vi "Omniax_mDrive_XYZR_MM_BR_RES_2_NC_GR_pxi_Acc.vi"() -> ()   [LabVIEW 2009]
uses:
  <vilib>/Instr/_visa.llb/VISA Configure Serial Port (Instr).vi
panel:
  out "XY Graph 2":cluster{"Y":dbl[], "Y":dbl[]}[](graph)
  out "XY Graph":cluster{"Y":dbl[], "Y":dbl[]}[](graph)
  out "X Scan Duration":dbl
  out "Y Scan Duration":dbl
  out "Z Scan Duration":dbl
  out "R Scan Duration":dbl
  out "R Backlash steps/sec":i32
  out "R Backlash":i32
  out "R Holding Current %":i32
  out "R Run Current %":i32
  out "R offset deg":dbl
  out "R deg/rev":dbl
  out "R steps/rev":u32
  out "R velocity PV step/sec":i32
  out "R MINPOS":i32=-94296
  out "R MAXPOS":i32=-34296
  out "R COM PORT":refnum<visa-resource-name>="COM5"
  in  "R Scan set":bool
  in  "R Scan Velocity SP deg/sec":dbl
  in  "R Scan Length SP deg":dbl
  in  "R Move Set":bool
  out "Reset R Motor Steps":i32
  in  "Reset R Position deg":dbl
  out "R Velocity MVdeg/sec":dbl
  in  "R Velocity SP deg/sec":dbl
  in  "R Position SP deg":dbl
  out "R Position MV deg":dbl
  out "R Scan velocity MV deg/sec":dbl format="%#_6f"
  out "R Scan length MV deg":dbl
  in  "R Scan Length SP steps":i32 min=0 max=6144000 step=100
  in  "R Scan OK":bool
  in  "R Velocity SP step/sec":i32 min=1 max=20000
  in  "R Scan Velocity SP steps/sec":i32=1 min=1 max=102400 step=1
  in  "R Go":bool
  in  "R Step SP":i32=-20000 min=-6144000 max=0 step=500
  out "R Position deg PV":dbl
  out "R Step PV":i32 max=2000
  out "R Backlash corr":bool
  out "R in Motion":bool
  out "R Scan":bool
  out "R in Range":bool
  out "Z COM PORT":refnum<visa-resource-name>="COM5"
  out "Z Backlash steps/sec":i32
  out "Z Backlash":i32
  out "Z Holding Current %":i32
  out "Z Run Current %":i32
  out "Z offset mm":dbl
  out "Z mm/rev":dbl
  out "Z steps/rev":u32
  out "Z  velocity PV step/sec":i32
  out "Z MINPOS":i32=-94296
  out "Z MAXPOS":i32=-34296
  in  "Z Scan set":bool
  in  "Z Scan Velocity SP mm/sec":dbl
  in  "Z Scan Length SP mm":dbl
  in  "Z Move Set":bool
  out "Reset Z Motor Steps":i32
  in  "Reset Z Position mm":dbl
  out "Z Velocity MV mm/sec":dbl
  in  "Z Velocity SP mm/sec":dbl
  in  "Z Position SP mm":dbl
  out "Z Position MV mm":dbl
  out "Z Scan velocity MV mm/sec":dbl format="%#_6f"
  out "Z Scan length MV mm":dbl
  in  "Z Scan Length SP steps":i32 min=0 max=2048000 step=100
  in  "Z Scan OK":bool
  in  "Z Velocity SP step/sec":i32 min=1 max=204800
  in  "Z Scan Velocity SP steps/sec":i32=1 min=1 max=102400 step=1
  in  "Z Go":bool
  in  "Z Step SP":i32=-20000 min=0 max=102400000 step=500
  out "Z Position mm PV":dbl
  out "Z Step PV":i32 max=2000
  out "Z Backlash corr":bool
  out "Z in Motion":bool
  out "Z Scan":bool
  out "Z in Range":bool
  out "Reset X Motor Steps":i32
  in  "Reset X Position mm":dbl
  out "X Backlash corr":bool
  out "X  in Motion":bool
  out "X Scan":bool
  out "X  in Range":bool
  out "X Step PV":i32 max=2000
  out "X Position mm PV":dbl
  out "X velocity PV step/sec":i32
  in  "X Scan set":bool
  in  "X Scan Velocity SP mm/sec":dbl
  in  "X Scan Length SP mm":dbl
  in  "X Move Set":bool
  out "X Velocity MV mm/sec":dbl
  in  "X Velocity SP mm/sec":dbl
  in  "X Position SP mm":dbl
  out "X Position MV mm":dbl
  out "X Scan velocity MV mm/sec":dbl format="%#_6f"
  out "X Scan length MV mm":dbl
  in  "X Scan Length SP steps":i32 min=-2304000 max=2304000 step=100
  in  "X Scan OK":bool
  in  "X Velocity SP step/sec":i32 min=1 max=25600
  in  "X Scan Velocity SP steps/sec":i32=1 min=1 max=102400 step=1
  in  "X Go":bool
  in  "X Step SP":i32=-20000 min=-2304000 max=2304000 step=500
  out "X Backlash steps/sec":i32
  out "X Backlash":i32
  out "X Holding Current %":i32
  out "X Run Current %":i32
  out "X offset mm":dbl
  out "X mm/rev":dbl
  out "X steps/rev":u32
  out "X MAXPOS":i32=-34296
  out "X MINPOS":i32=-94296
  out "X COM PORT":refnum<visa-resource-name>="COM5"
  out "Y Backlash corr":bool
  in  "Y Scan set":bool
  in  "Y Scan Velocity SP mm/sec":dbl
  in  "Y Scan Length SP mm":dbl
  in  "Y Move Set":bool
  out "Y Backlash steps/sec":i32
  out "Y Backlash":i32
  out "Y in Motion":bool
  in  "Reset":bool
  out "Reset Y Motor Steps":i32
  in  "Reset Y Position mm":dbl
  out "Y Velocity MV mm/sec":dbl
  in  "Y Velocity SP mm/sec":dbl
  in  "Y Position SP mm":dbl
  out "Y Position MV mm":dbl
  out "Y Holding Current %":i32
  out "Y Run Current %":i32
  out "Y Scan velocity MV mm/sec":dbl format="%#_6f"
  out "Y Scan length MV mm":dbl
  in  "Scan Cancel":bool
  out "Y Position mm PV":dbl
  out "Y offset mm":dbl
  out "Y mm/rev":dbl
  out "Y steps/rev":u32
  out "Y velocity PV step/sec":i32
  in  "Y Scan Length SP steps":i32 min=-2304000 max=2304000 step=100
  out "Y Scan":bool
  in  "Y Scan OK":bool
  in  "Scan Go":bool
  in  "Y Velocity SP step/sec":i32 min=1 max=25600
  in  "Y Scan Velocity SP steps/sec":i32=1 min=1 max=102400 step=1
  in  "Stop":bool
  out "Y in Range":bool
  out "Y Step PV":i32 max=2000
  in  "Y Go":bool
  in  "Y Step SP":i32=-20000 min=-2304000 max=2304000 step=500
  out "Y MINPOS":i32=-94296
  out "Y MAXPOS":i32=-34296
  out "Y COM PORT":refnum<visa-resource-name>="COM5"
  # "L"
  # "M"
  # "B"
  # "S"
  # "MX"
  # "MY"
  # "MZ"
  # "MR"
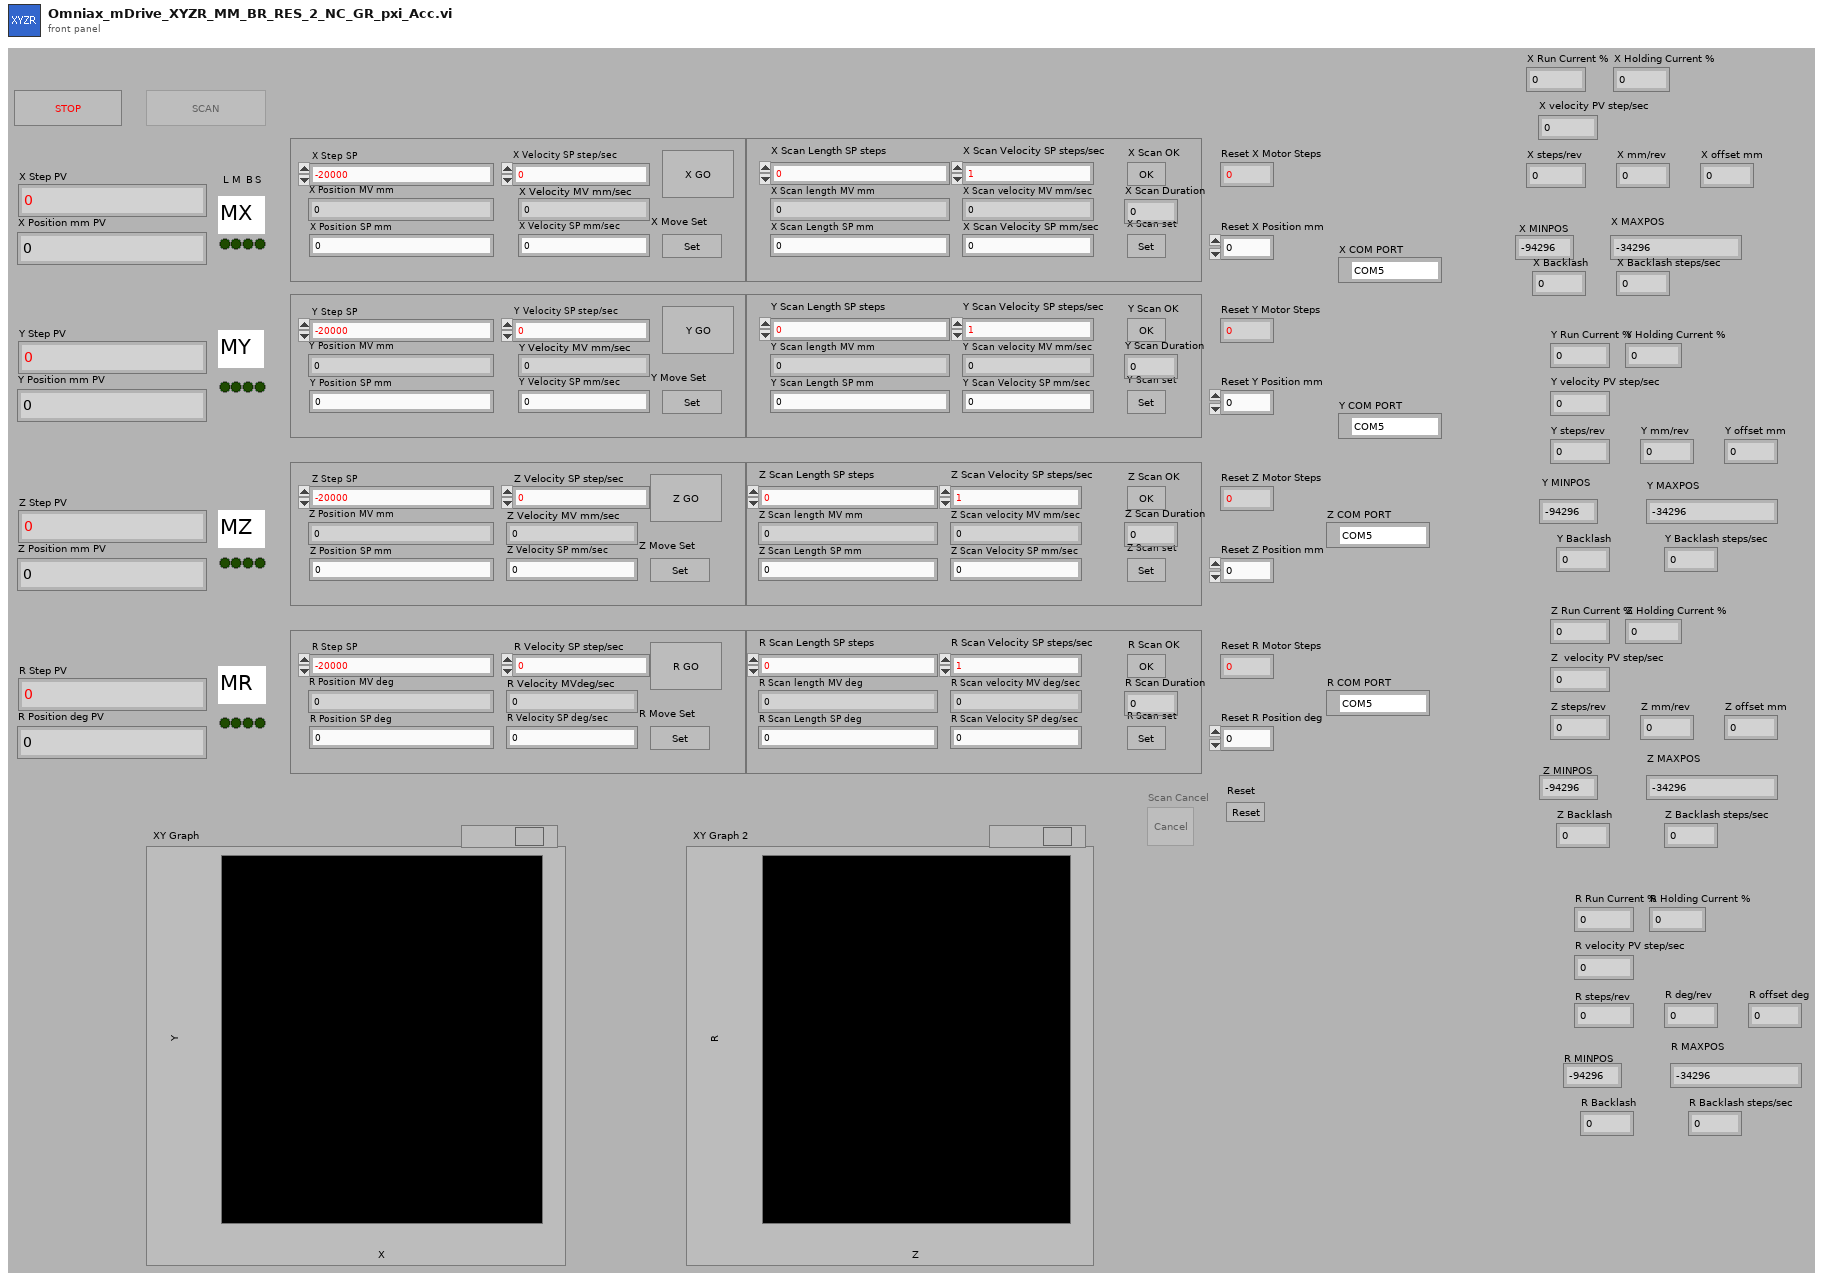
[diagram p1: front panel]
types:
  T1 = enum8{"Enabled", "Disabled", "Disabled and Grayed Out"}
  T2 = enum16{"Stop", "Reset", "Run Current", "Holding Current", "Accel Rate", "Decel Rate", "Move to Relative Position", "Move to Absolute Position", "Echo Mode", "Print Parameter", "Send String", "Microstep Resolution", "Set Current Position", "Max Velocity"}
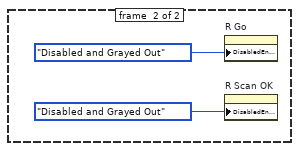
[diagram p2: hidden frame]
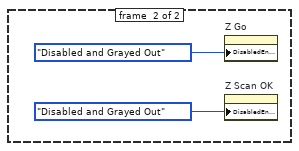
[diagram p5: hidden frame]
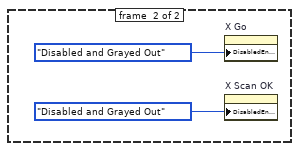
[diagram p8: hidden frame]
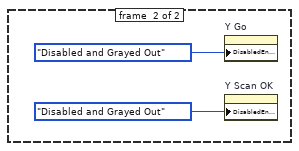
[diagram p11: hidden frame]
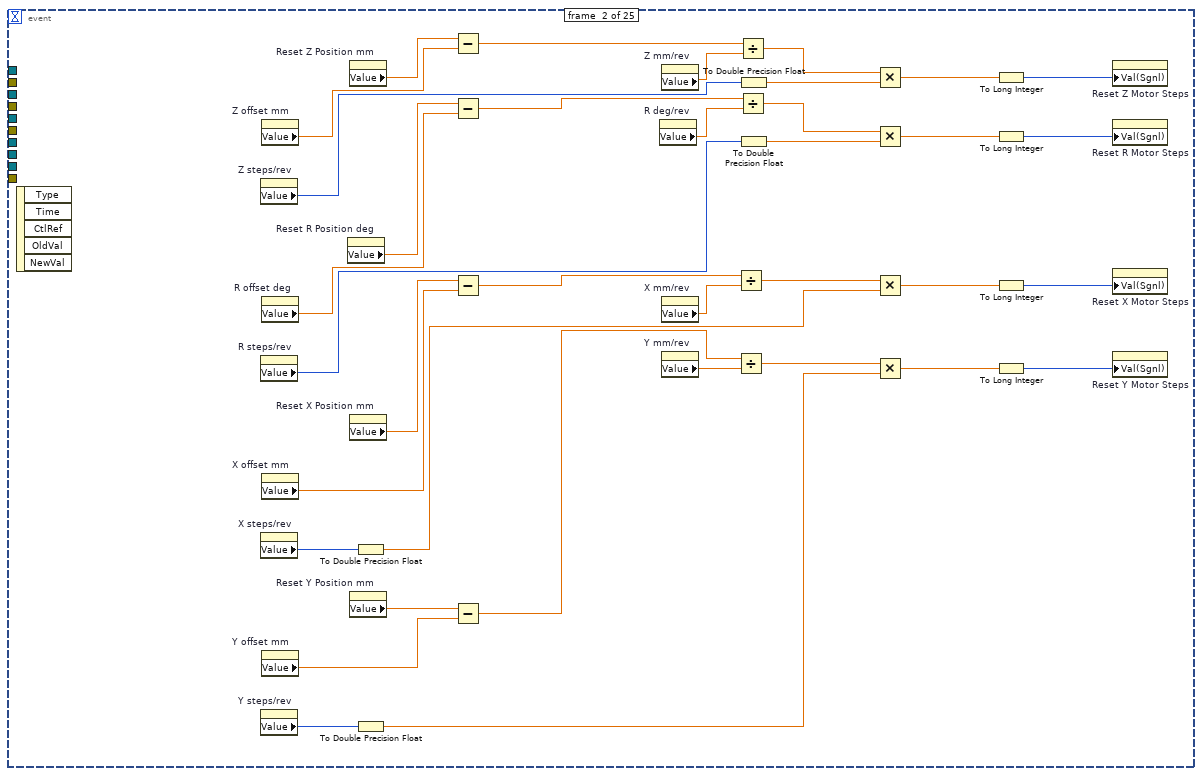
[diagram p14: hidden frame]
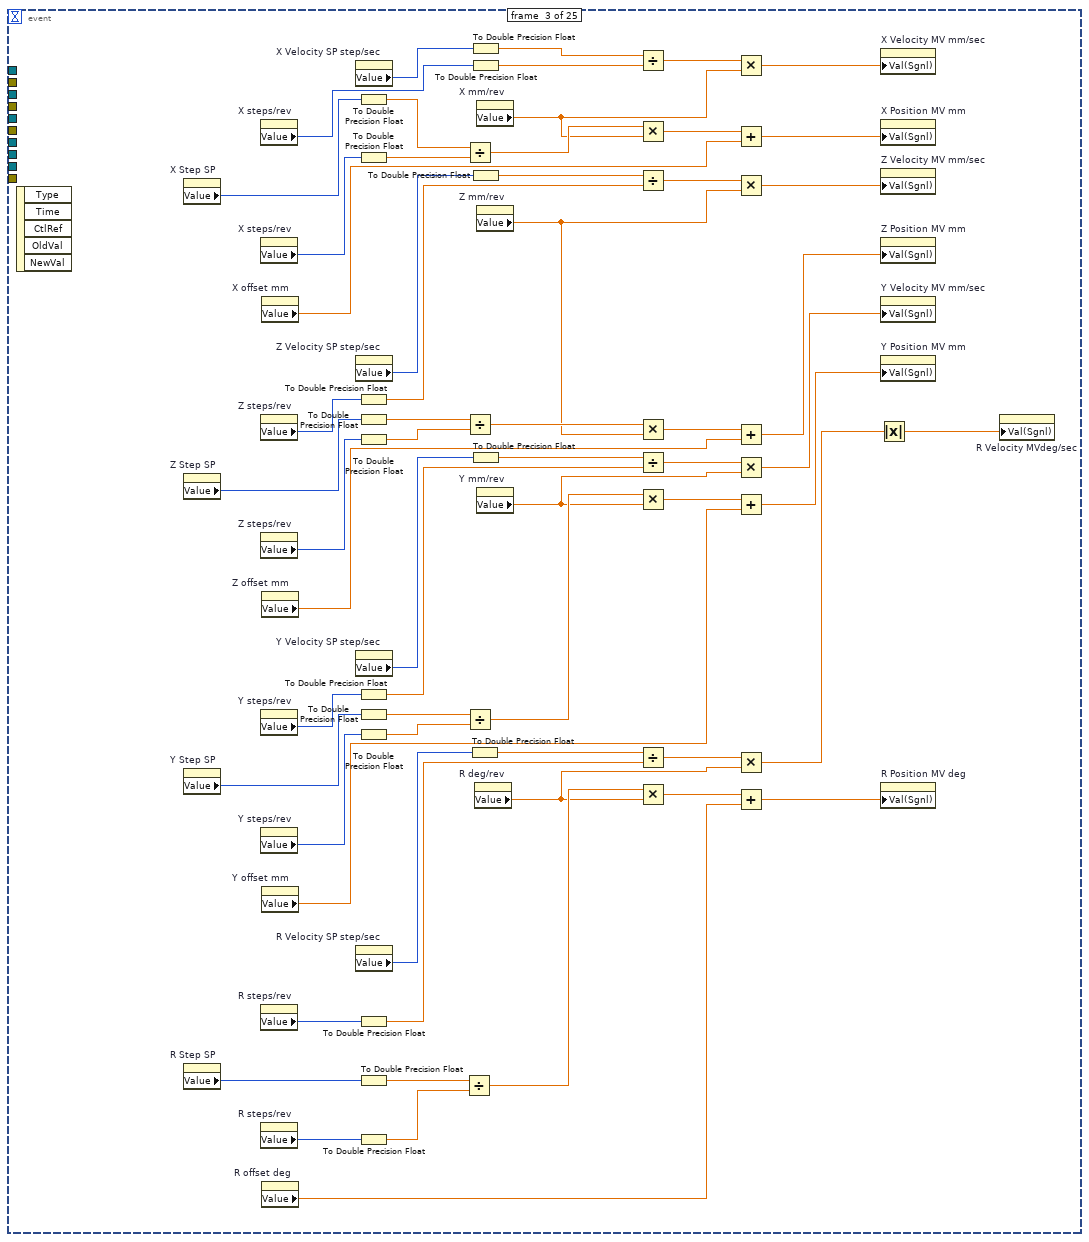
[diagram p15: hidden frame]
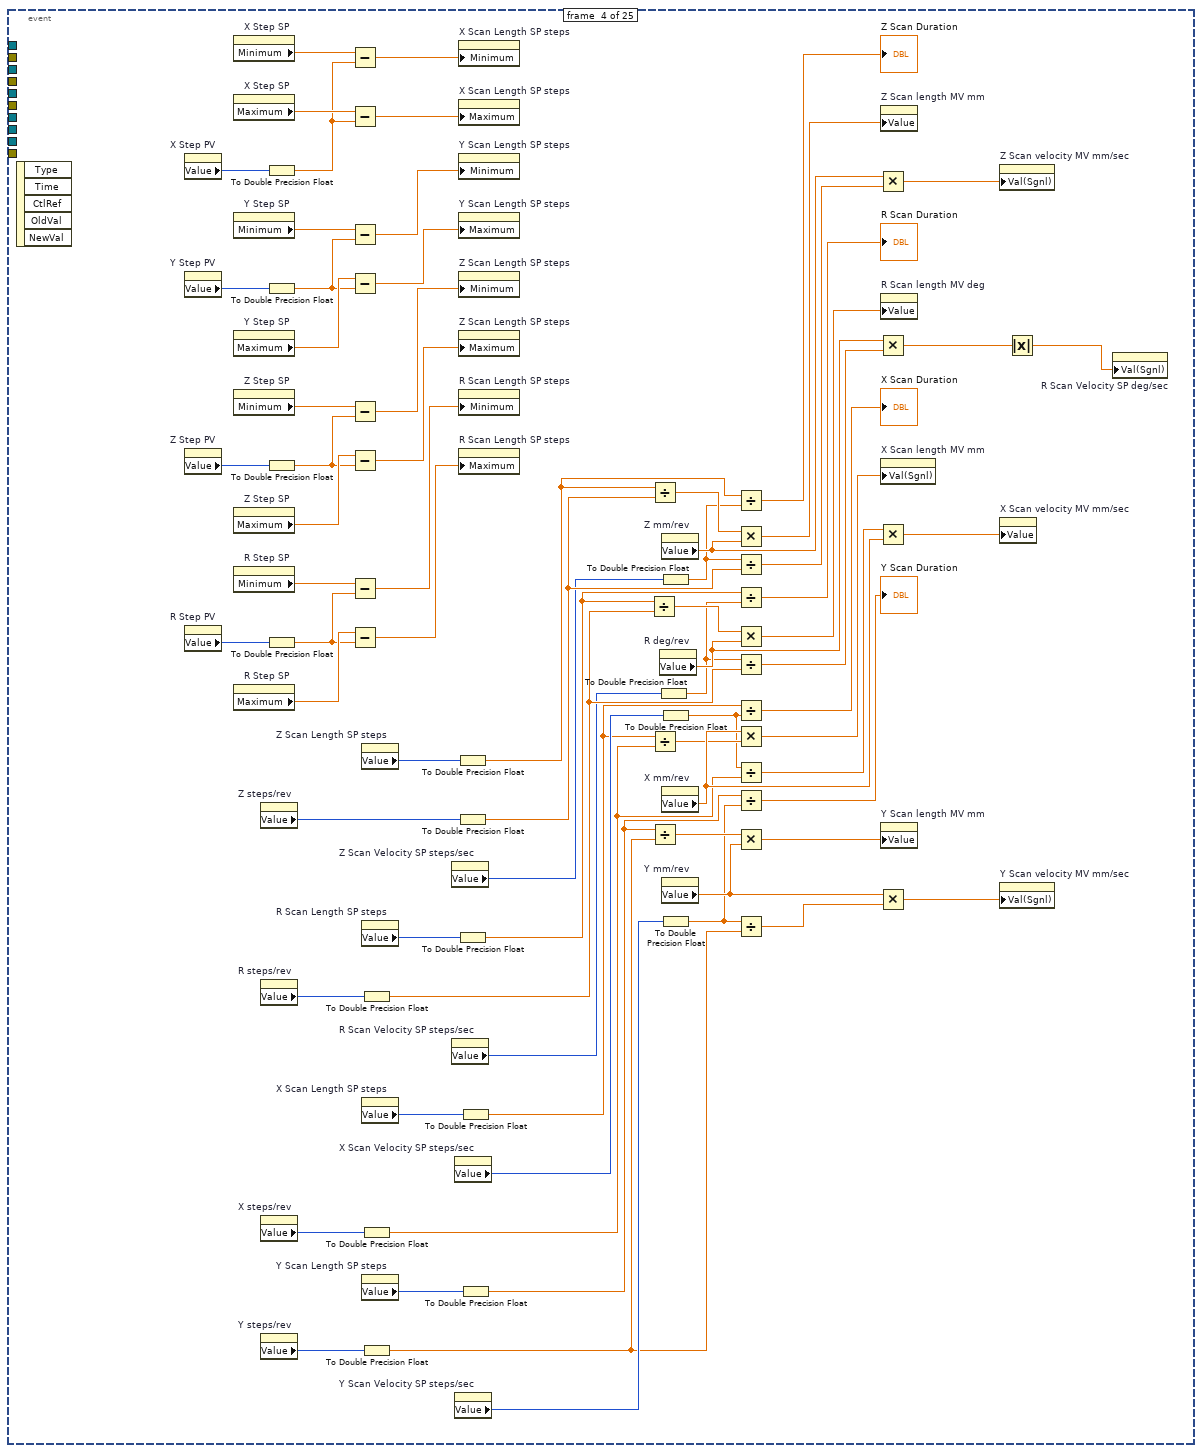
[diagram p16: hidden frame]
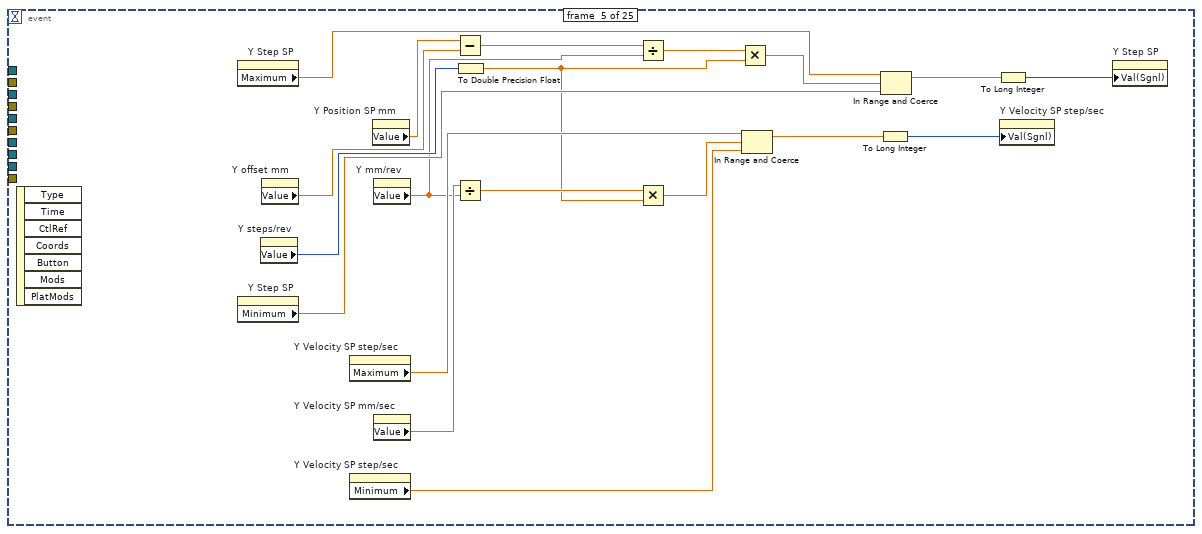
[diagram p17: hidden frame]
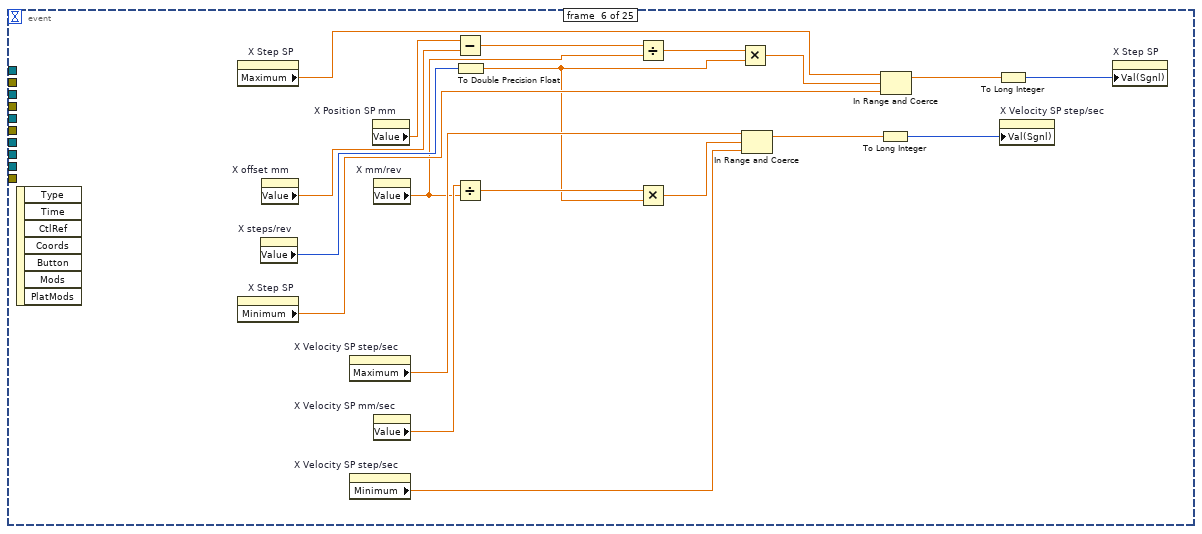
[diagram p18: hidden frame]
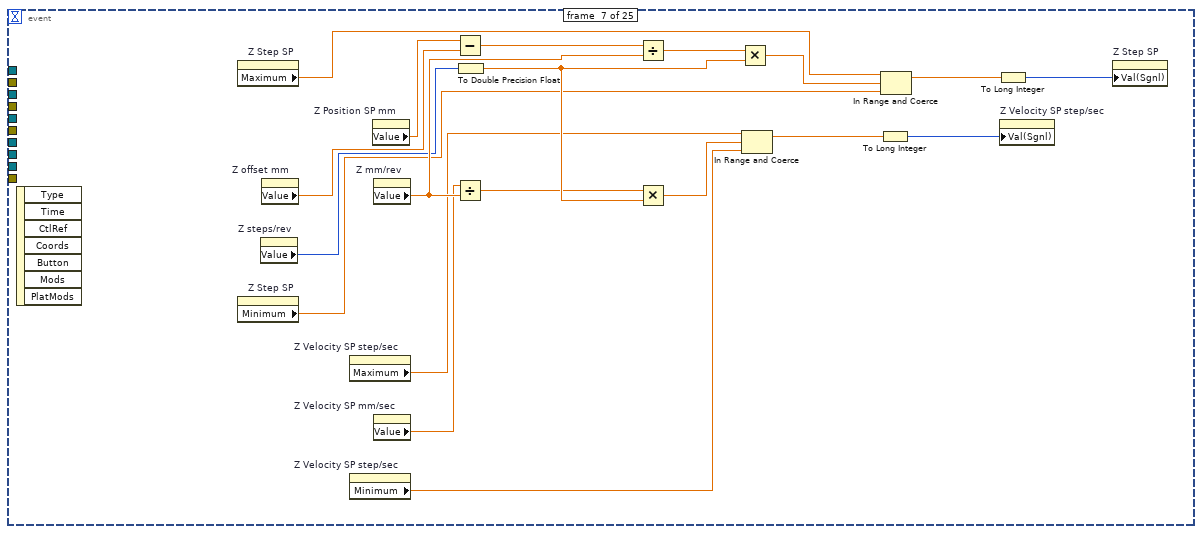
[diagram p19: hidden frame]
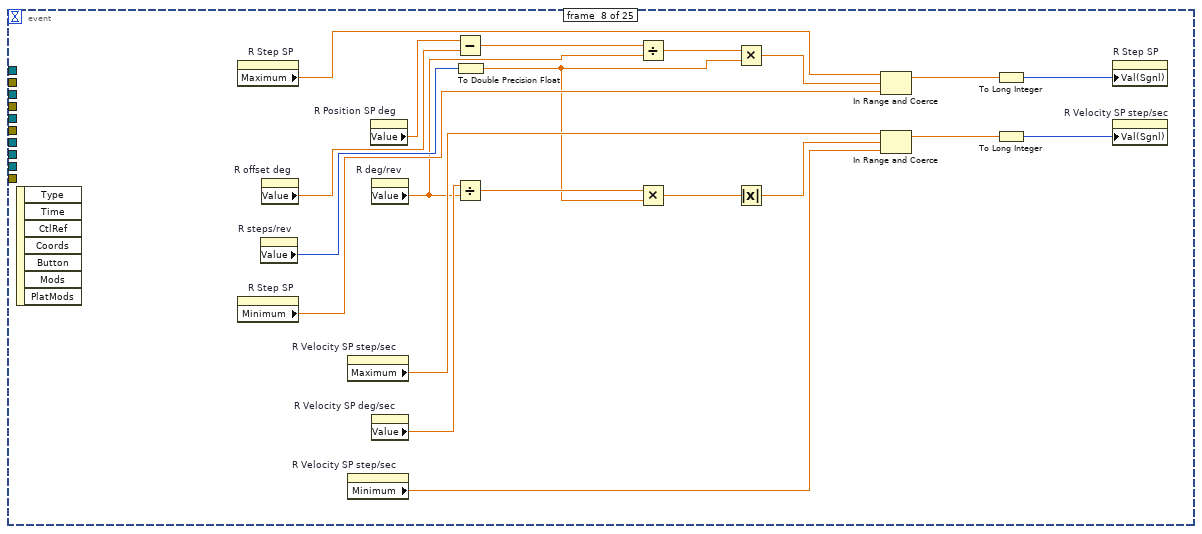
[diagram p20: hidden frame]
diagram:
  w29 = refnum<visa-resource-name> "COM7" ("COM PORT")
  w31 = u16 0 items=["None", "XON/XOFF", "RTS/CTS", "XON/XOFF & RTS/CTS", "DTR/DSR", "XON/XOFF & DTR/DSR"] ("flow control (0:none)")
  w32 = u16 10 items=["1.0"=10, "1.5"=15, "2.0"=20] ("stop bits (10: 1 bit)")
  w62 = refnum<visa-resource-name> "COM6" ("COM PORT")
  w64 = u16 0 items=["None", "XON/XOFF", "RTS/CTS", "XON/XOFF & RTS/CTS", "DTR/DSR", "XON/XOFF & DTR/DSR"] ("flow control (0:none)")
  w65 = u16 10 items=["1.0"=10, "1.5"=15, "2.0"=20] ("stop bits (10: 1 bit)")
  w75 = refnum<visa-resource-name> "COM4" ("COM PORT")
  w77 = u16 0 items=["None", "XON/XOFF", "RTS/CTS", "XON/XOFF & RTS/CTS", "DTR/DSR", "XON/XOFF & DTR/DSR"] ("flow control (0:none)")
  w78 = u16 10 items=["1.0"=10, "1.5"=15, "2.0"=20] ("stop bits (10: 1 bit)")
  w100 = refnum<visa-resource-name> "COM5" ("COM PORT")
  w102 = u16 0 items=["None", "XON/XOFF", "RTS/CTS", "XON/XOFF & RTS/CTS", "DTR/DSR", "XON/XOFF & DTR/DSR"] ("flow control (0:none)")
  w103 = u16 10 items=["1.0"=10, "1.5"=15, "2.0"=20] ("stop bits (10: 1 bit)")
  # "Stop bits"
  # "Stop bits"
  # "Stop bits"
  # "Stop bits"
  n1 = flat-sequence {
    frame #0 {
      w112 = -3.0 ("R deg/rev")
      w110 = u32 51200 ("step/rev")
      w114 = 20000 ("Value (Signaling)")
      n2 = To Double Precision Float(number=w114) -> (double precision float=w116:dbl)
      n3 = To Double Precision Float(number=w110) -> (double precision float=w111:dbl)
      n4 = property on="R Velocity SP step/sec" class="DigNum (strict)"("Val(Sgnl)"=w114) -> ()  [unwired: 2 in, 2 out]
      n5 = property on="R Velocity SP step/sec" class="DigNum (strict)"("Minimum"=1.0 ("Data Entry Limits:Minimum")) -> ()  [unwired: 2 in, 2 out]
      n6 = Divide(x=w116, y=w111) -> (x/y=w115:dbl)
      n7 = property on="R Velocity SP step/sec" class="DigNum (strict)"("Maximum"=w116) -> ()  [unwired: 2 in, 2 out]
      n8 = Multiply(x=w115, y=w112) -> (x*y=w113:dbl)
      n9 = Absolute Value(x=w113) -> (abs(x)=w107:dbl)
      n10 = property on="R Velocity SP deg/sec" class="DigNum (strict)"("Val(Sgnl)"=w107) -> ()  [unwired: 2 in, 2 out]
      "R offset deg" <- 0.0 ("R offset deg")
      "R deg/rev" <- w112
      "R steps/rev" <- w110
    }
  }
  n11 = flat-sequence {
    frame #0 {
      w118 = 0.2 ("Z mm/rev")
      w117 = u32 51200 ("step/rev")
      w119 = 204800 ("Value (Signaling)")
      n12 = To Double Precision Float(number=w119) -> (double precision float=w123:dbl)
      n13 = To Double Precision Float(number=w117) -> (double precision float=w122:dbl)
      n14 = property on="Z Velocity SP step/sec" class="DigNum (strict)"("Val(Sgnl)"=w119) -> ()  [unwired: 2 in, 2 out]
      n15 = property on="Z Velocity SP step/sec" class="DigNum (strict)"("Minimum"=1.0 ("Data Entry Limits:Minimum")) -> ()  [unwired: 2 in, 2 out]
      n16 = Divide(x=w123, y=w122) -> (x/y=w120:dbl)
      n17 = property on="Z Velocity SP step/sec" class="DigNum (strict)"("Maximum"=w123) -> ()  [unwired: 2 in, 2 out]
      n18 = Multiply(x=w120, y=w118) -> (x*y=w121:dbl)
      n19 = property on="Z Velocity SP mm/sec" class="DigNum (strict)"("Val(Sgnl)"=w121) -> ()  [unwired: 2 in, 2 out]
      "Z offset mm" <- 0.0 ("Z offset mm")
      "Z mm/rev" <- w118
      "Z steps/rev" <- w117
    }
  }
  n20 = flat-sequence {
    frame #0 {
      n21 = property on="X Backlash corr" class="Bool (strict)"("Val(Sgnl)"=FALSE ("Value (Signaling)")) -> ()  [unwired: 2 in, 2 out]
      n22 = property on="R Backlash corr" class="Bool (strict)"("Val(Sgnl)"=FALSE ("Value (Signaling)")) -> ()  [unwired: 2 in, 2 out]
      n23 = property on="Z Backlash corr" class="Bool (strict)"("Val(Sgnl)"=FALSE ("Value (Signaling)")) -> ()  [unwired: 2 in, 2 out]
      n24 = property on="Y Backlash corr" class="Bool (strict)"("Val(Sgnl)"=FALSE ("Value (Signaling)")) -> ()  [unwired: 2 in, 2 out]
      "Z Backlash steps/sec" <- 25600 ("Z Backlash steps/sec")
      "Z Backlash" <- -12800 ("Z Backlash")
      "X Backlash steps/sec" <- 25600 ("Value (Signaling)")
      "X Backlash" <- -5120 ("Backlash2")
      "Y Backlash" <- -5120 ("Backlash2")
      "Y Backlash steps/sec" <- 25600 ("Value (Signaling)")
      "R Backlash steps/sec" <- 6400 ("R Backlash steps/sec")
      "R Backlash" <- -12800 ("R Backlash")
    }
  }
  n25 = flat-sequence {
    frame #0 {
      "Z Holding Current %" <- 20 ("Z Holding Current %")
      "Z Run Current %" <- 40 ("Z Run Current %")
      "X Run Current %" <- 40 ("Run Current %")
      "X Holding Current %" <- 20 ("Holding Current %")
      "Y Run Current %" <- 40 ("Run Current %")
      "Y Holding Current %" <- 20 ("Holding Current %")
      "R Holding Current %" <- 20 ("R Holding Current %")
      "R Run Current %" <- 100 ("R Run Current %")
    }
  }
  n26 = flat-sequence {
    frame #0 {
      n27 = property on="Y Scan" class="Bool (strict)"("Val(Sgnl)"=FALSE ("Value (Signaling)")) -> ()  [unwired: 2 in, 2 out]
      n28 = property on="R Velocity SP deg/sec" class="DigNum (strict)"("Val(Sgnl)"=0.1 ("Value (Signaling)")) -> ()  [unwired: 2 in, 2 out]
      n29 = property on="X Scan Velocity SP mm/sec" class="DigNum (strict)"("Val(Sgnl)"=0.1 ("Value (Signaling)")) -> ()  [unwired: 2 in, 2 out]
      n30 = property on="Z Scan" class="Bool (strict)"("Val(Sgnl)"=FALSE ("Value (Signaling)")) -> ()  [unwired: 2 in, 2 out]
      n31 = property on="X Scan" class="Bool (strict)"("Val(Sgnl)"=FALSE ("Value (Signaling)")) -> ()  [unwired: 2 in, 2 out]
      n32 = property on="Z Scan Velocity SP mm/sec" class="DigNum (strict)"("Val(Sgnl)"=0.1 ("Value (Signaling)")) -> ()  [unwired: 2 in, 2 out]
      n33 = property on="R Scan" class="Bool (strict)"("Val(Sgnl)"=FALSE ("Value (Signaling)")) -> ()  [unwired: 2 in, 2 out]
      n34 = property on="Y Scan Velocity SP mm/sec" class="DigNum (strict)"("Val(Sgnl)"=0.1 ("Value (Signaling)")) -> ()  [unwired: 2 in, 2 out]
      n35 = property on="Scan Cancel" class="Bool"("DisabledEnum"=T1."Disabled and Grayed Out" ("Disabled")) -> ()  [unwired: 2 in, 2 out]
      n36 = property on="Scan Go" class="Bool"("DisabledEnum"=T1."Disabled and Grayed Out" ("Disabled")) -> ()  [unwired: 2 in, 2 out]
    }
  }
  n37 = flat-sequence {
    frame #0 {
      w158 = 0.2 ("MM/rev")
      w161 = u32 51200 ("step/rev")
      w156 = 25600 ("Value (Signaling)")
      # "a=1000000"
      n38 = To Double Precision Float(number=w156) -> (double precision float=w162:dbl)
      n39 = To Double Precision Float(number=w161) -> (double precision float=w160:dbl)
      n40 = property on="X Velocity SP step/sec" class="DigNum (strict)"("Minimum"=1.0 ("Data Entry Limits:Minimum")) -> ()  [unwired: 2 in, 2 out]
      n41 = property on="X Velocity SP step/sec" class="DigNum (strict)"("Val(Sgnl)"=w156) -> ()  [unwired: 2 in, 2 out]
      n42 = Divide(x=w162, y=w160) -> (x/y=w157:dbl)
      n43 = property on="X Velocity SP step/sec" class="DigNum (strict)"("Maximum"=w162) -> ()  [unwired: 2 in, 2 out]
      n44 = Multiply(x=w157, y=w158) -> (x*y=w159:dbl)
      n45 = property on="X Velocity SP mm/sec" class="DigNum (strict)"("Val(Sgnl)"=w159) -> ()  [unwired: 2 in, 2 out]
      "X offset mm" <- 0.0 ("offset")
      "X steps/rev" <- w161
      "X mm/rev" <- w158
    }
  }
  n46 = flat-sequence {
    frame #0 {
      w167 = 0.2 ("MM/rev")
      w170 = u32 51200 ("step/rev")
      w165 = 25600 ("Value (Signaling)")
      n47 = To Double Precision Float(number=w165) -> (double precision float=w171:dbl)
      n48 = To Double Precision Float(number=w170) -> (double precision float=w169:dbl)
      n49 = property on="Y Velocity SP step/sec" class="DigNum (strict)"("Minimum"=1.0 ("Data Entry Limits:Minimum")) -> ()  [unwired: 2 in, 2 out]
      n50 = property on="Y Velocity SP step/sec" class="DigNum (strict)"("Val(Sgnl)"=w165) -> ()  [unwired: 2 in, 2 out]
      n51 = Divide(x=w171, y=w169) -> (x/y=w166:dbl)
      n52 = property on="Y Velocity SP step/sec" class="DigNum (strict)"("Maximum"=w171) -> ()  [unwired: 2 in, 2 out]
      n53 = Multiply(x=w166, y=w167) -> (x*y=w168:dbl)
      n54 = property on="Y Velocity SP mm/sec" class="DigNum (strict)"("Val(Sgnl)"=w168) -> ()  [unwired: 2 in, 2 out]
      "Y offset mm" <- 0.0 ("offset")
      "Y steps/rev" <- w170
      "Y mm/rev" <- w167
    }
  }
  n55 = call-poly "VISA Configure Serial Port"("VISA resource name"=w100, "timeout (10sec)"=u32 10000, "baud rate (9600)"=u32 9600, "data bits (8)"=u16 8, "parity (0:none)"=enum16{"None", "Odd", "Even", "Mark", "Space"}."None", "stop bits (10: 1 bit)"=w103, "flow control (0:none)"=w102) -> ("VISA resource name out"=w93:refnum<visa-resource-name>, "error out"=w92:errorcluster)  [unwired: 7 in]
  n56 = flat-sequence {
    tunnel: w92 -> [w175]
    tunnel: w93 -> [w177]
    tunnel: [w176] -> w10
    tunnel: [w174] -> w8
    tunnel: w10 -> [w183]
    tunnel: [w184] -> w9
    tunnel: w8 -> [w180]
    tunnel: [w182] -> w7
    tunnel: [w193] -> w91
    tunnel: [w195] -> w89
    tunnel: w9 -> [w194]
    tunnel: w7 -> [w196]
    tunnel: w91 -> [w203]
    tunnel: [w202] -> w90
    tunnel: w89 -> [w200]
    tunnel: [w201] -> w88
    tunnel: [w213] -> w95
    tunnel: [w214] -> w94
    tunnel: w90 -> [w212]
    tunnel: w88 -> [w211]
    tunnel: w95 -> [w224]
    tunnel: w94 -> [w223]
    tunnel: [w226] -> w61
    tunnel: [w225] -> w60
    tunnel: [w220] -> w59
    tunnel: [w231] -> w98
    tunnel: [w232] -> w99
    tunnel: w61 -> [w232]
    tunnel: w60 -> [w231]
    tunnel: w59 -> [w227]
    frame #0 {
      n57 = call "mDrive Send Command.vi"("error in (no error)"=w175, "Extra"="EM=2", "Command"=T2."Send String", "VISA resource name"=w177) -> ("error out"=w174:errorcluster, "VISA resource name out"=w176:refnum<visa-resource-name>)  [unwired: 3 in, 1 out]
    }
    frame #1 {
      n58 = Number To Decimal String(number=1000000) -> (decimal integer string=w185:string)  [unwired: 1 in]
      n59 = call "mDrive Send Command.vi"("error in (no error)"=w180, "Extra"=w185, "Command"=T2."Accel Rate", "VISA resource name"=w183) -> ("error out"=w181:errorcluster, "VISA resource name out"=w189:refnum<visa-resource-name>)  [unwired: 3 in, 1 out]
      n60 = call "mDrive Send Command.vi"("error in (no error)"=w181, "Extra"=w185, "Command"=T2."Decel Rate", "VISA resource name"=w189) -> ("error out"=w182:errorcluster, "VISA resource name out"=w184:refnum<visa-resource-name>)  [unwired: 3 in, 1 out]
    }
    frame #2 {
      # "Run Current %"
      n61 = property on="Y Run Current %" class="DigNum (strict)"() -> ("Value"=w191:i32)  [unwired: 2 in, 2 out]
      n62 = Number To Decimal String(number=w191) -> (decimal integer string=w192:string)  [unwired: 1 in]
      n63 = call "mDrive Send Command.vi"("error in (no error)"=w196, "Extra"=w192, "Command"=T2."Run Current", "VISA resource name"=w194) -> ("error out"=w195:errorcluster, "VISA resource name out"=w193:refnum<visa-resource-name>)  [unwired: 3 in, 1 out]
    }
    frame #3 {
      # "Holding Current %"
      n64 = property on="Y Holding Current %" class="DigNum (strict)"() -> ("Value"=w198:i32)  [unwired: 2 in, 2 out]
      n65 = Number To Decimal String(number=w198) -> (decimal integer string=w199:string)  [unwired: 1 in]
      n66 = call "mDrive Send Command.vi"("error in (no error)"=w200, "Extra"=w199, "Command"=T2."Holding Current", "VISA resource name"=w203) -> ("error out"=w201:errorcluster, "VISA resource name out"=w202:refnum<visa-resource-name>)  [unwired: 3 in, 1 out]
    }
    frame #4 {
      # "Print Velocity Ma"
      # "Velocity Max"
      n67 = property on="Y Velocity SP step/sec" class="DigNum (strict)"() -> ("Value"=w210:i32)  [unwired: 2 in, 2 out]
      n68 = Number To Decimal String(number=w210) -> (decimal integer string=w209:string)  [unwired: 1 in]
      n69 = call "mDrive Send Command.vi"("error in (no error)"=w211, "Extra"=w209, "Command"=T2."Max Velocity", "VISA resource name"=w212) -> ("error out"=w207:errorcluster, "VISA resource name out"=w217:refnum<visa-resource-name>)  [unwired: 3 in, 1 out]
      n70 = call "mDrive Send Command.vi"("error in (no error)"=w207, "Extra"="VM", "Command"=T2."Print Parameter", "VISA resource name"=w217) -> ("error out"=w214:errorcluster, "read buffer"=w215:string, "VISA resource name out"=w213:refnum<visa-resource-name>)  [unwired: 3 in]
      n71 = Decimal String To Number(string=w215, offset=0) -> (number=w208:i32)  [unwired: 1 in, 1 out]
      n72 = property on="Y scan velocity MV step/sec" class="DigNum (strict)"("Val(Sgnl)"=w208) -> ()  [unwired: 2 in, 2 out]
    }
    frame #5 {
      # "PRINT POSITION"
      n73 = call "mDrive Send Command.vi"("error in (no error)"=w223, "Extra"="P", "Command"=T2."Print Parameter", "VISA resource name"=w224) -> ("error out"=w225:errorcluster, "read buffer"=w222:string, "VISA resource name out"=w226:refnum<visa-resource-name>)  [unwired: 3 in]
      n74 = Decimal String To Number(string=w222, offset=0) -> (number=w220:i32)  [unwired: 1 in, 1 out]
    }
    frame #6 {
      w229 = -2304000 ("lower limit")
      w230 = 2304000 ("upper limit")
      n75 = property on="Y Step SP" class="DigNum (strict)"("Val(Sgnl)"=w227) -> ()  [unwired: 2 in, 2 out]
      n76 = property on="Y Step SP" class="DigNum (strict)"("Maximum"=w230) -> ()  [unwired: 2 in, 2 out]
      n77 = In Range and Coerce(upper limit=w230, x=w227, lower limit=w229) -> (In Range?=w228:bool)  [unwired: 1 out]
      n78 = property on="Y Step SP" class="DigNum (strict)"("Minimum"=w229) -> ()  [unwired: 2 in, 2 out]
      n79 = property on="Y in Range" class="Bool (strict)"("Val(Sgnl)"=w228) -> ()  [unwired: 2 in, 2 out]
      "Y MINPOS" <- w229
      "Y MAXPOS" <- w230
    }
  }
  n80 = call-poly "VISA Configure Serial Port"("VISA resource name"=w75, "timeout (10sec)"=u32 10000, "baud rate (9600)"=u32 9600, "data bits (8)"=u16 8, "parity (0:none)"=enum16{"None", "Odd", "Even", "Mark", "Space"}."None", "stop bits (10: 1 bit)"=w78, "flow control (0:none)"=w77) -> ("VISA resource name out"=w74:refnum<visa-resource-name>, "error out"=w73:errorcluster)  [unwired: 7 in]
  n81 = call-poly "VISA Configure Serial Port"("VISA resource name"=w29, "timeout (10sec)"=u32 10000, "baud rate (9600)"=u32 9600, "data bits (8)"=u16 8, "parity (0:none)"=enum16{"None", "Odd", "Even", "Mark", "Space"}."None", "stop bits (10: 1 bit)"=w32, "flow control (0:none)"=w31) -> ("VISA resource name out"=w28:refnum<visa-resource-name>, "error out"=w27:errorcluster)  [unwired: 7 in]
  n82 = call-poly "VISA Configure Serial Port"("VISA resource name"=w62, "timeout (10sec)"=u32 10000, "baud rate (9600)"=u32 9600, "data bits (8)"=u16 8, "parity (0:none)"=enum16{"None", "Odd", "Even", "Mark", "Space"}."None", "stop bits (10: 1 bit)"=w65, "flow control (0:none)"=w64) -> ("VISA resource name out"=w46:refnum<visa-resource-name>, "error out"=w45:errorcluster)  [unwired: 7 in]
  n83 = flat-sequence {
    tunnel: w45 -> [w233]
    tunnel: w46 -> [w236]
    tunnel: [w235] -> w6
    tunnel: [w234] -> w4
    tunnel: w6 -> [w246]
    tunnel: [w241] -> w5
    tunnel: w4 -> [w245]
    tunnel: [w245] -> w3
    tunnel: [w250] -> w55
    tunnel: [w252] -> w54
    tunnel: w5 -> [w251]
    tunnel: w3 -> [w253]
    tunnel: w55 -> [w260]
    tunnel: [w259] -> w53
    tunnel: w54 -> [w257]
    tunnel: [w258] -> w52
    tunnel: [w270] -> w51
    tunnel: [w271] -> w50
    tunnel: w53 -> [w269]
    tunnel: w52 -> [w268]
    tunnel: w51 -> [w281]
    tunnel: w50 -> [w280]
    tunnel: [w283] -> w49
    tunnel: [w282] -> w48
    tunnel: [w277] -> w47
    tunnel: [w290] -> w25
    tunnel: [w291] -> w26
    tunnel: w49 -> [w291]
    tunnel: w48 -> [w290]
    tunnel: w47 -> [w288]
    frame #0 {
      n84 = call "mDrive Send Command.vi"("error in (no error)"=w233, "Extra"="EM=2", "Command"=T2."Send String", "VISA resource name"=w236) -> ("error out"=w234:errorcluster, "VISA resource name out"=w235:refnum<visa-resource-name>)  [unwired: 3 in, 1 out]
    }
    frame #1 {
      n85 = Number To Decimal String(number=1000000) -> (decimal integer string=w239:string)  [unwired: 1 in]
      n86 = call "mDrive Send Command.vi"("Extra"=w239, "Command"=T2."Accel Rate", "VISA resource name"=w246) -> ("VISA resource name out"=w244:refnum<visa-resource-name>)  [unwired: 4 in, 2 out]
      n87 = call "mDrive Send Command.vi"("Extra"=w239, "Command"=T2."Decel Rate", "VISA resource name"=w244) -> ("VISA resource name out"=w241:refnum<visa-resource-name>)  [unwired: 4 in, 2 out]
    }
    frame #2 {
      # "Run Current %"
      n88 = property on="Z Run Current %" class="DigNum (strict)"() -> ("Value"=w248:i32)  [unwired: 2 in, 2 out]
      n89 = Number To Decimal String(number=w248) -> (decimal integer string=w249:string)  [unwired: 1 in]
      n90 = call "mDrive Send Command.vi"("error in (no error)"=w253, "Extra"=w249, "Command"=T2."Run Current", "VISA resource name"=w251) -> ("error out"=w252:errorcluster, "VISA resource name out"=w250:refnum<visa-resource-name>)  [unwired: 3 in, 1 out]
    }
    frame #3 {
      # "Holding Current %"
      n91 = property on="Z Run Current %" class="DigNum (strict)"() -> ("Value"=w255:i32)  [unwired: 2 in, 2 out]
      n92 = Number To Decimal String(number=w255) -> (decimal integer string=w256:string)  [unwired: 1 in]
      n93 = call "mDrive Send Command.vi"("error in (no error)"=w257, "Extra"=w256, "Command"=T2."Holding Current", "VISA resource name"=w260) -> ("error out"=w258:errorcluster, "VISA resource name out"=w259:refnum<visa-resource-name>)  [unwired: 3 in, 1 out]
    }
    frame #4 {
      # "Print Velocity Ma"
      # "Velocity Max"
      n94 = property on="Z Velocity SP step/sec" class="DigNum (strict)"() -> ("Value"=w267:i32)  [unwired: 2 in, 2 out]
      n95 = Number To Decimal String(number=w267) -> (decimal integer string=w266:string)  [unwired: 1 in]
      n96 = call "mDrive Send Command.vi"("error in (no error)"=w268, "Extra"=w266, "Command"=T2."Max Velocity", "VISA resource name"=w269) -> ("error out"=w264:errorcluster, "VISA resource name out"=w274:refnum<visa-resource-name>)  [unwired: 3 in, 1 out]
      n97 = call "mDrive Send Command.vi"("error in (no error)"=w264, "Extra"="VM", "Command"=T2."Print Parameter", "VISA resource name"=w274) -> ("error out"=w271:errorcluster, "read buffer"=w272:string, "VISA resource name out"=w270:refnum<visa-resource-name>)  [unwired: 3 in]
      n98 = Decimal String To Number(string=w272, offset=0) -> (number=w265:i32)  [unwired: 1 in, 1 out]
      n99 = property on="Z  velocity PV step/sec" class="DigNum (strict)"("Val(Sgnl)"=w265) -> ()  [unwired: 2 in, 2 out]
    }
    frame #5 {
      # "PRINT POSITION"
      n100 = call "mDrive Send Command.vi"("error in (no error)"=w280, "Extra"="P", "Command"=T2."Print Parameter", "VISA resource name"=w281) -> ("error out"=w282:errorcluster, "read buffer"=w279:string, "VISA resource name out"=w283:refnum<visa-resource-name>)  [unwired: 3 in]
      n101 = Decimal String To Number(string=w279, offset=0) -> (number=w277:i32)  [unwired: 1 in, 1 out]
    }
    frame #6 {
      n102 = property on="Z Step SP" class="DigNum (strict)"("Val(Sgnl)"=w288) -> ()  [unwired: 2 in, 2 out]
      n103 = property on="Z Step SP" class="DigNum (strict)"() -> ("Minimum"=w287:dbl)  [unwired: 2 in, 2 out]
      n104 = To Long Integer(number=w287) -> (32bit integer=w284:i32)
      "Z MINPOS" <- w284
      n105 = property on="Z Step SP" class="DigNum (strict)"() -> ("Maximum"=w285:dbl)  [unwired: 2 in, 2 out]
      n106 = To Long Integer(number=w285) -> (32bit integer=w286:i32)
      "Z MAXPOS" <- w286
      n107 = In Range and Coerce(upper limit=w286, x=w288, lower limit=w284) -> (In Range?=w289:bool)  [unwired: 1 out]
      n108 = property on="Z in Range" class="Bool (strict)"("Val(Sgnl)"=w289) -> ()  [unwired: 2 in, 2 out]
    }
  }
  n109 = flat-sequence {
    tunnel: w73 -> [w293]
    tunnel: w74 -> [w295]
    tunnel: [w294] -> w18
    tunnel: [w292] -> w16
    tunnel: w18 -> [w299]
    tunnel: [w298] -> w17
    tunnel: w16 -> [w300]
    tunnel: [w302] -> w15
    tunnel: [w311] -> w87
    tunnel: [w313] -> w86
    tunnel: w17 -> [w312]
    tunnel: w15 -> [w314]
    tunnel: w87 -> [w321]
    tunnel: [w320] -> w85
    tunnel: w86 -> [w318]
    tunnel: [w319] -> w84
    tunnel: [w331] -> w83
    tunnel: [w332] -> w82
    tunnel: w85 -> [w330]
    tunnel: w84 -> [w329]
    tunnel: w83 -> [w342]
    tunnel: w82 -> [w341]
    tunnel: [w344] -> w58
    tunnel: [w343] -> w57
    tunnel: [w338] -> w56
    tunnel: [w349] -> w71
    tunnel: [w350] -> w72
    tunnel: w58 -> [w350]
    tunnel: w57 -> [w349]
    tunnel: w56 -> [w345]
    frame #0 {
      n110 = call "mDrive Send Command.vi"("error in (no error)"=w293, "Extra"="EM=2", "Command"=T2."Send String", "VISA resource name"=w295) -> ("error out"=w292:errorcluster, "VISA resource name out"=w294:refnum<visa-resource-name>)  [unwired: 3 in, 1 out]
    }
    frame #1 {
      n111 = Number To Decimal String(number=1000000) -> (decimal integer string=w303:string)  [unwired: 1 in]
      n112 = call "mDrive Send Command.vi"("error in (no error)"=w300, "Extra"=w303, "Command"=T2."Accel Rate", "VISA resource name"=w299) -> ("error out"=w301:errorcluster, "VISA resource name out"=w307:refnum<visa-resource-name>)  [unwired: 3 in, 1 out]
      n113 = call "mDrive Send Command.vi"("error in (no error)"=w301, "Extra"=w303, "Command"=T2."Decel Rate", "VISA resource name"=w307) -> ("error out"=w302:errorcluster, "VISA resource name out"=w298:refnum<visa-resource-name>)  [unwired: 3 in, 1 out]
    }
    frame #2 {
      # "Run Current %"
      n114 = property on="X Run Current %" class="DigNum (strict)"() -> ("Value"=w309:i32)  [unwired: 2 in, 2 out]
      n115 = Number To Decimal String(number=w309) -> (decimal integer string=w310:string)  [unwired: 1 in]
      n116 = call "mDrive Send Command.vi"("error in (no error)"=w314, "Extra"=w310, "Command"=T2."Run Current", "VISA resource name"=w312) -> ("error out"=w313:errorcluster, "VISA resource name out"=w311:refnum<visa-resource-name>)  [unwired: 3 in, 1 out]
    }
    frame #3 {
      # "Holding Current %"
      n117 = property on="X Holding Current %" class="DigNum (strict)"() -> ("Value"=w316:i32)  [unwired: 2 in, 2 out]
      n118 = Number To Decimal String(number=w316) -> (decimal integer string=w317:string)  [unwired: 1 in]
      n119 = call "mDrive Send Command.vi"("error in (no error)"=w318, "Extra"=w317, "Command"=T2."Holding Current", "VISA resource name"=w321) -> ("error out"=w319:errorcluster, "VISA resource name out"=w320:refnum<visa-resource-name>)  [unwired: 3 in, 1 out]
    }
    frame #4 {
      # "Print Velocity Ma"
      # "Velocity Max"
      n120 = property on="X Velocity SP step/sec" class="DigNum (strict)"() -> ("Value"=w328:i32)  [unwired: 2 in, 2 out]
      n121 = Number To Decimal String(number=w328) -> (decimal integer string=w327:string)  [unwired: 1 in]
      n122 = call "mDrive Send Command.vi"("error in (no error)"=w329, "Extra"=w327, "Command"=T2."Max Velocity", "VISA resource name"=w330) -> ("error out"=w325:errorcluster, "VISA resource name out"=w335:refnum<visa-resource-name>)  [unwired: 3 in, 1 out]
      n123 = call "mDrive Send Command.vi"("error in (no error)"=w325, "Extra"="VM", "Command"=T2."Print Parameter", "VISA resource name"=w335) -> ("error out"=w332:errorcluster, "read buffer"=w333:string, "VISA resource name out"=w331:refnum<visa-resource-name>)  [unwired: 3 in]
      n124 = Decimal String To Number(string=w333, offset=0) -> (number=w326:i32)  [unwired: 1 in, 1 out]
      n125 = property on="X velocity PV step/sec" class="DigNum (strict)"("Val(Sgnl)"=w326) -> ()  [unwired: 2 in, 2 out]
    }
    frame #5 {
      # "PRINT POSITION"
      n126 = call "mDrive Send Command.vi"("error in (no error)"=w341, "Extra"="P", "Command"=T2."Print Parameter", "VISA resource name"=w342) -> ("error out"=w343:errorcluster, "read buffer"=w340:string, "VISA resource name out"=w344:refnum<visa-resource-name>)  [unwired: 3 in]
      n127 = Decimal String To Number(string=w340, offset=0) -> (number=w338:i32)  [unwired: 1 in, 1 out]
    }
    frame #6 {
      w347 = -2304000 ("lower limit")
      w348 = 2304000 ("upper limit")
      n128 = property on="X Step SP" class="DigNum (strict)"("Val(Sgnl)"=w345) -> ()  [unwired: 2 in, 2 out]
      n129 = property on="X Step SP" class="DigNum (strict)"("Maximum"=w348) -> ()  [unwired: 2 in, 2 out]
      n130 = In Range and Coerce(upper limit=w348, x=w345, lower limit=w347) -> (In Range?=w346:bool)  [unwired: 1 out]
      n131 = property on="X Step SP" class="DigNum (strict)"("Minimum"=w347) -> ()  [unwired: 2 in, 2 out]
      n132 = property on="X  in Range" class="Bool (strict)"("Val(Sgnl)"=w346) -> ()  [unwired: 2 in, 2 out]
      "X MINPOS" <- w347
      "X MAXPOS" <- w348
    }
  }
  n133 = flat-sequence {
    tunnel: w27 -> [w354]
    tunnel: w28 -> [w352]
    tunnel: [w351] -> w14
    tunnel: [w353] -> w12
    tunnel: w14 -> [w358]
    tunnel: [w359] -> w13
    tunnel: w12 -> [w357]
    tunnel: [w360] -> w11
    tunnel: [w371] -> w44
    tunnel: [w373] -> w43
    tunnel: w13 -> [w372]
    tunnel: w11 -> [w367]
    tunnel: w44 -> [w380]
    tunnel: [w379] -> w42
    tunnel: w43 -> [w377]
    tunnel: [w378] -> w41
    tunnel: [w390] -> w40
    tunnel: [w391] -> w39
    tunnel: w42 -> [w389]
    tunnel: w41 -> [w388]
    tunnel: w40 -> [w401]
    tunnel: w39 -> [w400]
    tunnel: [w403] -> w38
    tunnel: [w402] -> w37
    tunnel: [w397] -> w36
    tunnel: [w408] -> w21
    tunnel: [w409] -> w22
    tunnel: w38 -> [w409]
    tunnel: w37 -> [w408]
    tunnel: w36 -> [w406]
    frame #0 {
      n134 = call "mDrive Send Command.vi"("error in (no error)"=w354, "Extra"="EM=2", "Command"=T2."Send String", "VISA resource name"=w352) -> ("error out"=w353:errorcluster, "VISA resource name out"=w351:refnum<visa-resource-name>)  [unwired: 3 in, 1 out]
    }
    frame #1 {
      # "pr=1000000"
      n135 = Number To Decimal String(number=100000) -> (decimal integer string=w362:string)  [unwired: 1 in]
      n136 = call "mDrive Send Command.vi"("error in (no error)"=w357, "Extra"=w362, "Command"=T2."Accel Rate", "VISA resource name"=w358) -> ("error out"=w361:errorcluster, "VISA resource name out"=w366:refnum<visa-resource-name>)  [unwired: 3 in, 1 out]
      n137 = call "mDrive Send Command.vi"("error in (no error)"=w361, "Extra"=w362, "Command"=T2."Decel Rate", "VISA resource name"=w366) -> ("error out"=w360:errorcluster, "VISA resource name out"=w359:refnum<visa-resource-name>)  [unwired: 3 in, 1 out]
    }
    frame #2 {
      # "Run Current %"
      n138 = property on="R Run Current %" class="DigNum (strict)"() -> ("Value"=w369:i32)  [unwired: 2 in, 2 out]
      n139 = Number To Decimal String(number=w369) -> (decimal integer string=w370:string)  [unwired: 1 in]
      n140 = call "mDrive Send Command.vi"("error in (no error)"=w367, "Extra"=w370, "Command"=T2."Run Current", "VISA resource name"=w372) -> ("error out"=w373:errorcluster, "VISA resource name out"=w371:refnum<visa-resource-name>)  [unwired: 3 in, 1 out]
    }
    frame #3 {
      # "Holding Current %"
      n141 = property on="R Holding Current %" class="DigNum (strict)"() -> ("Value"=w375:i32)  [unwired: 2 in, 2 out]
      n142 = Number To Decimal String(number=w375) -> (decimal integer string=w376:string)  [unwired: 1 in]
      n143 = call "mDrive Send Command.vi"("error in (no error)"=w377, "Extra"=w376, "Command"=T2."Holding Current", "VISA resource name"=w380) -> ("error out"=w378:errorcluster, "VISA resource name out"=w379:refnum<visa-resource-name>)  [unwired: 3 in, 1 out]
    }
    frame #4 {
      # "Print Velocity Ma"
      # "Velocity Max"
      n144 = property on="R Velocity SP step/sec" class="DigNum (strict)"() -> ("Value"=w387:i32)  [unwired: 2 in, 2 out]
      n145 = Number To Decimal String(number=w387) -> (decimal integer string=w386:string)  [unwired: 1 in]
      n146 = call "mDrive Send Command.vi"("error in (no error)"=w388, "Extra"=w386, "Command"=T2."Max Velocity", "VISA resource name"=w389) -> ("error out"=w384:errorcluster, "VISA resource name out"=w394:refnum<visa-resource-name>)  [unwired: 3 in, 1 out]
      n147 = call "mDrive Send Command.vi"("error in (no error)"=w384, "Extra"="VM", "Command"=T2."Print Parameter", "VISA resource name"=w394) -> ("error out"=w391:errorcluster, "read buffer"=w392:string, "VISA resource name out"=w390:refnum<visa-resource-name>)  [unwired: 3 in]
      n148 = Decimal String To Number(string=w392, offset=0) -> (number=w385:i32)  [unwired: 1 in, 1 out]
      n149 = property on="R velocity PV step/sec" class="DigNum (strict)"("Val(Sgnl)"=w385) -> ()  [unwired: 2 in, 2 out]
    }
    frame #5 {
      # "PRINT POSITION"
      n150 = call "mDrive Send Command.vi"("error in (no error)"=w400, "Extra"="P", "Command"=T2."Print Parameter", "VISA resource name"=w401) -> ("error out"=w402:errorcluster, "read buffer"=w399:string, "VISA resource name out"=w403:refnum<visa-resource-name>)  [unwired: 3 in]
      n151 = Decimal String To Number(string=w399, offset=0) -> (number=w397:i32)  [unwired: 1 in, 1 out]
    }
    frame #6 {
      w405 = -6144000 ("lower limit")
      w404 = 0 ("upper limit")
      n152 = property on="R Step SP" class="DigNum (strict)"("Val(Sgnl)"=w406) -> ()  [unwired: 2 in, 2 out]
      n153 = property on="R Step SP" class="DigNum (strict)"("Maximum"=w404) -> ()  [unwired: 2 in, 2 out]
      n154 = In Range and Coerce(upper limit=w404, x=w406, lower limit=w405) -> (In Range?=w407:bool)  [unwired: 1 out]
      n155 = property on="R Step SP" class="DigNum (strict)"("Minimum"=w405) -> ()  [unwired: 2 in, 2 out]
      n156 = property on="R in Range" class="Bool (strict)"("Val(Sgnl)"=w407) -> ()  [unwired: 2 in, 2 out]
      "R MINPOS" <- w405
      "R MAXPOS" <- w404
    }
  }
  n157 = property on="Z Step SP" class="DigNum (strict)"("Minimum"=0 ("lower limit")) -> ()  [unwired: 2 in, 2 out]
  n158 = property on="Z Step SP" class="DigNum (strict)"("Maximum"=102400000 ("upper limit")) -> ()  [unwired: 2 in, 2 out]
  n159 = while {
    tunnel: w99 -> [w425]
    tunnel: w98 -> [w428]
    tunnel: [w429] -> w96
    tunnel: [w427] -> w97
    tunnel: w72 -> [w423]
    tunnel: w71 -> [w422]
    tunnel: [w421] -> w70
    tunnel: [w420] -> w69
    tunnel: w26 -> [w419]
    tunnel: w25 -> [w418]
    tunnel: [w417] -> w24
    tunnel: [w416] -> w23
    tunnel: w22 -> [w415]
    tunnel: w21 -> [w414]
    tunnel: [w413] -> w20
    tunnel: [w412] -> w19
    stop <- w424 stop-if-true
    n160 = property on="X COM PORT" class="VISAName"() -> ("Value"=w411:refnum<visa-resource-name>)  [unwired: 2 in, 2 out]
    n161 = property on="Y COM PORT" class="VISAName"() -> ("Value"=w410:refnum<visa-resource-name>)  [unwired: 2 in, 2 out]
    n162 = event shown="[0] Timeout" {
      selector: _ -> [_ _ _ _ _ _ _ _ _ _ _ _ _ _ _ _ _ _ _ _ _ _ _ _ _]
      dyn-events: _ -> [_ _ _ _ _ _ _ _ _ _ _ _ _ _ _ _ _ _ _ _ _ _ _ _ _]
      timeout: 200 -> [_ _ _ _ _ _ _ _ _ _ _ _ _ _ _ _ _ _ _ _ _ _ _ _ _]
      tunnel: w428 -> [w495 _ _ _ _ _ _ _ _ _ _ _ w1324 _ _ _ _ w1573 _ _ w1669 w1685 w1729 w1806 w2050]
      tunnel: [w494 _ _ _ _ _ _ _ _ _ _ _ w1330 _ _ _ _ w1571 _ _ w1669 w1683 w1731 w1795 w2048] -> w429
      tunnel: w425 -> [_ _ _ _ _ _ _ _ _ _ _ _ w1325 _ _ _ _ w1572 _ _ w1670 w1686 w1730 w1808 w2051]
      tunnel: [w493 _ _ _ _ _ _ _ _ _ _ _ w1331 _ _ _ _ w1568 _ _ w1670 w1684 w1732 w1796 w2049] -> w427
      tunnel: [_ _ _ _ _ _ _ _ _ _ _ _ _ _ _ _ _ _ _ _ TRUE _ _ _ _] -> w424
      tunnel: w423 -> [_ _ _ _ _ _ _ _ _ _ _ _ _ _ _ w1482 w1537 _ _ _ _ w1680 w1722 w1812 w2047]
      tunnel: w422 -> [w470 _ _ _ _ _ _ _ _ _ _ _ _ _ _ w1481 w1536 _ _ _ _ w1679 w1721 w1810 w2046]
      tunnel: [w469 _ _ _ _ _ _ _ _ _ _ _ _ _ _ w1480 w1535 _ _ _ _ w1682 w1720 w1788 w2045] -> w421
      tunnel: [w468 _ _ _ _ _ _ _ _ _ _ _ _ _ _ w1479 w1534 _ _ _ _ w1681 w1719 w1786 w2044] -> w420
      tunnel: w419 -> [w442 _ _ _ _ _ _ _ _ _ _ _ _ w1376 _ _ _ _ w1603 _ _ w1678 w1716 w1804 w2043]
      tunnel: w418 -> [w445 _ _ _ _ _ _ _ _ _ _ _ _ w1375 _ _ _ _ w1602 _ _ w1677 w1715 w1802 w2042]
      tunnel: [w444 _ _ _ _ _ _ _ _ _ _ _ _ w1373 _ _ _ _ w1600 _ _ w1676 w1714 w1794 w2039] -> w417
      tunnel: [w443 _ _ _ _ _ _ _ _ _ _ _ _ w1374 _ _ _ _ w1601 _ _ w1675 w1713 w1793 w2038] -> w416
      tunnel: w415 -> [w441 _ _ _ _ _ _ _ _ _ _ _ _ _ w1429 _ _ _ _ w1637 _ w1674 w1710 w1799 w2041]
      tunnel: w414 -> [w440 _ _ _ _ _ _ _ _ _ _ _ _ _ w1428 _ _ _ _ w1636 _ w1673 w1709 w1797 w2040]
      tunnel: [w439 _ _ _ _ _ _ _ _ _ _ _ _ _ w1426 _ _ _ _ w1635 _ w1672 w1708 w1791 w2037] -> w413
      tunnel: [w438 _ _ _ _ _ _ _ _ _ _ _ _ _ w1427 _ _ _ _ w1634 _ w1671 w1707 w1790 w2036] -> w412
      tunnel: w411 -> [w431 _ _ _ _ _ _ _ _ _ _ _ _ _ _ _ _ _ _ _ _ _ _ _ _]
      tunnel: w410 -> [w430 _ _ _ _ _ _ _ _ _ _ _ _ _ _ _ _ _ _ _ _ _ _ _ _]
      event #0 {
        n163 = event-data() -> ()  [unwired: 1 in, 2 out]
        n164 = flat-sequence {
          tunnel: [w785] -> w481
          tunnel: [w761] -> w480
          tunnel: [w774] -> w479
          tunnel: [w752] -> w478
          tunnel: w431 -> [w751]
          tunnel: w470 -> [w750]
          tunnel: w481 -> [w791]
          tunnel: [w791] -> w477
          tunnel: w480 -> [w790]
          tunnel: [w790] -> w476
          tunnel: w479 -> [w789]
          tunnel: [w789] -> w475
          tunnel: w478 -> [w786]
          tunnel: [w786] -> w474
          tunnel: w477 -> [w798]
          tunnel: [w799] -> w473
          tunnel: w476 -> [w801]
          tunnel: [w800] -> w472
          tunnel: w475 -> [w797]
          tunnel: [w796] -> w471
          tunnel: w474 -> [w796]
          tunnel: w473 -> [w811]
          tunnel: w472 -> [w812]
          tunnel: w471 -> [w814]
          tunnel: [w810] -> w468
          tunnel: [w809] -> w469
          frame #0 {
            w756 = 0.05 ("Delay Time (s)")
            n165 = property on="X Step SP" class="DigNum (strict)"() -> ("Maximum"=w776:dbl)  [unwired: 2 in, 2 out]
            n166 = property on="X Step SP" class="DigNum (strict)"() -> ("Minimum"=w778:dbl)  [unwired: 2 in, 2 out]
            n167 = property on="X steps/rev" class="DigNum (strict)"() -> ("Value"=w772:u32)  [unwired: 2 in, 2 out]
            n168 = property on="X offset mm" class="DigNum (strict)"() -> ("Value"=w768:dbl)  [unwired: 2 in, 2 out]
            n169 = To Long Integer(number=w776) -> (32bit integer=w775:i32)
            n170 = To Long Integer(number=w778) -> (32bit integer=w777:i32)
            n171 = To Double Precision Float(number=w772) -> (double precision float=w773:dbl)
            n172 = call "mDrive Send Command.vi"("error in (no error)"=w750, "Extra"="P", "Command"=T2."Print Parameter", "VISA resource name"=w751) -> ("error out"=w780:errorcluster, "read buffer"=w784:string, "VISA resource name out"=w782:refnum<visa-resource-name>)  [unwired: 3 in]
            n173 = call "Time Delay12"("error in (no error)"=w780, "Delay Time (s)"=w756) -> ("error out"=w779:errorcluster)  [unwired: 9 in]
            n174 = Decimal String To Number(string=w784, offset=0) -> (number=w764:i32)  [unwired: 1 in, 1 out]
            n175 = To Long Integer(number=w764) -> (32bit integer=w766:i32)
            n176 = property on="X Step PV" class="DigNum (strict)"("Val(Sgnl)"=w766) -> ()  [unwired: 2 in, 2 out]
            n177 = call "mDrive Send Command.vi"("error in (no error)"=w779, "Extra"="MV", "Command"=T2."Print Parameter", "VISA resource name"=w782) -> ("error out"=w781:errorcluster, "read buffer"=w762:string, "VISA resource name out"=w785:refnum<visa-resource-name>)  [unwired: 3 in]
            n178 = call "Time Delay11"("error in (no error)"=w781, "Delay Time (s)"=w756) -> ("error out"=w761:errorcluster)  [unwired: 9 in]
            n179 = In Range and Coerce(upper limit=w775, x=w766, lower limit=w777) -> (In Range?=w774:bool)  [unwired: 1 out]
            n180 = To Double Precision Float(number=w766) -> (double precision float=w767:dbl)
            n181 = Decimal String To Number(string=w762, offset=0 ("offset (0)")) -> (number=w755:i32)  [unwired: 1 in, 1 out]
            n182 = Divide(x=w767, y=w773) -> (x/y=w771:dbl)
            n183 = Number To Boolean Array(number=w755) -> (Boolean array=w754:bool[])
            n184 = property on="X  in Range" class="Bool (strict)"("Val(Sgnl)"=w774) -> ()  [unwired: 2 in, 2 out]
            n185 = property on="X mm/rev" class="DigNum (strict)"() -> ("Value"=w770:dbl)  [unwired: 2 in, 2 out]
            n186 = Index Array(array=w754, index=0) -> (element=w752:bool)
            n187 = Multiply(x=w771, y=w770) -> (x*y=w769:dbl)
            n188 = property on="X  in Motion" class="Bool (strict)"("Val(Sgnl)"=w752) -> ()  [unwired: 2 in, 2 out]
            n189 = Add(x=w769, y=w768) -> (x+y=w765:dbl)
            n190 = property on="X Position mm PV" class="DigNum (strict)"("Val(Sgnl)"=w765) -> ()  [unwired: 2 in, 2 out]
          }
          frame #1 {
            n191 = property on="X Scan" class="Bool (strict)"() -> ("Value"=w787:bool)  [unwired: 2 in, 2 out]
            n192 = Or(x=w786, y=w787) -> (x .or. y?=w788:bool)
            n193 = case shown="True" w788 {
              frame #0 {
                n194 = property on="X Go" class="Bool"("DisabledEnum"=T1."Enabled" ("Disabled")) -> ()  [unwired: 2 in, 2 out]
                n195 = property on="X Scan OK" class="Bool"("DisabledEnum"=T1."Enabled" ("Disabled")) -> ()  [unwired: 2 in, 2 out]
              }
              frame #1 {
                n196 = property on="X Go" class="Bool"("DisabledEnum"=T1."Disabled and Grayed Out" ("Disabled")) -> ()  [unwired: 2 in, 2 out]
                n197 = property on="X Scan OK" class="Bool"("DisabledEnum"=T1."Disabled and Grayed Out" ("Disabled")) -> ()  [unwired: 2 in, 2 out]
              }
            }
          }
          frame #2 {
            n198 = case shown="False" w797 {
              tunnel: w798 -> [w804 w808]
              tunnel: [w805 w808] -> w799
              tunnel: [w806 w807] -> w800
              tunnel: w801 -> [w803 w807]
              frame #0 {
                n199 = call "mDrive Send Command.vi"("error in (no error)"=w803, "Command"=T2."Stop", "VISA resource name"=w804) -> ("error out"=w806:errorcluster, "VISA resource name out"=w805:refnum<visa-resource-name>)  [unwired: 4 in, 1 out]
              }
              frame #1 {
              }
            }
          }
          frame #3 {
            n200 = property on="X Backlash corr" class="Bool (strict)"() -> ("Value"=w815:bool)  [unwired: 2 in, 2 out]
            n201 = Implies(1:w814, 2:w815) -> (0:w813:bool)
            n202 = case shown="False" w813 {
              tunnel: w812 -> [w822 w875]
              tunnel: w811 -> [w821 w876]
              tunnel: [w820 w875] -> w810
              tunnel: [w819 w876] -> w809
              frame #0 {
                # "Backlash"
                n203 = flat-sequence {
                  tunnel: [w837] -> w834
                  tunnel: [w839] -> w833
                  tunnel: [w838] -> w832
                  tunnel: w822 -> [w836]
                  tunnel: w821 -> [w835]
                  tunnel: w834 -> [w847]
                  tunnel: [w847] -> w831
                  tunnel: w833 -> [w846]
                  tunnel: w832 -> [w845]
                  tunnel: [w844] -> w830
                  tunnel: [w843] -> w829
                  tunnel: [w842] -> w818
                  tunnel: w831 -> [w857]
                  tunnel: w830 -> [w856]
                  tunnel: w829 -> [w854]
                  tunnel: [w855] -> w828
                  tunnel: [w854] -> w827
                  tunnel: [w853] -> w824
                  tunnel: [w852] -> w823
                  tunnel: w818 -> [w852]
                  tunnel: w828 -> [w868]
                  tunnel: w827 -> [w861]
                  tunnel: [w868] -> w826
                  tunnel: [w867] -> w825
                  tunnel: w824 -> [w867]
                  tunnel: w823 -> [w863]
                  tunnel: [w862] -> w816
                  tunnel: w826 -> [w872]
                  tunnel: w825 -> [w871]
                  tunnel: [w870] -> w820
                  tunnel: [w869] -> w817
                  tunnel: w816 -> [w869]
                  tunnel: [w874] -> w819
                  tunnel: w817 -> [w874]
                  frame #0 {
                    n204 = property on="X Backlash steps/sec" class="DigNum (strict)"() -> ("Value"=w837:i32)  [unwired: 2 in, 2 out]
                    n205 = Number To Decimal String(number=w837) -> (decimal integer string=w840:string)  [unwired: 1 in]
                    n206 = call "mDrive Send Command.vi"("error in (no error)"=w836, "Extra"=w840, "Command"=T2."Max Velocity", "VISA resource name"=w835) -> ("error out"=w838:errorcluster, "VISA resource name out"=w839:refnum<visa-resource-name>)  [unwired: 3 in, 1 out]
                  }
                  frame #1 {
                    n207 = property on="X Backlash" class="DigNum (strict)"() -> ("Value"=w842:i32)  [unwired: 2 in, 2 out]
                    n208 = Number To Decimal String(number=w842) -> (decimal integer string=w848:string)  [unwired: 1 in]
                    n209 = call "mDrive Send Command.vi"("error in (no error)"=w845, "Extra"=w848, "Command"=T2."Move to Relative Position", "VISA resource name"=w846) -> ("error out"=w844:errorcluster, "VISA resource name out"=w843:refnum<visa-resource-name>)  [unwired: 3 in, 1 out]
                  }
                  frame #2 {
                    n210 = To Double Precision Float(number=w852) -> (double precision float=w850:dbl)
                    n211 = To Double Precision Float(number=w857) -> (double precision float=w859:dbl)
                    n212 = Absolute Value(x=w850) -> (abs(x)=w851:dbl)
                    n213 = Divide(x=w851, y=w859) -> (x/y=w860:dbl)
                    n214 = Add(x=w860, y=0.3) -> (x+y=w853:dbl)
                    n215 = call "Time Delay13"("error in (no error)"=w856, "Delay Time (s)"=w853) -> ("error out"=w855:errorcluster)  [unwired: 9 in]
                  }
                  frame #3 {
                    n216 = Negate(x=w863) -> (-x=w864:i32)
                    n217 = Number To Decimal String(number=w864) -> (decimal integer string=w865:string)  [unwired: 1 in]
                    n218 = call "mDrive Send Command.vi"("Extra"=w865, "Command"=T2."Move to Relative Position", "VISA resource name"=w861) -> ("VISA resource name out"=w862:refnum<visa-resource-name>)  [unwired: 4 in, 2 out]
                  }
                  frame #4 {
                    n219 = call "Time Delay14"("error in (no error)"=w872, "Delay Time (s)"=w871) -> ("error out"=w870:errorcluster)  [unwired: 9 in]
                  }
                  frame #5 {
                    n220 = property on="X Backlash corr" class="Bool (strict)"("Val(Sgnl)"=FALSE ("Value (Signaling)")) -> ()  [unwired: 2 in, 2 out]
                  }
                }
              }
              frame #1 {
              }
            }
          }
        }
        n221 = flat-sequence {
          tunnel: w495 -> [w907]
          tunnel: w430 -> [w906]
          tunnel: [w912] -> w492
          tunnel: [w886] -> w490
          tunnel: [w899] -> w488
          tunnel: [w877] -> w486
          tunnel: w492 -> [w918]
          tunnel: [w918] -> w491
          tunnel: w490 -> [w917]
          tunnel: [w917] -> w489
          tunnel: w488 -> [w916]
          tunnel: [w916] -> w487
          tunnel: w486 -> [w913]
          tunnel: [w913] -> w482
          tunnel: w491 -> [w925]
          tunnel: [w926] -> w485
          tunnel: w489 -> [w928]
          tunnel: [w927] -> w484
          tunnel: w487 -> [w924]
          tunnel: [w923] -> w483
          tunnel: w482 -> [w923]
          tunnel: w485 -> [w938]
          tunnel: w484 -> [w939]
          tunnel: w483 -> [w941]
          tunnel: [w937] -> w494
          tunnel: [w936] -> w493
          frame #0 {
            w881 = 0.05 ("Delay Time (s)")
            n222 = property on="Y Step SP" class="DigNum (strict)"() -> ("Maximum"=w901:dbl)  [unwired: 2 in, 2 out]
            n223 = property on="Y Step SP" class="DigNum (strict)"() -> ("Minimum"=w903:dbl)  [unwired: 2 in, 2 out]
            n224 = property on="Y steps/rev" class="DigNum (strict)"() -> ("Value"=w897:u32)  [unwired: 2 in, 2 out]
            n225 = property on="Y offset mm" class="DigNum (strict)"() -> ("Value"=w893:dbl)  [unwired: 2 in, 2 out]
            n226 = To Long Integer(number=w901) -> (32bit integer=w900:i32)
            n227 = To Long Integer(number=w903) -> (32bit integer=w902:i32)
            n228 = To Double Precision Float(number=w897) -> (double precision float=w898:dbl)
            n229 = call "mDrive Send Command.vi"("error in (no error)"=w907, "Extra"="P", "Command"=T2."Print Parameter", "VISA resource name"=w906) -> ("error out"=w905:errorcluster, "read buffer"=w911:string, "VISA resource name out"=w909:refnum<visa-resource-name>)  [unwired: 3 in]
            n230 = call "Time Delay4"("error in (no error)"=w905, "Delay Time (s)"=w881) -> ("error out"=w904:errorcluster)  [unwired: 9 in]
            n231 = Decimal String To Number(string=w911, offset=0) -> (number=w889:i32)  [unwired: 1 in, 1 out]
            n232 = To Long Integer(number=w889) -> (32bit integer=w891:i32)
            n233 = property on="Y Step PV" class="DigNum (strict)"("Val(Sgnl)"=w891) -> ()  [unwired: 2 in, 2 out]
            n234 = call "mDrive Send Command.vi"("error in (no error)"=w904, "Extra"="MV", "Command"=T2."Print Parameter", "VISA resource name"=w909) -> ("error out"=w908:errorcluster, "read buffer"=w887:string, "VISA resource name out"=w912:refnum<visa-resource-name>)  [unwired: 3 in]
            n235 = call "Time Delay3"("error in (no error)"=w908, "Delay Time (s)"=w881) -> ("error out"=w886:errorcluster)  [unwired: 9 in]
            n236 = In Range and Coerce(upper limit=w900, x=w891, lower limit=w902) -> (In Range?=w899:bool)  [unwired: 1 out]
            n237 = To Double Precision Float(number=w891) -> (double precision float=w892:dbl)
            n238 = Decimal String To Number(string=w887, offset=0 ("offset (0)")) -> (number=w880:i32)  [unwired: 1 in, 1 out]
            n239 = property on="Y in Range" class="Bool (strict)"("Val(Sgnl)"=w899) -> ()  [unwired: 2 in, 2 out]
            n240 = Divide(x=w892, y=w898) -> (x/y=w896:dbl)
            n241 = Number To Boolean Array(number=w880) -> (Boolean array=w879:bool[])
            n242 = property on="Y mm/rev" class="DigNum (strict)"() -> ("Value"=w895:dbl)  [unwired: 2 in, 2 out]
            n243 = Index Array(array=w879, index=0) -> (element=w877:bool)
            n244 = Multiply(x=w896, y=w895) -> (x*y=w894:dbl)
            n245 = property on="Y in Motion" class="Bool (strict)"("Val(Sgnl)"=w877) -> ()  [unwired: 2 in, 2 out]
            n246 = Add(x=w894, y=w893) -> (x+y=w890:dbl)
            n247 = property on="Y Position mm PV" class="DigNum (strict)"("Val(Sgnl)"=w890) -> ()  [unwired: 2 in, 2 out]
          }
          frame #1 {
            n248 = property on="Y Scan" class="Bool (strict)"() -> ("Value"=w914:bool)  [unwired: 2 in, 2 out]
            n249 = Or(x=w913, y=w914) -> (x .or. y?=w915:bool)
            n250 = case shown="True" w915 {
              frame #0 {
                n251 = property on="Y Go" class="Bool"("DisabledEnum"=T1."Enabled" ("Disabled")) -> ()  [unwired: 2 in, 2 out]
                n252 = property on="Y Scan OK" class="Bool"("DisabledEnum"=T1."Enabled" ("Disabled")) -> ()  [unwired: 2 in, 2 out]
              }
              frame #1 {
                n253 = property on="Y Go" class="Bool"("DisabledEnum"=T1."Disabled and Grayed Out" ("Disabled")) -> ()  [unwired: 2 in, 2 out]
                n254 = property on="Y Scan OK" class="Bool"("DisabledEnum"=T1."Disabled and Grayed Out" ("Disabled")) -> ()  [unwired: 2 in, 2 out]
              }
            }
          }
          frame #2 {
            n255 = case shown="False" w924 {
              tunnel: w925 -> [w931 w935]
              tunnel: [w932 w935] -> w926
              tunnel: [w933 w934] -> w927
              tunnel: w928 -> [w930 w934]
              frame #0 {
                n256 = call "mDrive Send Command.vi"("error in (no error)"=w930, "Command"=T2."Stop", "VISA resource name"=w931) -> ("error out"=w933:errorcluster, "VISA resource name out"=w932:refnum<visa-resource-name>)  [unwired: 4 in, 1 out]
              }
              frame #1 {
              }
            }
          }
          frame #3 {
            n257 = property on="Y Backlash corr" class="Bool (strict)"() -> ("Value"=w942:bool)  [unwired: 2 in, 2 out]
            n258 = Implies(1:w941, 2:w942) -> (0:w940:bool)
            n259 = case shown="False" w940 {
              tunnel: w939 -> [w949 w1002]
              tunnel: w938 -> [w948 w1003]
              tunnel: [w947 w1002] -> w937
              tunnel: [w946 w1003] -> w936
              frame #0 {
                # "Backlash"
                n260 = flat-sequence {
                  tunnel: [w964] -> w961
                  tunnel: [w966] -> w960
                  tunnel: [w965] -> w959
                  tunnel: w949 -> [w963]
                  tunnel: w948 -> [w962]
                  tunnel: w961 -> [w974]
                  tunnel: [w974] -> w958
                  tunnel: w960 -> [w973]
                  tunnel: w959 -> [w972]
                  tunnel: [w971] -> w957
                  tunnel: [w970] -> w956
                  tunnel: [w969] -> w945
                  tunnel: w958 -> [w984]
                  tunnel: w957 -> [w983]
                  tunnel: w956 -> [w981]
                  tunnel: [w982] -> w955
                  tunnel: [w981] -> w954
                  tunnel: [w980] -> w951
                  tunnel: [w979] -> w950
                  tunnel: w945 -> [w979]
                  tunnel: w955 -> [w995]
                  tunnel: w954 -> [w988]
                  tunnel: [w995] -> w953
                  tunnel: [w994] -> w952
                  tunnel: w951 -> [w994]
                  tunnel: w950 -> [w990]
                  tunnel: [w989] -> w943
                  tunnel: w953 -> [w999]
                  tunnel: w952 -> [w998]
                  tunnel: [w997] -> w947
                  tunnel: [w996] -> w944
                  tunnel: w943 -> [w996]
                  tunnel: [w1001] -> w946
                  tunnel: w944 -> [w1001]
                  frame #0 {
                    n261 = property on="Y Backlash steps/sec" class="DigNum (strict)"() -> ("Value"=w964:i32)  [unwired: 2 in, 2 out]
                    n262 = Number To Decimal String(number=w964) -> (decimal integer string=w967:string)  [unwired: 1 in]
                    n263 = call "mDrive Send Command.vi"("error in (no error)"=w963, "Extra"=w967, "Command"=T2."Max Velocity", "VISA resource name"=w962) -> ("error out"=w965:errorcluster, "VISA resource name out"=w966:refnum<visa-resource-name>)  [unwired: 3 in, 1 out]
                  }
                  frame #1 {
                    n264 = property on="Y Backlash" class="DigNum (strict)"() -> ("Value"=w969:i32)  [unwired: 2 in, 2 out]
                    n265 = Number To Decimal String(number=w969) -> (decimal integer string=w975:string)  [unwired: 1 in]
                    n266 = call "mDrive Send Command.vi"("error in (no error)"=w972, "Extra"=w975, "Command"=T2."Move to Relative Position", "VISA resource name"=w973) -> ("error out"=w971:errorcluster, "VISA resource name out"=w970:refnum<visa-resource-name>)  [unwired: 3 in, 1 out]
                  }
                  frame #2 {
                    n267 = To Double Precision Float(number=w979) -> (double precision float=w977:dbl)
                    n268 = To Double Precision Float(number=w984) -> (double precision float=w986:dbl)
                    n269 = Absolute Value(x=w977) -> (abs(x)=w978:dbl)
                    n270 = Divide(x=w978, y=w986) -> (x/y=w987:dbl)
                    n271 = Add(x=w987, y=0.3) -> (x+y=w980:dbl)
                    n272 = call "Time Delay8"("error in (no error)"=w983, "Delay Time (s)"=w980) -> ("error out"=w982:errorcluster)  [unwired: 9 in]
                  }
                  frame #3 {
                    n273 = Negate(x=w990) -> (-x=w991:i32)
                    n274 = Number To Decimal String(number=w991) -> (decimal integer string=w992:string)  [unwired: 1 in]
                    n275 = call "mDrive Send Command.vi"("Extra"=w992, "Command"=T2."Move to Relative Position", "VISA resource name"=w988) -> ("VISA resource name out"=w989:refnum<visa-resource-name>)  [unwired: 4 in, 2 out]
                  }
                  frame #4 {
                    n276 = call "Time Delay2"("error in (no error)"=w999, "Delay Time (s)"=w998) -> ("error out"=w997:errorcluster)  [unwired: 9 in]
                  }
                  frame #5 {
                    n277 = property on="Y Backlash corr" class="Bool (strict)"("Val(Sgnl)"=FALSE ("Value (Signaling)")) -> ()  [unwired: 2 in, 2 out]
                  }
                }
              }
              frame #1 {
              }
            }
          }
        }
        n278 = flat-sequence {
          tunnel: [w658] -> w467
          tunnel: [w634] -> w466
          tunnel: [w647] -> w465
          tunnel: [w625] -> w464
          tunnel: w442 -> [w624]
          tunnel: w445 -> [w623]
          tunnel: w467 -> [w664]
          tunnel: [w664] -> w463
          tunnel: w466 -> [w663]
          tunnel: [w663] -> w462
          tunnel: w465 -> [w662]
          tunnel: [w662] -> w461
          tunnel: w464 -> [w659]
          tunnel: [w659] -> w460
          tunnel: w463 -> [w671]
          tunnel: [w672] -> w459
          tunnel: w462 -> [w674]
          tunnel: [w673] -> w458
          tunnel: w461 -> [w670]
          tunnel: [w669] -> w457
          tunnel: w460 -> [w669]
          tunnel: w459 -> [w684]
          tunnel: w458 -> [w685]
          tunnel: w457 -> [w687]
          tunnel: [w683] -> w443
          tunnel: [w682] -> w444
          frame #0 {
            w629 = 0.05 ("Delay Time (s)")
            n279 = property on="Z Step SP" class="DigNum (strict)"() -> ("Maximum"=w649:dbl)  [unwired: 2 in, 2 out]
            n280 = property on="Z Step SP" class="DigNum (strict)"() -> ("Minimum"=w651:dbl)  [unwired: 2 in, 2 out]
            n281 = property on="Z steps/rev" class="DigNum (strict)"() -> ("Value"=w645:u32)  [unwired: 2 in, 2 out]
            n282 = property on="Z offset mm" class="DigNum (strict)"() -> ("Value"=w641:dbl)  [unwired: 2 in, 2 out]
            n283 = To Long Integer(number=w649) -> (32bit integer=w648:i32)
            n284 = To Long Integer(number=w651) -> (32bit integer=w650:i32)
            n285 = To Double Precision Float(number=w645) -> (double precision float=w646:dbl)
            n286 = call "mDrive Send Command.vi"("error in (no error)"=w623, "Extra"="P", "Command"=T2."Print Parameter", "VISA resource name"=w624) -> ("error out"=w653:errorcluster, "read buffer"=w657:string, "VISA resource name out"=w655:refnum<visa-resource-name>)  [unwired: 3 in]
            n287 = call "Time Delay17"("error in (no error)"=w653, "Delay Time (s)"=w629) -> ("error out"=w652:errorcluster)  [unwired: 9 in]
            n288 = Decimal String To Number(string=w657, offset=0) -> (number=w637:i32)  [unwired: 1 in, 1 out]
            n289 = To Long Integer(number=w637) -> (32bit integer=w639:i32)
            n290 = property on="Z Step PV" class="DigNum (strict)"("Val(Sgnl)"=w639) -> ()  [unwired: 2 in, 2 out]
            n291 = call "mDrive Send Command.vi"("error in (no error)"=w652, "Extra"="MV", "Command"=T2."Print Parameter", "VISA resource name"=w655) -> ("error out"=w654:errorcluster, "read buffer"=w635:string, "VISA resource name out"=w658:refnum<visa-resource-name>)  [unwired: 3 in]
            n292 = call "Time Delay16"("error in (no error)"=w654, "Delay Time (s)"=w629) -> ("error out"=w634:errorcluster)  [unwired: 9 in]
            n293 = In Range and Coerce(upper limit=w648, x=w639, lower limit=w650) -> (In Range?=w647:bool)  [unwired: 1 out]
            n294 = To Double Precision Float(number=w639) -> (double precision float=w640:dbl)
            n295 = Decimal String To Number(string=w635, offset=0 ("offset (0)")) -> (number=w628:i32)  [unwired: 1 in, 1 out]
            n296 = property on="Z in Range" class="Bool (strict)"("Val(Sgnl)"=w647) -> ()  [unwired: 2 in, 2 out]
            n297 = Divide(x=w640, y=w646) -> (x/y=w644:dbl)
            n298 = Number To Boolean Array(number=w628) -> (Boolean array=w627:bool[])
            n299 = property on="Z mm/rev" class="DigNum (strict)"() -> ("Value"=w643:dbl)  [unwired: 2 in, 2 out]
            n300 = Index Array(array=w627, index=0) -> (element=w625:bool)
            n301 = Multiply(x=w644, y=w643) -> (x*y=w642:dbl)
            n302 = property on="Z in Motion" class="Bool (strict)"("Val(Sgnl)"=w625) -> ()  [unwired: 2 in, 2 out]
            n303 = Add(x=w642, y=w641) -> (x+y=w638:dbl)
            n304 = property on="Z Position mm PV" class="DigNum (strict)"("Val(Sgnl)"=w638) -> ()  [unwired: 2 in, 2 out]
          }
          frame #1 {
            n305 = property on="Z Scan" class="Bool (strict)"() -> ("Value"=w660:bool)  [unwired: 2 in, 2 out]
            n306 = Or(x=w659, y=w660) -> (x .or. y?=w661:bool)
            n307 = case shown="True" w661 {
              frame #0 {
                n308 = property on="Z Go" class="Bool"("DisabledEnum"=T1."Enabled" ("Disabled")) -> ()  [unwired: 2 in, 2 out]
                n309 = property on="Z Scan OK" class="Bool"("DisabledEnum"=T1."Enabled" ("Disabled")) -> ()  [unwired: 2 in, 2 out]
              }
              frame #1 {
                n310 = property on="Z Go" class="Bool"("DisabledEnum"=T1."Disabled and Grayed Out" ("Disabled")) -> ()  [unwired: 2 in, 2 out]
                n311 = property on="Z Scan OK" class="Bool"("DisabledEnum"=T1."Disabled and Grayed Out" ("Disabled")) -> ()  [unwired: 2 in, 2 out]
              }
            }
          }
          frame #2 {
            n312 = case shown="False" w670 {
              tunnel: w671 -> [w677 w681]
              tunnel: [w678 w681] -> w672
              tunnel: [w679 w680] -> w673
              tunnel: w674 -> [w676 w680]
              frame #0 {
                n313 = call "mDrive Send Command.vi"("error in (no error)"=w676, "Command"=T2."Stop", "VISA resource name"=w677) -> ("error out"=w679:errorcluster, "VISA resource name out"=w678:refnum<visa-resource-name>)  [unwired: 4 in, 1 out]
              }
              frame #1 {
              }
            }
          }
          frame #3 {
            n314 = property on="Z Backlash corr" class="Bool (strict)"() -> ("Value"=w688:bool)  [unwired: 2 in, 2 out]
            n315 = Implies(1:w687, 2:w688) -> (0:w686:bool)
            n316 = case shown="False" w686 {
              tunnel: w685 -> [w695 w748]
              tunnel: w684 -> [w694 w749]
              tunnel: [w693 w748] -> w683
              tunnel: [w692 w749] -> w682
              frame #0 {
                # "Backlash"
                n317 = flat-sequence {
                  tunnel: [w710] -> w707
                  tunnel: [w712] -> w706
                  tunnel: [w711] -> w705
                  tunnel: w695 -> [w709]
                  tunnel: w694 -> [w708]
                  tunnel: w707 -> [w720]
                  tunnel: [w720] -> w704
                  tunnel: w706 -> [w719]
                  tunnel: w705 -> [w718]
                  tunnel: [w717] -> w703
                  tunnel: [w716] -> w702
                  tunnel: [w715] -> w691
                  tunnel: w704 -> [w730]
                  tunnel: w703 -> [w729]
                  tunnel: w702 -> [w727]
                  tunnel: [w728] -> w701
                  tunnel: [w727] -> w700
                  tunnel: [w726] -> w697
                  tunnel: [w725] -> w696
                  tunnel: w691 -> [w725]
                  tunnel: w701 -> [w741]
                  tunnel: w700 -> [w734]
                  tunnel: [w741] -> w699
                  tunnel: [w740] -> w698
                  tunnel: w697 -> [w740]
                  tunnel: w696 -> [w736]
                  tunnel: [w735] -> w689
                  tunnel: w699 -> [w745]
                  tunnel: w698 -> [w744]
                  tunnel: [w743] -> w693
                  tunnel: [w742] -> w690
                  tunnel: w689 -> [w742]
                  tunnel: [w747] -> w692
                  tunnel: w690 -> [w747]
                  frame #0 {
                    n318 = property on="Z Backlash steps/sec" class="DigNum (strict)"() -> ("Value"=w710:i32)  [unwired: 2 in, 2 out]
                    n319 = Number To Decimal String(number=w710) -> (decimal integer string=w713:string)  [unwired: 1 in]
                    n320 = call "mDrive Send Command.vi"("error in (no error)"=w709, "Extra"=w713, "Command"=T2."Max Velocity", "VISA resource name"=w708) -> ("error out"=w711:errorcluster, "VISA resource name out"=w712:refnum<visa-resource-name>)  [unwired: 3 in, 1 out]
                  }
                  frame #1 {
                    n321 = property on="Z Backlash" class="DigNum (strict)"() -> ("Value"=w715:i32)  [unwired: 2 in, 2 out]
                    n322 = Number To Decimal String(number=w715) -> (decimal integer string=w721:string)  [unwired: 1 in]
                    n323 = call "mDrive Send Command.vi"("error in (no error)"=w718, "Extra"=w721, "Command"=T2."Move to Relative Position", "VISA resource name"=w719) -> ("error out"=w717:errorcluster, "VISA resource name out"=w716:refnum<visa-resource-name>)  [unwired: 3 in, 1 out]
                  }
                  frame #2 {
                    n324 = To Double Precision Float(number=w725) -> (double precision float=w723:dbl)
                    n325 = To Double Precision Float(number=w730) -> (double precision float=w732:dbl)
                    n326 = Absolute Value(x=w723) -> (abs(x)=w724:dbl)
                    n327 = Divide(x=w724, y=w732) -> (x/y=w733:dbl)
                    n328 = Add(x=w733, y=0.5) -> (x+y=w726:dbl)
                    n329 = call "Time Delay18"("error in (no error)"=w729, "Delay Time (s)"=w726) -> ("error out"=w728:errorcluster)  [unwired: 9 in]
                  }
                  frame #3 {
                    n330 = Negate(x=w736) -> (-x=w737:i32)
                    n331 = Number To Decimal String(number=w737) -> (decimal integer string=w738:string)  [unwired: 1 in]
                    n332 = call "mDrive Send Command.vi"("Extra"=w738, "Command"=T2."Move to Relative Position", "VISA resource name"=w734) -> ("VISA resource name out"=w735:refnum<visa-resource-name>)  [unwired: 4 in, 2 out]
                  }
                  frame #4 {
                    n333 = call "Time Delay19"("error in (no error)"=w745, "Delay Time (s)"=w744) -> ("error out"=w743:errorcluster)  [unwired: 9 in]
                  }
                  frame #5 {
                    n334 = property on="Z Backlash corr" class="Bool (strict)"("Val(Sgnl)"=FALSE ("Value (Signaling)")) -> ()  [unwired: 2 in, 2 out]
                  }
                }
              }
              frame #1 {
              }
            }
          }
        }
        n335 = flat-sequence {
          tunnel: [w531] -> w456
          tunnel: [w507] -> w455
          tunnel: [w520] -> w454
          tunnel: [w498] -> w453
          tunnel: w441 -> [w497]
          tunnel: w440 -> [w496]
          tunnel: w456 -> [w537]
          tunnel: [w537] -> w452
          tunnel: w455 -> [w536]
          tunnel: [w536] -> w451
          tunnel: w454 -> [w535]
          tunnel: [w535] -> w450
          tunnel: w453 -> [w532]
          tunnel: [w532] -> w449
          tunnel: w452 -> [w544]
          tunnel: [w545] -> w448
          tunnel: w451 -> [w547]
          tunnel: [w546] -> w447
          tunnel: w450 -> [w543]
          tunnel: [w542] -> w446
          tunnel: w449 -> [w542]
          tunnel: w448 -> [w557]
          tunnel: w447 -> [w558]
          tunnel: w446 -> [w560]
          tunnel: [w556] -> w438
          tunnel: [w555] -> w439
          frame #0 {
            w502 = 0.05 ("Delay Time (s)")
            n336 = property on="R Step SP" class="DigNum (strict)"() -> ("Maximum"=w522:dbl)  [unwired: 2 in, 2 out]
            n337 = property on="R Step SP" class="DigNum (strict)"() -> ("Minimum"=w524:dbl)  [unwired: 2 in, 2 out]
            n338 = property on="R steps/rev" class="DigNum (strict)"() -> ("Value"=w518:u32)  [unwired: 2 in, 2 out]
            n339 = property on="R offset deg" class="DigNum (strict)"() -> ("Value"=w514:dbl)  [unwired: 2 in, 2 out]
            n340 = To Long Integer(number=w522) -> (32bit integer=w521:i32)
            n341 = To Long Integer(number=w524) -> (32bit integer=w523:i32)
            n342 = To Double Precision Float(number=w518) -> (double precision float=w519:dbl)
            n343 = call "mDrive Send Command.vi"("error in (no error)"=w496, "Extra"="P", "Command"=T2."Print Parameter", "VISA resource name"=w497) -> ("error out"=w526:errorcluster, "read buffer"=w530:string, "VISA resource name out"=w528:refnum<visa-resource-name>)  [unwired: 3 in]
            n344 = call "Time Delay21"("error in (no error)"=w526, "Delay Time (s)"=w502) -> ("error out"=w525:errorcluster)  [unwired: 9 in]
            n345 = Decimal String To Number(string=w530, offset=0) -> (number=w510:i32)  [unwired: 1 in, 1 out]
            n346 = To Long Integer(number=w510) -> (32bit integer=w512:i32)
            n347 = property on="R Step PV" class="DigNum (strict)"("Val(Sgnl)"=w512) -> ()  [unwired: 2 in, 2 out]
            n348 = call "mDrive Send Command.vi"("error in (no error)"=w525, "Extra"="MV", "Command"=T2."Print Parameter", "VISA resource name"=w528) -> ("error out"=w527:errorcluster, "read buffer"=w508:string, "VISA resource name out"=w531:refnum<visa-resource-name>)  [unwired: 3 in]
            n349 = call "Time Delay20"("error in (no error)"=w527, "Delay Time (s)"=w502) -> ("error out"=w507:errorcluster)  [unwired: 9 in]
            n350 = In Range and Coerce(upper limit=w521, x=w512, lower limit=w523) -> (In Range?=w520:bool)  [unwired: 1 out]
            n351 = To Double Precision Float(number=w512) -> (double precision float=w513:dbl)
            n352 = Decimal String To Number(string=w508, offset=0 ("offset (0)")) -> (number=w501:i32)  [unwired: 1 in, 1 out]
            n353 = property on="R in Range" class="Bool (strict)"("Val(Sgnl)"=w520) -> ()  [unwired: 2 in, 2 out]
            n354 = Divide(x=w513, y=w519) -> (x/y=w517:dbl)
            n355 = Number To Boolean Array(number=w501) -> (Boolean array=w500:bool[])
            n356 = property on="R deg/rev" class="DigNum (strict)"() -> ("Value"=w516:dbl)  [unwired: 2 in, 2 out]
            n357 = Index Array(array=w500, index=0) -> (element=w498:bool)
            n358 = Multiply(x=w517, y=w516) -> (x*y=w515:dbl)
            n359 = property on="R in Motion" class="Bool (strict)"("Val(Sgnl)"=w498) -> ()  [unwired: 2 in, 2 out]
            n360 = Add(x=w515, y=w514) -> (x+y=w511:dbl)
            n361 = property on="R Position deg PV" class="DigNum (strict)"("Val(Sgnl)"=w511) -> ()  [unwired: 2 in, 2 out]
          }
          frame #1 {
            n362 = property on="R Scan" class="Bool (strict)"() -> ("Value"=w533:bool)  [unwired: 2 in, 2 out]
            n363 = Or(x=w532, y=w533) -> (x .or. y?=w534:bool)
            n364 = case shown="True" w534 {
              frame #0 {
                n365 = property on="R Go" class="Bool"("DisabledEnum"=T1."Enabled" ("Disabled")) -> ()  [unwired: 2 in, 2 out]
                n366 = property on="R Scan OK" class="Bool"("DisabledEnum"=T1."Enabled" ("Disabled")) -> ()  [unwired: 2 in, 2 out]
              }
              frame #1 {
                n367 = property on="R Go" class="Bool"("DisabledEnum"=T1."Disabled and Grayed Out" ("Disabled")) -> ()  [unwired: 2 in, 2 out]
                n368 = property on="R Scan OK" class="Bool"("DisabledEnum"=T1."Disabled and Grayed Out" ("Disabled")) -> ()  [unwired: 2 in, 2 out]
              }
            }
          }
          frame #2 {
            n369 = case shown="False" w543 {
              tunnel: w544 -> [w550 w554]
              tunnel: [w551 w554] -> w545
              tunnel: [w552 w553] -> w546
              tunnel: w547 -> [w549 w553]
              frame #0 {
                n370 = call "mDrive Send Command.vi"("error in (no error)"=w549, "Command"=T2."Stop", "VISA resource name"=w550) -> ("error out"=w552:errorcluster, "VISA resource name out"=w551:refnum<visa-resource-name>)  [unwired: 4 in, 1 out]
              }
              frame #1 {
              }
            }
          }
          frame #3 {
            n371 = property on="R Backlash corr" class="Bool (strict)"() -> ("Value"=w561:bool)  [unwired: 2 in, 2 out]
            n372 = Implies(1:w560, 2:w561) -> (0:w559:bool)
            n373 = case shown="False" w559 {
              tunnel: w558 -> [w568 w621]
              tunnel: w557 -> [w567 w622]
              tunnel: [w566 w621] -> w556
              tunnel: [w565 w622] -> w555
              frame #0 {
                # "Backlash"
                n374 = flat-sequence {
                  tunnel: [w583] -> w580
                  tunnel: [w585] -> w579
                  tunnel: [w584] -> w578
                  tunnel: w568 -> [w582]
                  tunnel: w567 -> [w581]
                  tunnel: w580 -> [w593]
                  tunnel: [w593] -> w577
                  tunnel: w579 -> [w592]
                  tunnel: w578 -> [w591]
                  tunnel: [w590] -> w576
                  tunnel: [w589] -> w575
                  tunnel: [w588] -> w564
                  tunnel: w577 -> [w603]
                  tunnel: w576 -> [w602]
                  tunnel: w575 -> [w600]
                  tunnel: [w601] -> w574
                  tunnel: [w600] -> w573
                  tunnel: [w599] -> w570
                  tunnel: [w598] -> w569
                  tunnel: w564 -> [w598]
                  tunnel: w574 -> [w614]
                  tunnel: w573 -> [w607]
                  tunnel: [w614] -> w572
                  tunnel: [w613] -> w571
                  tunnel: w570 -> [w613]
                  tunnel: w569 -> [w609]
                  tunnel: [w608] -> w562
                  tunnel: w572 -> [w618]
                  tunnel: w571 -> [w617]
                  tunnel: [w616] -> w566
                  tunnel: [w615] -> w563
                  tunnel: w562 -> [w615]
                  tunnel: [w620] -> w565
                  tunnel: w563 -> [w620]
                  frame #0 {
                    n375 = property on="R Backlash steps/sec" class="DigNum (strict)"() -> ("Value"=w583:i32)  [unwired: 2 in, 2 out]
                    n376 = Number To Decimal String(number=w583) -> (decimal integer string=w586:string)  [unwired: 1 in]
                    n377 = call "mDrive Send Command.vi"("error in (no error)"=w582, "Extra"=w586, "Command"=T2."Max Velocity", "VISA resource name"=w581) -> ("error out"=w584:errorcluster, "VISA resource name out"=w585:refnum<visa-resource-name>)  [unwired: 3 in, 1 out]
                  }
                  frame #1 {
                    n378 = property on="R Backlash" class="DigNum (strict)"() -> ("Value"=w588:i32)  [unwired: 2 in, 2 out]
                    n379 = Number To Decimal String(number=w588) -> (decimal integer string=w594:string)  [unwired: 1 in]
                    n380 = call "mDrive Send Command.vi"("error in (no error)"=w591, "Extra"=w594, "Command"=T2."Move to Relative Position", "VISA resource name"=w592) -> ("error out"=w590:errorcluster, "VISA resource name out"=w589:refnum<visa-resource-name>)  [unwired: 3 in, 1 out]
                  }
                  frame #2 {
                    n381 = To Double Precision Float(number=w598) -> (double precision float=w596:dbl)
                    n382 = To Double Precision Float(number=w603) -> (double precision float=w605:dbl)
                    n383 = Absolute Value(x=w596) -> (abs(x)=w597:dbl)
                    n384 = Divide(x=w597, y=w605) -> (x/y=w606:dbl)
                    n385 = Add(x=w606, y=0.3) -> (x+y=w599:dbl)
                    n386 = call "Time Delay22"("error in (no error)"=w602, "Delay Time (s)"=w599) -> ("error out"=w601:errorcluster)  [unwired: 9 in]
                  }
                  frame #3 {
                    n387 = Negate(x=w609) -> (-x=w610:i32)
                    n388 = Number To Decimal String(number=w610) -> (decimal integer string=w611:string)  [unwired: 1 in]
                    n389 = call "mDrive Send Command.vi"("Extra"=w611, "Command"=T2."Move to Relative Position", "VISA resource name"=w607) -> ("VISA resource name out"=w608:refnum<visa-resource-name>)  [unwired: 4 in, 2 out]
                  }
                  frame #4 {
                    n390 = call "Time Delay23"("error in (no error)"=w618, "Delay Time (s)"=w617) -> ("error out"=w616:errorcluster)  [unwired: 9 in]
                  }
                  frame #5 {
                    n391 = property on="R Backlash corr" class="Bool (strict)"("Val(Sgnl)"=FALSE ("Value (Signaling)")) -> ()  [unwired: 2 in, 2 out]
                  }
                }
              }
              frame #1 {
              }
            }
          }
        }
        n392 = property on="X Position mm PV" class="DigNum (strict)"() -> ("Value"=w433:dbl)  [unwired: 2 in, 2 out]
        n393 = property on="Y Position mm PV" class="DigNum (strict)"() -> ("Value"=w435:dbl)  [unwired: 2 in, 2 out]
        n394 = property on="Z Position mm PV" class="DigNum (strict)"() -> ("Value"=w432:dbl)  [unwired: 2 in, 2 out]
        n395 = property on="R Position deg PV" class="DigNum (strict)"() -> ("Value"=w434:dbl)  [unwired: 2 in, 2 out]
        n396 = call "Build XY Graph"("Y Input"=w435, "X Input"=w433) -> ("XY Graph"=→"XY Graph":cluster{"Y":dbl[], "Y":dbl[]}[])  [unwired: 8 in, 1 out]
        n397 = call "Build XY Graph2"("Y Input"=w434, "X Input"=w432) -> ("XY Graph"=→"XY Graph 2":cluster{"Y":dbl[], "Y":dbl[]}[])  [unwired: 8 in, 1 out]
      }
      event #1 {
        n398 = event-data() -> ()  [unwired: 1 in, 5 out]
        n399 = property on="Z steps/rev" class="DigNum (strict)"() -> ("Value"=w1015:u32)  [unwired: 2 in, 2 out]
        n400 = property on="R steps/rev" class="DigNum (strict)"() -> ("Value"=w1006:u32)  [unwired: 2 in, 2 out]
        n401 = property on="X steps/rev" class="DigNum (strict)"() -> ("Value"=w1024:u32)  [unwired: 2 in, 2 out]
        n402 = property on="Y steps/rev" class="DigNum (strict)"() -> ("Value"=w1033:u32)  [unwired: 2 in, 2 out]
        n403 = property on="Z offset mm" class="DigNum (strict)"() -> ("Value"=w1013:dbl)  [unwired: 2 in, 2 out]
        n404 = property on="R offset deg" class="DigNum (strict)"() -> ("Value"=w1004:dbl)  [unwired: 2 in, 2 out]
        n405 = property on="X offset mm" class="DigNum (strict)"() -> ("Value"=w1022:dbl)  [unwired: 2 in, 2 out]
        n406 = property on="Y offset mm" class="DigNum (strict)"() -> ("Value"=w1031:dbl)  [unwired: 2 in, 2 out]
        n407 = property on="Reset R Position deg" class="DigNum (strict)"() -> ("Value"=w1012:dbl)  [unwired: 2 in, 2 out]
        n408 = property on="Reset Z Position mm" class="DigNum (strict)"() -> ("Value"=w1021:dbl)  [unwired: 2 in, 2 out]
        n409 = property on="Reset X Position mm" class="DigNum (strict)"() -> ("Value"=w1030:dbl)  [unwired: 2 in, 2 out]
        n410 = property on="Reset Y Position mm" class="DigNum (strict)"() -> ("Value"=w1039:dbl)  [unwired: 2 in, 2 out]
        n411 = To Double Precision Float(number=w1024) -> (double precision float=w1027:dbl)
        n412 = To Double Precision Float(number=w1033) -> (double precision float=w1036:dbl)
        n413 = Subtract(x=w1021, y=w1013) -> (x-y=w1020:dbl)
        n414 = Subtract(x=w1012, y=w1004) -> (x-y=w1011:dbl)
        n415 = Subtract(x=w1030, y=w1022) -> (x-y=w1029:dbl)
        n416 = Subtract(x=w1039, y=w1031) -> (x-y=w1038:dbl)
        n417 = property on="R deg/rev" class="DigNum (strict)"() -> ("Value"=w1005:dbl)  [unwired: 2 in, 2 out]
        n418 = property on="Z mm/rev" class="DigNum (strict)"() -> ("Value"=w1014:dbl)  [unwired: 2 in, 2 out]
        n419 = property on="X mm/rev" class="DigNum (strict)"() -> ("Value"=w1023:dbl)  [unwired: 2 in, 2 out]
        n420 = property on="Y mm/rev" class="DigNum (strict)"() -> ("Value"=w1032:dbl)  [unwired: 2 in, 2 out]
        n421 = Divide(x=w1029, y=w1023) -> (x/y=w1028:dbl)
        n422 = Divide(x=w1038, y=w1032) -> (x/y=w1037:dbl)
        n423 = Divide(x=w1020, y=w1014) -> (x/y=w1019:dbl)
        n424 = Divide(x=w1011, y=w1005) -> (x/y=w1010:dbl)
        n425 = To Double Precision Float(number=w1015) -> (double precision float=w1018:dbl)
        n426 = To Double Precision Float(number=w1006) -> (double precision float=w1009:dbl)
        n427 = Multiply(x=w1019, y=w1018) -> (x*y=w1017:dbl)
        n428 = Multiply(x=w1010, y=w1009) -> (x*y=w1008:dbl)
        n429 = Multiply(x=w1028, y=w1027) -> (x*y=w1026:dbl)
        n430 = Multiply(x=w1037, y=w1036) -> (x*y=w1035:dbl)
        n431 = To Long Integer(number=w1017) -> (32bit integer=w1016:i32)
        n432 = To Long Integer(number=w1008) -> (32bit integer=w1007:i32)
        n433 = To Long Integer(number=w1026) -> (32bit integer=w1025:i32)
        n434 = To Long Integer(number=w1035) -> (32bit integer=w1034:i32)
        n435 = property on="Reset Z Motor Steps" class="DigNum (strict)"("Val(Sgnl)"=w1016) -> ()  [unwired: 2 in, 2 out]
        n436 = property on="Reset R Motor Steps" class="DigNum (strict)"("Val(Sgnl)"=w1007) -> ()  [unwired: 2 in, 2 out]
        n437 = property on="Reset X Motor Steps" class="DigNum (strict)"("Val(Sgnl)"=w1025) -> ()  [unwired: 2 in, 2 out]
        n438 = property on="Reset Y Motor Steps" class="DigNum (strict)"("Val(Sgnl)"=w1034) -> ()  [unwired: 2 in, 2 out]
      }
      event #2 {
        n439 = event-data() -> ()  [unwired: 1 in, 5 out]
        n440 = property on="X Step SP" class="DigNum (strict)"() -> ("Value"=w1064:i32)  [unwired: 2 in, 2 out]
        n441 = property on="Z Step SP" class="DigNum (strict)"() -> ("Value"=w1056:i32)  [unwired: 2 in, 2 out]
        n442 = property on="Y Step SP" class="DigNum (strict)"() -> ("Value"=w1072:i32)  [unwired: 2 in, 2 out]
        n443 = property on="R Step SP" class="DigNum (strict)"() -> ("Value"=w1048:i32)  [unwired: 2 in, 2 out]
        n444 = property on="X steps/rev" class="DigNum (strict)"() -> ("Value"=w1089:u32)  [unwired: 2 in, 2 out]
        n445 = property on="X steps/rev" class="DigNum (strict)"() -> ("Value"=w1062:u32)  [unwired: 2 in, 2 out]
        n446 = property on="Z steps/rev" class="DigNum (strict)"() -> ("Value"=w1083:u32)  [unwired: 2 in, 2 out]
        n447 = property on="Z steps/rev" class="DigNum (strict)"() -> ("Value"=w1054:u32)  [unwired: 2 in, 2 out]
        n448 = property on="Y steps/rev" class="DigNum (strict)"() -> ("Value"=w1095:u32)  [unwired: 2 in, 2 out]
        n449 = property on="Y steps/rev" class="DigNum (strict)"() -> ("Value"=w1070:u32)  [unwired: 2 in, 2 out]
        n450 = property on="R steps/rev" class="DigNum (strict)"() -> ("Value"=w1077:u32)  [unwired: 2 in, 2 out]
        n451 = property on="R steps/rev" class="DigNum (strict)"() -> ("Value"=w1046:u32)  [unwired: 2 in, 2 out]
        n452 = property on="X offset mm" class="DigNum (strict)"() -> ("Value"=w1061:dbl)  [unwired: 2 in, 2 out]
        n453 = property on="Z offset mm" class="DigNum (strict)"() -> ("Value"=w1053:dbl)  [unwired: 2 in, 2 out]
        n454 = property on="Y offset mm" class="DigNum (strict)"() -> ("Value"=w1069:dbl)  [unwired: 2 in, 2 out]
        n455 = property on="R offset deg" class="DigNum (strict)"() -> ("Value"=w1045:dbl)  [unwired: 2 in, 2 out]
        n456 = property on="X Velocity SP step/sec" class="DigNum (strict)"() -> ("Value"=w1091:i32)  [unwired: 2 in, 2 out]
        n457 = property on="Z Velocity SP step/sec" class="DigNum (strict)"() -> ("Value"=w1085:i32)  [unwired: 2 in, 2 out]
        n458 = property on="Y Velocity SP step/sec" class="DigNum (strict)"() -> ("Value"=w1097:i32)  [unwired: 2 in, 2 out]
        n459 = property on="R Velocity SP step/sec" class="DigNum (strict)"() -> ("Value"=w1079:i32)  [unwired: 2 in, 2 out]
        n460 = To Double Precision Float(number=w1064) -> (double precision float=w1065:dbl)
        n461 = To Double Precision Float(number=w1062) -> (double precision float=w1068:dbl)
        n462 = To Double Precision Float(number=w1083) -> (double precision float=w1088:dbl)
        n463 = To Double Precision Float(number=w1056) -> (double precision float=w1057:dbl)
        n464 = To Double Precision Float(number=w1054) -> (double precision float=w1060:dbl)
        n465 = To Double Precision Float(number=w1095) -> (double precision float=w1100:dbl)
        n466 = To Double Precision Float(number=w1072) -> (double precision float=w1073:dbl)
        n467 = To Double Precision Float(number=w1070) -> (double precision float=w1076:dbl)
        n468 = To Double Precision Float(number=w1077) -> (double precision float=w1082:dbl)
        n469 = To Double Precision Float(number=w1048) -> (double precision float=w1049:dbl)
        n470 = To Double Precision Float(number=w1046) -> (double precision float=w1052:dbl)
        n471 = Divide(x=w1049, y=w1052) -> (x/y=w1051:dbl)
        n472 = Divide(x=w1065, y=w1068) -> (x/y=w1067:dbl)
        n473 = Divide(x=w1057, y=w1060) -> (x/y=w1059:dbl)
        n474 = Divide(x=w1073, y=w1076) -> (x/y=w1075:dbl)
        n475 = To Double Precision Float(number=w1079) -> (double precision float=w1080:dbl)
        n476 = To Double Precision Float(number=w1091) -> (double precision float=w1092:dbl)
        n477 = To Double Precision Float(number=w1089) -> (double precision float=w1094:dbl)
        n478 = To Double Precision Float(number=w1085) -> (double precision float=w1086:dbl)
        n479 = To Double Precision Float(number=w1097) -> (double precision float=w1098:dbl)
        n480 = property on="R deg/rev" class="DigNum (strict)"() -> ("Value"=w1044:dbl)  [unwired: 2 in, 2 out]
        n481 = property on="X mm/rev" class="DigNum (strict)"() -> ("Value"=w1042:dbl)  [unwired: 2 in, 2 out]
        n482 = property on="Z mm/rev" class="DigNum (strict)"() -> ("Value"=w1043:dbl)  [unwired: 2 in, 2 out]
        n483 = property on="Y mm/rev" class="DigNum (strict)"() -> ("Value"=w1041:dbl)  [unwired: 2 in, 2 out]
        n484 = Divide(x=w1092, y=w1094) -> (x/y=w1093:dbl)
        n485 = Multiply(x=w1067, y=w1042) -> (x*y=w1066:dbl)
        n486 = Divide(x=w1086, y=w1088) -> (x/y=w1087:dbl)
        n487 = Multiply(x=w1059, y=w1043) -> (x*y=w1058:dbl)
        n488 = Divide(x=w1098, y=w1100) -> (x/y=w1099:dbl)
        n489 = Multiply(x=w1075, y=w1041) -> (x*y=w1074:dbl)
        n490 = Divide(x=w1080, y=w1082) -> (x/y=w1081:dbl)
        n491 = Multiply(x=w1051, y=w1044) -> (x*y=w1050:dbl)
        n492 = Multiply(x=w1093, y=w1042) -> (x*y=w1090:dbl)
        n493 = Add(x=w1066, y=w1061) -> (x+y=w1063:dbl)
        n494 = Multiply(x=w1087, y=w1043) -> (x*y=w1084:dbl)
        n495 = Add(x=w1058, y=w1053) -> (x+y=w1055:dbl)
        n496 = Multiply(x=w1099, y=w1041) -> (x*y=w1096:dbl)
        n497 = Add(x=w1074, y=w1069) -> (x+y=w1071:dbl)
        n498 = Multiply(x=w1081, y=w1044) -> (x*y=w1078:dbl)
        n499 = Add(x=w1050, y=w1045) -> (x+y=w1047:dbl)
        n500 = Absolute Value(x=w1078) -> (abs(x)=w1040:dbl)
        n501 = property on="X Velocity MV mm/sec" class="DigNum (strict)"("Val(Sgnl)"=w1090) -> ()  [unwired: 2 in, 2 out]
        n502 = property on="X Position MV mm" class="DigNum (strict)"("Val(Sgnl)"=w1063) -> ()  [unwired: 2 in, 2 out]
        n503 = property on="Z Velocity MV mm/sec" class="DigNum (strict)"("Val(Sgnl)"=w1084) -> ()  [unwired: 2 in, 2 out]
        n504 = property on="Z Position MV mm" class="DigNum (strict)"("Val(Sgnl)"=w1055) -> ()  [unwired: 2 in, 2 out]
        n505 = property on="Y Velocity MV mm/sec" class="DigNum (strict)"("Val(Sgnl)"=w1096) -> ()  [unwired: 2 in, 2 out]
        n506 = property on="Y Position MV mm" class="DigNum (strict)"("Val(Sgnl)"=w1071) -> ()  [unwired: 2 in, 2 out]
        n507 = property on="R Position MV deg" class="DigNum (strict)"("Val(Sgnl)"=w1047) -> ()  [unwired: 2 in, 2 out]
        n508 = property on="R Velocity MVdeg/sec" class="DigNum (strict)"("Val(Sgnl)"=w1040) -> ()  [unwired: 2 in, 2 out]
      }
      event #3 {
        n509 = event-data() -> ()  [unwired: 1 in, 5 out]
        n510 = property on="X Step PV" class="DigNum (strict)"() -> ("Value"=w1165:i32)  [unwired: 2 in, 2 out]
        n511 = property on="Y Step PV" class="DigNum (strict)"() -> ("Value"=w1151:i32)  [unwired: 2 in, 2 out]
        n512 = property on="Z Step PV" class="DigNum (strict)"() -> ("Value"=w1138:i32)  [unwired: 2 in, 2 out]
        n513 = property on="R Step PV" class="DigNum (strict)"() -> ("Value"=w1124:i32)  [unwired: 2 in, 2 out]
        n514 = property on="X Step SP" class="DigNum (strict)"() -> ("Minimum"=w1172:dbl)  [unwired: 2 in, 2 out]
        n515 = property on="X Step SP" class="DigNum (strict)"() -> ("Maximum"=w1171:dbl)  [unwired: 2 in, 2 out]
        n516 = property on="Y Step SP" class="DigNum (strict)"() -> ("Minimum"=w1158:dbl)  [unwired: 2 in, 2 out]
        n517 = property on="Y Step SP" class="DigNum (strict)"() -> ("Maximum"=w1157:dbl)  [unwired: 2 in, 2 out]
        n518 = property on="Z Step SP" class="DigNum (strict)"() -> ("Minimum"=w1145:dbl)  [unwired: 2 in, 2 out]
        n519 = property on="Z Step SP" class="DigNum (strict)"() -> ("Maximum"=w1144:dbl)  [unwired: 2 in, 2 out]
        n520 = property on="R Step SP" class="DigNum (strict)"() -> ("Minimum"=w1129:dbl)  [unwired: 2 in, 2 out]
        n521 = property on="R Step SP" class="DigNum (strict)"() -> ("Maximum"=w1132:dbl)  [unwired: 2 in, 2 out]
        n522 = property on="Z steps/rev" class="DigNum (strict)"() -> ("Value"=w1140:u32)  [unwired: 2 in, 2 out]
        n523 = property on="R steps/rev" class="DigNum (strict)"() -> ("Value"=w1126:u32)  [unwired: 2 in, 2 out]
        n524 = property on="X steps/rev" class="DigNum (strict)"() -> ("Value"=w1167:u32)  [unwired: 2 in, 2 out]
        n525 = property on="Y steps/rev" class="DigNum (strict)"() -> ("Value"=w1153:u32)  [unwired: 2 in, 2 out]
        n526 = To Double Precision Float(number=w1165) -> (double precision float=w1118:dbl)
        n527 = To Double Precision Float(number=w1151) -> (double precision float=w1117:dbl)
        n528 = To Double Precision Float(number=w1138) -> (double precision float=w1116:dbl)
        n529 = To Double Precision Float(number=w1124) -> (double precision float=w1115:dbl)
        n530 = Subtract(x=w1172, y=w1118) -> (x-y=w1173:dbl)
        n531 = Subtract(x=w1171, y=w1118) -> (x-y=w1170:dbl)
        n532 = Subtract(x=w1158, y=w1117) -> (x-y=w1159:dbl)
        n533 = Subtract(x=w1157, y=w1117) -> (x-y=w1156:dbl)
        n534 = Subtract(x=w1145, y=w1116) -> (x-y=w1146:dbl)
        n535 = Subtract(x=w1144, y=w1116) -> (x-y=w1143:dbl)
        n536 = Subtract(x=w1129, y=w1115) -> (x-y=w1130:dbl)
        n537 = Subtract(x=w1132, y=w1115) -> (x-y=w1131:dbl)
        n538 = property on="Z Scan Length SP steps" class="DigNum (strict)"() -> ("Value"=w1141:i32)  [unwired: 2 in, 2 out]
        n539 = property on="R Scan Length SP steps" class="DigNum (strict)"() -> ("Value"=w1127:i32)  [unwired: 2 in, 2 out]
        n540 = To Double Precision Float(number=w1126) -> (double precision float=w1123:dbl)
        n541 = property on="X Scan Length SP steps" class="DigNum (strict)"() -> ("Value"=w1163:i32)  [unwired: 2 in, 2 out]
        n542 = To Double Precision Float(number=w1167) -> (double precision float=w1164:dbl)
        n543 = property on="Y Scan Length SP steps" class="DigNum (strict)"() -> ("Value"=w1154:i32)  [unwired: 2 in, 2 out]
        n544 = To Double Precision Float(number=w1153) -> (double precision float=w1108:dbl)
        n545 = property on="Z Scan Velocity SP steps/sec" class="DigNum (strict)"() -> ("Value"=w1136:i32)  [unwired: 2 in, 2 out]
        n546 = property on="R Scan Velocity SP steps/sec" class="DigNum (strict)"() -> ("Value"=w1122:i32)  [unwired: 2 in, 2 out]
        n547 = property on="X Scan Velocity SP steps/sec" class="DigNum (strict)"() -> ("Value"=w1168:i32)  [unwired: 2 in, 2 out]
        n548 = property on="Y Scan Velocity SP steps/sec" class="DigNum (strict)"() -> ("Value"=w1150:i32)  [unwired: 2 in, 2 out]
        n549 = To Double Precision Float(number=w1141) -> (double precision float=w1114:dbl)
        n550 = To Double Precision Float(number=w1140) -> (double precision float=w1137:dbl)
        n551 = To Double Precision Float(number=w1127) -> (double precision float=w1112:dbl)
        n552 = property on="X Scan Length SP steps" class="DigNum (strict)"("Minimum"=w1173) -> ()  [unwired: 2 in, 2 out]
        n553 = property on="X Scan Length SP steps" class="DigNum (strict)"("Maximum"=w1170) -> ()  [unwired: 2 in, 2 out]
        n554 = property on="Y Scan Length SP steps" class="DigNum (strict)"("Minimum"=w1159) -> ()  [unwired: 2 in, 2 out]
        n555 = property on="Y Scan Length SP steps" class="DigNum (strict)"("Maximum"=w1156) -> ()  [unwired: 2 in, 2 out]
        n556 = property on="Z Scan Length SP steps" class="DigNum (strict)"("Minimum"=w1146) -> ()  [unwired: 2 in, 2 out]
        n557 = property on="Z Scan Length SP steps" class="DigNum (strict)"("Maximum"=w1143) -> ()  [unwired: 2 in, 2 out]
        n558 = property on="R Scan Length SP steps" class="DigNum (strict)"("Minimum"=w1130) -> ()  [unwired: 2 in, 2 out]
        n559 = property on="R Scan Length SP steps" class="DigNum (strict)"("Maximum"=w1131) -> ()  [unwired: 2 in, 2 out]
        n560 = To Double Precision Float(number=w1163) -> (double precision float=w1103:dbl)
        n561 = To Double Precision Float(number=w1154) -> (double precision float=w1107:dbl)
        n562 = Divide(x=w1112, y=w1123) -> (x/y=w1128:dbl)
        n563 = Divide(x=w1114, y=w1137) -> (x/y=w1142:dbl)
        n564 = Divide(x=w1103, y=w1164) -> (x/y=w1162:dbl)
        n565 = Divide(x=w1107, y=w1108) -> (x/y=w1155:dbl)
        n566 = To Double Precision Float(number=w1122) -> (double precision float=w1111:dbl)
        n567 = property on="R deg/rev" class="DigNum (strict)"() -> ("Value"=w1125:dbl)  [unwired: 2 in, 2 out]
        n568 = To Double Precision Float(number=w1136) -> (double precision float=w1113:dbl)
        n569 = To Double Precision Float(number=w1168) -> (double precision float=w1102:dbl)
        n570 = To Double Precision Float(number=w1150) -> (double precision float=w1106:dbl)
        n571 = property on="Z mm/rev" class="DigNum (strict)"() -> ("Value"=w1139:dbl)  [unwired: 2 in, 2 out]
        n572 = property on="X mm/rev" class="DigNum (strict)"() -> ("Value"=w1166:dbl)  [unwired: 2 in, 2 out]
        n573 = property on="Y mm/rev" class="DigNum (strict)"() -> ("Value"=w1152:dbl)  [unwired: 2 in, 2 out]
        n574 = Divide(x=w1114, y=w1113) -> (x/y=→"Z Scan Duration":dbl)
        n575 = Multiply(x=w1142, y=w1139) -> (x*y=w1134:dbl)
        n576 = Divide(x=w1113, y=w1137) -> (x/y=w1135:dbl)
        n577 = Divide(x=w1112, y=w1111) -> (x/y=→"R Scan Duration":dbl)
        n578 = Multiply(x=w1128, y=w1125) -> (x*y=w1120:dbl)
        n579 = Divide(x=w1111, y=w1123) -> (x/y=w1121:dbl)
        n580 = Divide(x=w1103, y=w1102) -> (x/y=→"X Scan Duration":dbl)
        n581 = Multiply(x=w1166, y=w1162) -> (x*y=w1160:dbl)
        n582 = Divide(x=w1102, y=w1164) -> (x/y=w1169:dbl)
        n583 = Divide(x=w1107, y=w1106) -> (x/y=→"Y Scan Duration":dbl)
        n584 = Multiply(x=w1155, y=w1152) -> (x*y=w1148:dbl)
        n585 = Divide(x=w1106, y=w1108) -> (x/y=w1149:dbl)
        n586 = Multiply(x=w1139, y=w1135) -> (x*y=w1133:dbl)
        n587 = Multiply(x=w1125, y=w1121) -> (x*y=w1119:dbl)
        n588 = Multiply(x=w1169, y=w1166) -> (x*y=w1161:dbl)
        n589 = Multiply(x=w1152, y=w1149) -> (x*y=w1147:dbl)
        n590 = property on="Z Scan length MV mm" class="DigNum (strict)"("Value"=w1134) -> ()  [unwired: 2 in, 2 out]
        n591 = property on="R Scan length MV deg" class="DigNum (strict)"("Value"=w1120) -> ()  [unwired: 2 in, 2 out]
        n592 = property on="X Scan length MV mm" class="DigNum (strict)"("Val(Sgnl)"=w1160) -> ()  [unwired: 2 in, 2 out]
        n593 = property on="Y Scan length MV mm" class="DigNum (strict)"("Value"=w1148) -> ()  [unwired: 2 in, 2 out]
        n594 = property on="Z Scan velocity MV mm/sec" class="DigNum (strict)"("Val(Sgnl)"=w1133) -> ()  [unwired: 2 in, 2 out]
        n595 = property on="X Scan velocity MV mm/sec" class="DigNum (strict)"("Value"=w1161) -> ()  [unwired: 2 in, 2 out]
        n596 = property on="Y Scan velocity MV mm/sec" class="DigNum (strict)"("Val(Sgnl)"=w1147) -> ()  [unwired: 2 in, 2 out]
        n597 = Absolute Value(x=w1119) -> (abs(x)=w1101:dbl)
        n598 = property on="R Scan Velocity SP deg/sec" class="DigNum (strict)"("Val(Sgnl)"=w1101) -> ()  [unwired: 2 in, 2 out]
      }
      event #4 {
        n599 = event-data() -> ()  [unwired: 1 in, 7 out]
        n600 = property on="Y Step SP" class="DigNum (strict)"() -> ("Maximum"=w1184:dbl)  [unwired: 2 in, 2 out]
        n601 = property on="Y Step SP" class="DigNum (strict)"() -> ("Minimum"=w1183:dbl)  [unwired: 2 in, 2 out]
        n602 = property on="Y steps/rev" class="DigNum (strict)"() -> ("Value"=w1190:u32)  [unwired: 2 in, 2 out]
        n603 = property on="Y offset mm" class="DigNum (strict)"() -> ("Value"=w1188:dbl)  [unwired: 2 in, 2 out]
        n604 = property on="Y Velocity SP step/sec" class="DigNum (strict)"() -> ("Maximum"=w1177:dbl)  [unwired: 2 in, 2 out]
        n605 = property on="Y Velocity SP step/sec" class="DigNum (strict)"() -> ("Minimum"=w1176:dbl)  [unwired: 2 in, 2 out]
        n606 = property on="Y Position SP mm" class="DigNum (strict)"() -> ("Value"=w1187:dbl)  [unwired: 2 in, 2 out]
        n607 = property on="Y mm/rev" class="DigNum (strict)"() -> ("Value"=w1174:dbl)  [unwired: 2 in, 2 out]
        n608 = property on="Y Velocity SP mm/sec" class="DigNum (strict)"() -> ("Value"=w1181:dbl)  [unwired: 2 in, 2 out]
        n609 = Subtract(x=w1187, y=w1188) -> (x-y=w1191:dbl)
        n610 = Divide(x=w1181, y=w1174) -> (x/y=w1182:dbl)
        n611 = To Double Precision Float(number=w1190) -> (double precision float=w1175:dbl)
        n612 = Divide(x=w1191, y=w1174) -> (x/y=w1192:dbl)
        n613 = Multiply(x=w1182, y=w1175) -> (x*y=w1179:dbl)
        n614 = Multiply(x=w1192, y=w1175) -> (x*y=w1186:dbl)
        n615 = In Range and Coerce(upper limit=w1177, x=w1179, lower limit=w1176) -> (coerced(x)=w1178:dbl)  [unwired: 1 out]
        n616 = To Long Integer(number=w1178) -> (32bit integer=w1180:i32)
        n617 = In Range and Coerce(upper limit=w1184, x=w1186, lower limit=w1183) -> (coerced(x)=w1185:dbl)  [unwired: 1 out]
        n618 = To Long Integer(number=w1185) -> (32bit integer=w1189:i32)
        n619 = property on="Y Velocity SP step/sec" class="DigNum (strict)"("Val(Sgnl)"=w1180) -> ()  [unwired: 2 in, 2 out]
        n620 = property on="Y Step SP" class="DigNum (strict)"("Val(Sgnl)"=w1189) -> ()  [unwired: 2 in, 2 out]
      }
      event #5 {
        n621 = event-data() -> ()  [unwired: 1 in, 7 out]
        n622 = property on="X Step SP" class="DigNum (strict)"() -> ("Maximum"=w1203:dbl)  [unwired: 2 in, 2 out]
        n623 = property on="X Step SP" class="DigNum (strict)"() -> ("Minimum"=w1202:dbl)  [unwired: 2 in, 2 out]
        n624 = property on="X steps/rev" class="DigNum (strict)"() -> ("Value"=w1209:u32)  [unwired: 2 in, 2 out]
        n625 = property on="X offset mm" class="DigNum (strict)"() -> ("Value"=w1207:dbl)  [unwired: 2 in, 2 out]
        n626 = property on="X Velocity SP step/sec" class="DigNum (strict)"() -> ("Maximum"=w1196:dbl)  [unwired: 2 in, 2 out]
        n627 = property on="X Velocity SP step/sec" class="DigNum (strict)"() -> ("Minimum"=w1195:dbl)  [unwired: 2 in, 2 out]
        n628 = property on="X Position SP mm" class="DigNum (strict)"() -> ("Value"=w1206:dbl)  [unwired: 2 in, 2 out]
        n629 = property on="X mm/rev" class="DigNum (strict)"() -> ("Value"=w1193:dbl)  [unwired: 2 in, 2 out]
        n630 = property on="X Velocity SP mm/sec" class="DigNum (strict)"() -> ("Value"=w1200:dbl)  [unwired: 2 in, 2 out]
        n631 = Subtract(x=w1206, y=w1207) -> (x-y=w1210:dbl)
        n632 = Divide(x=w1200, y=w1193) -> (x/y=w1201:dbl)
        n633 = To Double Precision Float(number=w1209) -> (double precision float=w1194:dbl)
        n634 = Divide(x=w1210, y=w1193) -> (x/y=w1211:dbl)
        n635 = Multiply(x=w1201, y=w1194) -> (x*y=w1198:dbl)
        n636 = Multiply(x=w1211, y=w1194) -> (x*y=w1205:dbl)
        n637 = In Range and Coerce(upper limit=w1196, x=w1198, lower limit=w1195) -> (coerced(x)=w1197:dbl)  [unwired: 1 out]
        n638 = To Long Integer(number=w1197) -> (32bit integer=w1199:i32)
        n639 = In Range and Coerce(upper limit=w1203, x=w1205, lower limit=w1202) -> (coerced(x)=w1204:dbl)  [unwired: 1 out]
        n640 = To Long Integer(number=w1204) -> (32bit integer=w1208:i32)
        n641 = property on="X Velocity SP step/sec" class="DigNum (strict)"("Val(Sgnl)"=w1199) -> ()  [unwired: 2 in, 2 out]
        n642 = property on="X Step SP" class="DigNum (strict)"("Val(Sgnl)"=w1208) -> ()  [unwired: 2 in, 2 out]
      }
      event #6 {
        n643 = event-data() -> ()  [unwired: 1 in, 7 out]
        n644 = property on="Z Step SP" class="DigNum (strict)"() -> ("Maximum"=w1220:dbl)  [unwired: 2 in, 2 out]
        n645 = property on="Z Step SP" class="DigNum (strict)"() -> ("Minimum"=w1219:dbl)  [unwired: 2 in, 2 out]
        n646 = property on="Z steps/rev" class="DigNum (strict)"() -> ("Value"=w1226:u32)  [unwired: 2 in, 2 out]
        n647 = property on="Z offset mm" class="DigNum (strict)"() -> ("Value"=w1224:dbl)  [unwired: 2 in, 2 out]
        n648 = property on="Z Velocity SP step/sec" class="DigNum (strict)"() -> ("Maximum"=w1213:dbl)  [unwired: 2 in, 2 out]
        n649 = property on="Z Velocity SP step/sec" class="DigNum (strict)"() -> ("Minimum"=w1212:dbl)  [unwired: 2 in, 2 out]
        n650 = property on="Z Position SP mm" class="DigNum (strict)"() -> ("Value"=w1223:dbl)  [unwired: 2 in, 2 out]
        n651 = property on="Z mm/rev" class="DigNum (strict)"() -> ("Value"=w1229:dbl)  [unwired: 2 in, 2 out]
        n652 = property on="Z Velocity SP mm/sec" class="DigNum (strict)"() -> ("Value"=w1217:dbl)  [unwired: 2 in, 2 out]
        n653 = Subtract(x=w1223, y=w1224) -> (x-y=w1227:dbl)
        n654 = Divide(x=w1217, y=w1229) -> (x/y=w1218:dbl)
        n655 = To Double Precision Float(number=w1226) -> (double precision float=w1230:dbl)
        n656 = Divide(x=w1227, y=w1229) -> (x/y=w1228:dbl)
        n657 = Multiply(x=w1218, y=w1230) -> (x*y=w1215:dbl)
        n658 = Multiply(x=w1228, y=w1230) -> (x*y=w1222:dbl)
        n659 = In Range and Coerce(upper limit=w1213, x=w1215, lower limit=w1212) -> (coerced(x)=w1214:dbl)  [unwired: 1 out]
        n660 = To Long Integer(number=w1214) -> (32bit integer=w1216:i32)
        n661 = In Range and Coerce(upper limit=w1220, x=w1222, lower limit=w1219) -> (coerced(x)=w1221:dbl)  [unwired: 1 out]
        n662 = To Long Integer(number=w1221) -> (32bit integer=w1225:i32)
        n663 = property on="Z Velocity SP step/sec" class="DigNum (strict)"("Val(Sgnl)"=w1216) -> ()  [unwired: 2 in, 2 out]
        n664 = property on="Z Step SP" class="DigNum (strict)"("Val(Sgnl)"=w1225) -> ()  [unwired: 2 in, 2 out]
      }
      event #7 {
        n665 = event-data() -> ()  [unwired: 1 in, 7 out]
        n666 = property on="R Step SP" class="DigNum (strict)"() -> ("Maximum"=w1242:dbl)  [unwired: 2 in, 2 out]
        n667 = property on="R Step SP" class="DigNum (strict)"() -> ("Minimum"=w1241:dbl)  [unwired: 2 in, 2 out]
        n668 = property on="R steps/rev" class="DigNum (strict)"() -> ("Value"=w1248:u32)  [unwired: 2 in, 2 out]
        n669 = property on="R offset deg" class="DigNum (strict)"() -> ("Value"=w1246:dbl)  [unwired: 2 in, 2 out]
        n670 = property on="R Velocity SP step/sec" class="DigNum (strict)"() -> ("Maximum"=w1235:dbl)  [unwired: 2 in, 2 out]
        n671 = property on="R Velocity SP step/sec" class="DigNum (strict)"() -> ("Minimum"=w1234:dbl)  [unwired: 2 in, 2 out]
        n672 = property on="R Position SP deg" class="DigNum (strict)"() -> ("Value"=w1245:dbl)  [unwired: 2 in, 2 out]
        n673 = property on="R deg/rev" class="DigNum (strict)"() -> ("Value"=w1232:dbl)  [unwired: 2 in, 2 out]
        n674 = property on="R Velocity SP deg/sec" class="DigNum (strict)"() -> ("Value"=w1239:dbl)  [unwired: 2 in, 2 out]
        n675 = Subtract(x=w1245, y=w1246) -> (x-y=w1249:dbl)
        n676 = Divide(x=w1239, y=w1232) -> (x/y=w1240:dbl)
        n677 = To Double Precision Float(number=w1248) -> (double precision float=w1233:dbl)
        n678 = Divide(x=w1249, y=w1232) -> (x/y=w1250:dbl)
        n679 = Multiply(x=w1240, y=w1233) -> (x*y=w1237:dbl)
        n680 = Multiply(x=w1250, y=w1233) -> (x*y=w1244:dbl)
        n681 = Absolute Value(x=w1237) -> (abs(x)=w1231:dbl)
        n682 = In Range and Coerce(upper limit=w1242, x=w1244, lower limit=w1241) -> (coerced(x)=w1243:dbl)  [unwired: 1 out]
        n683 = In Range and Coerce(upper limit=w1235, x=w1231, lower limit=w1234) -> (coerced(x)=w1236:dbl)  [unwired: 1 out]
        n684 = To Long Integer(number=w1243) -> (32bit integer=w1247:i32)
        n685 = To Long Integer(number=w1236) -> (32bit integer=w1238:i32)
        n686 = property on="R Step SP" class="DigNum (strict)"("Val(Sgnl)"=w1247) -> ()  [unwired: 2 in, 2 out]
        n687 = property on="R Velocity SP step/sec" class="DigNum (strict)"("Val(Sgnl)"=w1238) -> ()  [unwired: 2 in, 2 out]
      }
      event #8 {
        n688 = event-data() -> ()  [unwired: 1 in, 7 out]
        n689 = property on="Y Step SP" class="DigNum (strict)"() -> ("Maximum"=w1260:dbl)  [unwired: 2 in, 2 out]
        n690 = property on="Y Step SP" class="DigNum (strict)"() -> ("Minimum"=w1261:dbl)  [unwired: 2 in, 2 out]
        n691 = property on="Y steps/rev" class="DigNum (strict)"() -> ("Value"=w1266:u32)  [unwired: 2 in, 2 out]
        n692 = property on="Y Scan Length SP mm" class="DigNum (strict)"() -> ("Value"=w1264:dbl)  [unwired: 2 in, 2 out]
        n693 = property on="Y mm/rev" class="DigNum (strict)"() -> ("Value"=w1251:dbl)  [unwired: 2 in, 2 out]
        n694 = property on="Y Scan Velocity SP steps/sec" class="DigNum (strict)"() -> ("Maximum"=w1254:dbl)  [unwired: 2 in, 2 out]
        n695 = property on="Y Scan Velocity SP steps/sec" class="DigNum (strict)"() -> ("Minimum"=w1253:dbl)  [unwired: 2 in, 2 out]
        n696 = property on="Y Scan Velocity SP mm/sec" class="DigNum (strict)"() -> ("Value"=w1258:dbl)  [unwired: 2 in, 2 out]
        n697 = Divide(x=w1264, y=w1251) -> (x/y=w1267:dbl)
        n698 = To Double Precision Float(number=w1266) -> (double precision float=w1252:dbl)
        n699 = Multiply(x=w1267, y=w1252) -> (x*y=w1263:dbl)
        n700 = Divide(x=w1258, y=w1251) -> (x/y=w1259:dbl)
        n701 = Multiply(x=w1259, y=w1252) -> (x*y=w1256:dbl)
        n702 = In Range and Coerce(upper limit=w1260, x=w1263, lower limit=w1261) -> (coerced(x)=w1262:dbl)  [unwired: 1 out]
        n703 = To Long Integer(number=w1262) -> (32bit integer=w1265:i32)
        n704 = In Range and Coerce(upper limit=w1254, x=w1256, lower limit=w1253) -> (coerced(x)=w1255:dbl)  [unwired: 1 out]
        n705 = To Long Integer(number=w1255) -> (32bit integer=w1257:i32)
        n706 = property on="Y Scan Length SP steps" class="DigNum (strict)"("Val(Sgnl)"=w1265) -> ()  [unwired: 2 in, 2 out]
        n707 = property on="Y Scan Velocity SP steps/sec" class="DigNum (strict)"("Val(Sgnl)"=w1257) -> ()  [unwired: 2 in, 2 out]
      }
      event #9 {
        n708 = event-data() -> ()  [unwired: 1 in, 7 out]
        n709 = property on="X Step SP" class="DigNum (strict)"() -> ("Maximum"=w1277:dbl)  [unwired: 2 in, 2 out]
        n710 = property on="X Step SP" class="DigNum (strict)"() -> ("Minimum"=w1278:dbl)  [unwired: 2 in, 2 out]
        n711 = property on="X steps/rev" class="DigNum (strict)"() -> ("Value"=w1283:u32)  [unwired: 2 in, 2 out]
        n712 = property on="X Scan Length SP mm" class="DigNum (strict)"() -> ("Value"=w1281:dbl)  [unwired: 2 in, 2 out]
        n713 = property on="X mm/rev" class="DigNum (strict)"() -> ("Value"=w1268:dbl)  [unwired: 2 in, 2 out]
        n714 = property on="X Scan Velocity SP steps/sec" class="DigNum (strict)"() -> ("Maximum"=w1271:dbl)  [unwired: 2 in, 2 out]
        n715 = property on="X Scan Velocity SP steps/sec" class="DigNum (strict)"() -> ("Minimum"=w1270:dbl)  [unwired: 2 in, 2 out]
        n716 = property on="X Scan Velocity SP mm/sec" class="DigNum (strict)"() -> ("Value"=w1275:dbl)  [unwired: 2 in, 2 out]
        n717 = Divide(x=w1281, y=w1268) -> (x/y=w1284:dbl)
        n718 = To Double Precision Float(number=w1283) -> (double precision float=w1269:dbl)
        n719 = Multiply(x=w1284, y=w1269) -> (x*y=w1280:dbl)
        n720 = Divide(x=w1275, y=w1268) -> (x/y=w1276:dbl)
        n721 = Multiply(x=w1276, y=w1269) -> (x*y=w1273:dbl)
        n722 = In Range and Coerce(upper limit=w1277, x=w1280, lower limit=w1278) -> (coerced(x)=w1279:dbl)  [unwired: 1 out]
        n723 = To Long Integer(number=w1279) -> (32bit integer=w1282:i32)
        n724 = In Range and Coerce(upper limit=w1271, x=w1273, lower limit=w1270) -> (coerced(x)=w1272:dbl)  [unwired: 1 out]
        n725 = To Long Integer(number=w1272) -> (32bit integer=w1274:i32)
        n726 = property on="X Scan Length SP steps" class="DigNum (strict)"("Val(Sgnl)"=w1282) -> ()  [unwired: 2 in, 2 out]
        n727 = property on="X Scan Velocity SP steps/sec" class="DigNum (strict)"("Val(Sgnl)"=w1274) -> ()  [unwired: 2 in, 2 out]
      }
      event #10 {
        n728 = event-data() -> ()  [unwired: 1 in, 7 out]
        n729 = property on="Z Step SP" class="DigNum (strict)"() -> ("Maximum"=w1294:dbl)  [unwired: 2 in, 2 out]
        n730 = property on="Z Step SP" class="DigNum (strict)"() -> ("Minimum"=w1295:dbl)  [unwired: 2 in, 2 out]
        n731 = property on="Z steps/rev" class="DigNum (strict)"() -> ("Value"=w1300:u32)  [unwired: 2 in, 2 out]
        n732 = property on="Z Scan Length SP mm" class="DigNum (strict)"() -> ("Value"=w1298:dbl)  [unwired: 2 in, 2 out]
        n733 = property on="Z mm/rev" class="DigNum (strict)"() -> ("Value"=w1285:dbl)  [unwired: 2 in, 2 out]
        n734 = property on="Z Scan Velocity SP steps/sec" class="DigNum (strict)"() -> ("Maximum"=w1288:dbl)  [unwired: 2 in, 2 out]
        n735 = property on="Z Scan Velocity SP steps/sec" class="DigNum (strict)"() -> ("Minimum"=w1287:dbl)  [unwired: 2 in, 2 out]
        n736 = property on="Z Scan Velocity SP mm/sec" class="DigNum (strict)"() -> ("Value"=w1292:dbl)  [unwired: 2 in, 2 out]
        n737 = Divide(x=w1298, y=w1285) -> (x/y=w1301:dbl)
        n738 = To Double Precision Float(number=w1300) -> (double precision float=w1286:dbl)
        n739 = Multiply(x=w1301, y=w1286) -> (x*y=w1297:dbl)
        n740 = Divide(x=w1292, y=w1285) -> (x/y=w1293:dbl)
        n741 = Multiply(x=w1293, y=w1286) -> (x*y=w1290:dbl)
        n742 = In Range and Coerce(upper limit=w1294, x=w1297, lower limit=w1295) -> (coerced(x)=w1296:dbl)  [unwired: 1 out]
        n743 = To Long Integer(number=w1296) -> (32bit integer=w1299:i32)
        n744 = In Range and Coerce(upper limit=w1288, x=w1290, lower limit=w1287) -> (coerced(x)=w1289:dbl)  [unwired: 1 out]
        n745 = To Long Integer(number=w1289) -> (32bit integer=w1291:i32)
        n746 = property on="Z Scan Length SP steps" class="DigNum (strict)"("Val(Sgnl)"=w1299) -> ()  [unwired: 2 in, 2 out]
        n747 = property on="Z Scan Velocity SP steps/sec" class="DigNum (strict)"("Val(Sgnl)"=w1291) -> ()  [unwired: 2 in, 2 out]
      }
      event #11 {
        n748 = event-data() -> ()  [unwired: 1 in, 7 out]
        n749 = property on="R Step SP" class="DigNum (strict)"() -> ("Maximum"=w1312:dbl)  [unwired: 2 in, 2 out]
        n750 = property on="R Step SP" class="DigNum (strict)"() -> ("Minimum"=w1313:dbl)  [unwired: 2 in, 2 out]
        n751 = property on="R steps/rev" class="DigNum (strict)"() -> ("Value"=w1318:u32)  [unwired: 2 in, 2 out]
        n752 = property on="R Velocity SP step/sec" class="DigNum (strict)"() -> ("Maximum"=w1306:dbl)  [unwired: 2 in, 2 out]
        n753 = property on="R Scan Length SP deg" class="DigNum (strict)"() -> ("Value"=w1316:dbl)  [unwired: 2 in, 2 out]
        n754 = property on="R deg/rev" class="DigNum (strict)"() -> ("Value"=w1303:dbl)  [unwired: 2 in, 2 out]
        n755 = property on="R Scan Velocity SP steps/sec" class="DigNum (strict)"() -> ("Minimum"=w1305:dbl)  [unwired: 2 in, 2 out]
        n756 = property on="R Scan Velocity SP deg/sec" class="DigNum (strict)"() -> ("Value"=w1310:dbl)  [unwired: 2 in, 2 out]
        n757 = Divide(x=w1316, y=w1303) -> (x/y=w1319:dbl)
        n758 = To Double Precision Float(number=w1318) -> (double precision float=w1304:dbl)
        n759 = Multiply(x=w1319, y=w1304) -> (x*y=w1315:dbl)
        n760 = Divide(x=w1310, y=w1303) -> (x/y=w1311:dbl)
        n761 = Multiply(x=w1311, y=w1304) -> (x*y=w1308:dbl)
        n762 = In Range and Coerce(upper limit=w1312, x=w1315, lower limit=w1313) -> (coerced(x)=w1314:dbl)  [unwired: 1 out]
        n763 = To Long Integer(number=w1314) -> (32bit integer=w1317:i32)
        n764 = Absolute Value(x=w1308) -> (abs(x)=w1302:dbl)
        n765 = property on="R Scan Length SP steps" class="DigNum (strict)"("Val(Sgnl)"=w1317) -> ()  [unwired: 2 in, 2 out]
        n766 = In Range and Coerce(upper limit=w1306, x=w1302, lower limit=w1305) -> (coerced(x)=w1307:dbl)  [unwired: 1 out]
        n767 = To Long Integer(number=w1307) -> (32bit integer=w1309:i32)
        n768 = property on="R Scan Velocity SP steps/sec" class="DigNum (strict)"("Val(Sgnl)"=w1309) -> ()  [unwired: 2 in, 2 out]
      }
      event #12 {
        n769 = event-data() -> ()  [unwired: 1 in, 7 out]
        n770 = flat-sequence {
          tunnel: w1324 -> [w1334]
          tunnel: w1325 -> [w1335]
          tunnel: [w1335] -> w1321
          tunnel: [w1334] -> w1320
          tunnel: [w1338] -> w1323
          tunnel: [w1337] -> w1322
          tunnel: w1321 -> [w1340]
          tunnel: w1320 -> [w1339]
          tunnel: [w1358] -> w1327
          tunnel: [w1357] -> w1326
          tunnel: w1323 -> [w1356]
          tunnel: w1322 -> [w1355]
          tunnel: [w1365] -> w1329
          tunnel: [w1364] -> w1328
          tunnel: w1327 -> [w1363]
          tunnel: w1326 -> [w1362]
          tunnel: [w1371] -> w1330
          tunnel: [w1372] -> w1331
          tunnel: w1329 -> [w1372]
          tunnel: w1328 -> [w1370]
          frame #0 {
            n771 = property on="Scan Go" class="Bool"("DisabledEnum"=T1."Disabled and Grayed Out" ("Disabled")) -> ()  [unwired: 2 in, 2 out]
            n772 = property on="Y Go" class="Bool"("DisabledEnum"=T1."Disabled and Grayed Out" ("Disabled")) -> ()  [unwired: 2 in, 2 out]
          }
          frame #1 {
            n773 = property on="Y Step SP" class="DigNum (strict)"() -> ("Value"=w1348:i32)  [unwired: 2 in, 2 out]
            n774 = property on="Y Step PV" class="DigNum (strict)"() -> ("Value"=w1347:i32)  [unwired: 2 in, 2 out]
            n775 = property on="Y Backlash" class="DigNum (strict)"() -> ("Value"=w1336:i32)  [unwired: 2 in, 2 out]
            n776 = Subtract(x=w1348, y=w1347) -> (x-y=w1346:i32)
            n777 = Sign(1:w1336) -> (0:w1344:i32)
            n778 = Sign(1:w1346) -> (0:w1345:i32)
            n779 = Multiply(x=w1345, y=w1344) -> (x*y=w1343:i32)
            n780 = Equal?(x=w1343, y=1) -> (x = y?=w1341:bool)
            n781 = case shown="False" w1341 {
              tunnel: w1340 -> [w1351 w1353]
              tunnel: w1339 -> [w1350 w1352]
              tunnel: [w1350 w1352] -> w1338
              tunnel: [w1351 w1353] -> w1337
              frame #0 {
                n782 = property on="Y Backlash corr" class="Bool (strict)"("Val(Sgnl)"=FALSE ("Value (Signaling)")) -> ()  [unwired: 2 in, 2 out]
              }
              frame #1 {
                n783 = property on="Y Backlash corr" class="Bool (strict)"("Val(Sgnl)"=TRUE ("Value (Signaling)")) -> ()  [unwired: 2 in, 2 out]
              }
            }
          }
          frame #2 {
            # "Velocity Setting"
            n784 = property on="Y Velocity SP step/sec" class="DigNum (strict)"() -> ("Value"=w1359:i32)  [unwired: 2 in, 2 out]
            n785 = Number To Decimal String(number=w1359) -> (decimal integer string=w1360:string)  [unwired: 1 in]
            n786 = call "mDrive Send Command.vi"("error in (no error)"=w1356, "Extra"=w1360, "Command"=T2."Max Velocity", "VISA resource name"=w1355) -> ("error out"=w1357:errorcluster, "VISA resource name out"=w1358:refnum<visa-resource-name>)  [unwired: 3 in, 1 out]
          }
          frame #3 {
            # "Move to Abs Position"
            n787 = property on="Y Step SP" class="DigNum (strict)"() -> ("Value"=w1368:i32)  [unwired: 2 in, 2 out]
            n788 = Number To Decimal String(number=w1368) -> (decimal integer string=w1367:string)  [unwired: 1 in]
            n789 = call "mDrive Send Command.vi"("error in (no error)"=w1362, "Extra"=w1367, "Command"=T2."Move to Absolute Position", "VISA resource name"=w1363) -> ("error out"=w1364:errorcluster, "VISA resource name out"=w1365:refnum<visa-resource-name>)  [unwired: 3 in, 1 out]
          }
          frame #4 {
            n790 = call "Time Delay"("error in (no error)"=w1370, "Delay Time (s)"=0.1) -> ("error out"=w1371:errorcluster)  [unwired: 9 in]
          }
        }
      }
      event #13 {
        n791 = event-data() -> ()  [unwired: 1 in, 7 out]
        n792 = flat-sequence {
          tunnel: w1375 -> [w1387]
          tunnel: w1376 -> [w1388]
          tunnel: [w1388] -> w1378
          tunnel: [w1387] -> w1377
          tunnel: [w1391] -> w1380
          tunnel: [w1390] -> w1379
          tunnel: w1378 -> [w1393]
          tunnel: w1377 -> [w1392]
          tunnel: [w1411] -> w1382
          tunnel: [w1410] -> w1381
          tunnel: w1380 -> [w1409]
          tunnel: w1379 -> [w1408]
          tunnel: [w1418] -> w1384
          tunnel: [w1417] -> w1383
          tunnel: w1382 -> [w1416]
          tunnel: w1381 -> [w1415]
          tunnel: [w1424] -> w1374
          tunnel: [w1425] -> w1373
          tunnel: w1384 -> [w1425]
          tunnel: w1383 -> [w1423]
          frame #0 {
            n793 = property on="Scan Go" class="Bool"("DisabledEnum"=T1."Disabled and Grayed Out" ("Disabled")) -> ()  [unwired: 2 in, 2 out]
            n794 = property on="Z Go" class="Bool"("DisabledEnum"=T1."Disabled and Grayed Out" ("Disabled")) -> ()  [unwired: 2 in, 2 out]
          }
          frame #1 {
            n795 = property on="Z Step SP" class="DigNum (strict)"() -> ("Value"=w1401:i32)  [unwired: 2 in, 2 out]
            n796 = property on="Z Step PV" class="DigNum (strict)"() -> ("Value"=w1400:i32)  [unwired: 2 in, 2 out]
            n797 = property on="Z Backlash" class="DigNum (strict)"() -> ("Value"=w1389:i32)  [unwired: 2 in, 2 out]
            n798 = Subtract(x=w1401, y=w1400) -> (x-y=w1399:i32)
            n799 = Sign(1:w1389) -> (0:w1397:i32)
            n800 = Sign(1:w1399) -> (0:w1398:i32)
            n801 = Multiply(x=w1398, y=w1397) -> (x*y=w1396:i32)
            n802 = Equal?(x=w1396, y=1) -> (x = y?=w1394:bool)
            n803 = case shown="True" w1394 {
              tunnel: w1393 -> [w1404 w1406]
              tunnel: w1392 -> [w1403 w1405]
              tunnel: [w1403 w1405] -> w1391
              tunnel: [w1404 w1406] -> w1390
              frame #0 {
                n804 = property on="Z Backlash corr" class="Bool (strict)"("Val(Sgnl)"=FALSE ("Value (Signaling)")) -> ()  [unwired: 2 in, 2 out]
              }
              frame #1 {
                n805 = property on="Z Backlash corr" class="Bool (strict)"("Val(Sgnl)"=TRUE ("Value (Signaling)")) -> ()  [unwired: 2 in, 2 out]
              }
            }
          }
          frame #2 {
            # "Velocity Setting"
            n806 = property on="Z Velocity SP step/sec" class="DigNum (strict)"() -> ("Value"=w1412:i32)  [unwired: 2 in, 2 out]
            n807 = Number To Decimal String(number=w1412) -> (decimal integer string=w1413:string)  [unwired: 1 in]
            n808 = call "mDrive Send Command.vi"("error in (no error)"=w1409, "Extra"=w1413, "Command"=T2."Max Velocity", "VISA resource name"=w1408) -> ("error out"=w1410:errorcluster, "VISA resource name out"=w1411:refnum<visa-resource-name>)  [unwired: 3 in, 1 out]
          }
          frame #3 {
            # "Move to Abs Position"
            n809 = property on="Z Step SP" class="DigNum (strict)"() -> ("Value"=w1421:i32)  [unwired: 2 in, 2 out]
            n810 = Number To Decimal String(number=w1421) -> (decimal integer string=w1420:string)  [unwired: 1 in]
            n811 = call "mDrive Send Command.vi"("error in (no error)"=w1415, "Extra"=w1420, "Command"=T2."Move to Absolute Position", "VISA resource name"=w1416) -> ("error out"=w1417:errorcluster, "VISA resource name out"=w1418:refnum<visa-resource-name>)  [unwired: 3 in, 1 out]
          }
          frame #4 {
            n812 = call "Time Delay28"("error in (no error)"=w1423, "Delay Time (s)"=0.1) -> ("error out"=w1424:errorcluster)  [unwired: 9 in]
          }
        }
      }
      event #14 {
        n813 = event-data() -> ()  [unwired: 1 in, 7 out]
        n814 = flat-sequence {
          tunnel: w1428 -> [w1440]
          tunnel: w1429 -> [w1441]
          tunnel: [w1441] -> w1431
          tunnel: [w1440] -> w1430
          tunnel: [w1444] -> w1433
          tunnel: [w1443] -> w1432
          tunnel: w1431 -> [w1446]
          tunnel: w1430 -> [w1445]
          tunnel: [w1464] -> w1435
          tunnel: [w1463] -> w1434
          tunnel: w1433 -> [w1462]
          tunnel: w1432 -> [w1461]
          tunnel: [w1471] -> w1437
          tunnel: [w1470] -> w1436
          tunnel: w1435 -> [w1469]
          tunnel: w1434 -> [w1468]
          tunnel: [w1477] -> w1427
          tunnel: [w1478] -> w1426
          tunnel: w1437 -> [w1478]
          tunnel: w1436 -> [w1476]
          frame #0 {
            n815 = property on="Scan Go" class="Bool"("DisabledEnum"=T1."Disabled and Grayed Out" ("Disabled")) -> ()  [unwired: 2 in, 2 out]
            n816 = property on="R Go" class="Bool"("DisabledEnum"=T1."Disabled and Grayed Out" ("Disabled")) -> ()  [unwired: 2 in, 2 out]
          }
          frame #1 {
            n817 = property on="R Step SP" class="DigNum (strict)"() -> ("Value"=w1454:i32)  [unwired: 2 in, 2 out]
            n818 = property on="R Step PV" class="DigNum (strict)"() -> ("Value"=w1453:i32)  [unwired: 2 in, 2 out]
            n819 = property on="R Backlash" class="DigNum (strict)"() -> ("Value"=w1442:i32)  [unwired: 2 in, 2 out]
            n820 = Subtract(x=w1454, y=w1453) -> (x-y=w1452:i32)
            n821 = Sign(1:w1442) -> (0:w1450:i32)
            n822 = Sign(1:w1452) -> (0:w1451:i32)
            n823 = Multiply(x=w1451, y=w1450) -> (x*y=w1449:i32)
            n824 = Equal?(x=w1449, y=1) -> (x = y?=w1447:bool)
            n825 = case shown="True" w1447 {
              tunnel: w1446 -> [w1457 w1459]
              tunnel: w1445 -> [w1456 w1458]
              tunnel: [w1456 w1458] -> w1444
              tunnel: [w1457 w1459] -> w1443
              frame #0 {
                n826 = property on="R Backlash corr" class="Bool (strict)"("Val(Sgnl)"=FALSE ("Value (Signaling)")) -> ()  [unwired: 2 in, 2 out]
              }
              frame #1 {
                n827 = property on="R Backlash corr" class="Bool (strict)"("Val(Sgnl)"=TRUE ("Value (Signaling)")) -> ()  [unwired: 2 in, 2 out]
              }
            }
          }
          frame #2 {
            # "Velocity Setting"
            n828 = property on="R Velocity SP step/sec" class="DigNum (strict)"() -> ("Value"=w1465:i32)  [unwired: 2 in, 2 out]
            n829 = Number To Decimal String(number=w1465) -> (decimal integer string=w1466:string)  [unwired: 1 in]
            n830 = call "mDrive Send Command.vi"("error in (no error)"=w1462, "Extra"=w1466, "Command"=T2."Max Velocity", "VISA resource name"=w1461) -> ("error out"=w1463:errorcluster, "VISA resource name out"=w1464:refnum<visa-resource-name>)  [unwired: 3 in, 1 out]
          }
          frame #3 {
            # "Move to Abs Position"
            n831 = property on="R Step SP" class="DigNum (strict)"() -> ("Value"=w1474:i32)  [unwired: 2 in, 2 out]
            n832 = Number To Decimal String(number=w1474) -> (decimal integer string=w1473:string)  [unwired: 1 in]
            n833 = call "mDrive Send Command.vi"("error in (no error)"=w1468, "Extra"=w1473, "Command"=T2."Move to Absolute Position", "VISA resource name"=w1469) -> ("error out"=w1470:errorcluster, "VISA resource name out"=w1471:refnum<visa-resource-name>)  [unwired: 3 in, 1 out]
          }
          frame #4 {
            n834 = call "Time Delay29"("error in (no error)"=w1476, "Delay Time (s)"=0.1) -> ("error out"=w1477:errorcluster)  [unwired: 9 in]
          }
        }
      }
      event #15 {
        n835 = event-data() -> ()  [unwired: 1 in, 7 out]
        n836 = flat-sequence {
          tunnel: [w1492] -> w1484
          tunnel: [w1491] -> w1483
          tunnel: w1482 -> [w1492]
          tunnel: w1481 -> [w1491]
          tunnel: [w1497] -> w1486
          tunnel: [w1496] -> w1485
          tunnel: w1484 -> [w1499]
          tunnel: w1483 -> [w1498]
          tunnel: [w1517] -> w1488
          tunnel: [w1516] -> w1487
          tunnel: w1486 -> [w1515]
          tunnel: w1485 -> [w1514]
          tunnel: [w1524] -> w1490
          tunnel: [w1523] -> w1489
          tunnel: w1488 -> [w1522]
          tunnel: w1487 -> [w1521]
          tunnel: [w1530] -> w1479
          tunnel: [w1531] -> w1480
          tunnel: w1490 -> [w1531]
          tunnel: w1489 -> [w1529]
          frame #0 {
            n837 = property on="Scan Go" class="Bool"("DisabledEnum"=T1."Disabled and Grayed Out" ("Disabled")) -> ()  [unwired: 2 in, 2 out]
            n838 = property on="X Go" class="Bool"("DisabledEnum"=T1."Disabled and Grayed Out" ("Disabled")) -> ()  [unwired: 2 in, 2 out]
          }
          frame #1 {
            n839 = property on="X Step SP" class="DigNum (strict)"() -> ("Value"=w1507:i32)  [unwired: 2 in, 2 out]
            n840 = property on="X Step PV" class="DigNum (strict)"() -> ("Value"=w1506:i32)  [unwired: 2 in, 2 out]
            n841 = property on="X Backlash" class="DigNum (strict)"() -> ("Value"=w1495:i32)  [unwired: 2 in, 2 out]
            n842 = Subtract(x=w1507, y=w1506) -> (x-y=w1505:i32)
            n843 = Sign(1:w1495) -> (0:w1503:i32)
            n844 = Sign(1:w1505) -> (0:w1504:i32)
            n845 = Multiply(x=w1504, y=w1503) -> (x*y=w1502:i32)
            n846 = Equal?(x=w1502, y=1) -> (x = y?=w1500:bool)
            n847 = case shown="True" w1500 {
              tunnel: w1499 -> [w1510 w1512]
              tunnel: w1498 -> [w1509 w1511]
              tunnel: [w1509 w1511] -> w1497
              tunnel: [w1510 w1512] -> w1496
              frame #0 {
                n848 = property on="X Backlash corr" class="Bool (strict)"("Val(Sgnl)"=FALSE ("Value (Signaling)")) -> ()  [unwired: 2 in, 2 out]
              }
              frame #1 {
                n849 = property on="X Backlash corr" class="Bool (strict)"("Val(Sgnl)"=TRUE ("Value (Signaling)")) -> ()  [unwired: 2 in, 2 out]
              }
            }
          }
          frame #2 {
            # "Velocity Setting"
            n850 = property on="X Velocity SP step/sec" class="DigNum (strict)"() -> ("Value"=w1518:i32)  [unwired: 2 in, 2 out]
            n851 = Number To Decimal String(number=w1518) -> (decimal integer string=w1519:string)  [unwired: 1 in]
            n852 = call "mDrive Send Command.vi"("error in (no error)"=w1515, "Extra"=w1519, "Command"=T2."Max Velocity", "VISA resource name"=w1514) -> ("error out"=w1516:errorcluster, "VISA resource name out"=w1517:refnum<visa-resource-name>)  [unwired: 3 in, 1 out]
          }
          frame #3 {
            # "Move to Abs Position"
            n853 = property on="X Step SP" class="DigNum (strict)"() -> ("Value"=w1527:i32)  [unwired: 2 in, 2 out]
            n854 = Number To Decimal String(number=w1527) -> (decimal integer string=w1526:string)  [unwired: 1 in]
            n855 = call "mDrive Send Command.vi"("error in (no error)"=w1521, "Extra"=w1526, "Command"=T2."Move to Absolute Position", "VISA resource name"=w1522) -> ("error out"=w1523:errorcluster, "VISA resource name out"=w1524:refnum<visa-resource-name>)  [unwired: 3 in, 1 out]
          }
          frame #4 {
            n856 = call "Time Delay15"("error in (no error)"=w1529, "Delay Time (s)"=0.1) -> ("error out"=w1530:errorcluster)  [unwired: 9 in]
          }
        }
      }
      event #16 {
        n857 = event-data() -> ()  [unwired: 1 in, 7 out]
        n858 = flat-sequence {
          tunnel: [w1547] -> w1539
          tunnel: [w1545] -> w1538
          tunnel: w1537 -> [w1541]
          tunnel: w1536 -> [w1540]
          tunnel: w1539 -> [w1562]
          tunnel: w1538 -> [w1561]
          tunnel: [w1562] -> w1533
          tunnel: [w1561] -> w1532
          tunnel: [w1564] -> w1534
          tunnel: [w1565] -> w1535
          tunnel: w1533 -> [w1565]
          tunnel: w1532 -> [w1564]
          frame #0 {
            # "VELOCITY"
            n859 = property on="X Scan Velocity SP steps/sec" class="DigNum (strict)"() -> ("Value"=w1548:i32)  [unwired: 2 in, 2 out]
            n860 = Number To Decimal String(number=w1548) -> (decimal integer string=w1549:string)  [unwired: 1 in]
            n861 = call "mDrive Send Command.vi"("error in (no error)"=w1540, "Extra"=w1549, "Command"=T2."Max Velocity", "VISA resource name"=w1541) -> ("error out"=w1550:errorcluster, "VISA resource name out"=w1555:refnum<visa-resource-name>)  [unwired: 3 in, 1 out]
            n862 = call "Time Delay9"("error in (no error)"=w1550) -> ("error out"=w1553:errorcluster)  [unwired: 10 in]
            n863 = call "mDrive Send Command.vi"("error in (no error)"=w1553, "Extra"="VM", "Command"=T2."Print Parameter", "VISA resource name"=w1555) -> ("error out"=w1546:errorcluster, "read buffer"=w1551:string, "VISA resource name out"=w1547:refnum<visa-resource-name>)  [unwired: 3 in]
            n864 = call "Time Delay10"("error in (no error)"=w1546) -> ("error out"=w1545:errorcluster)  [unwired: 10 in]
            n865 = Decimal String To Number(string=w1551, offset=0) -> (number=w1554:i32)  [unwired: 1 in, 1 out]
            n866 = property on="X velocity PV step/sec" class="DigNum (strict)"("Val(Sgnl)"=w1554) -> ()  [unwired: 2 in, 2 out]
          }
          frame #1 {
            n867 = property on="X Scan" class="Bool (strict)"("Val(Sgnl)"=TRUE ("Slew Ready 2")) -> ()  [unwired: 2 in, 2 out]
            n868 = property on="Scan Go" class="Bool"("DisabledEnum"=T1."Enabled" ("Disabled")) -> ()  [unwired: 2 in, 2 out]
            n869 = property on="Scan Cancel" class="Bool"("DisabledEnum"=T1."Enabled" ("Disabled")) -> ()  [unwired: 2 in, 2 out]
            n870 = property on="X Scan Length SP steps" class="DigNum (strict)"("DisabledEnum"=T1."Disabled and Grayed Out" ("Disabled")) -> ()  [unwired: 2 in, 2 out]
            n871 = property on="X Scan Velocity SP steps/sec" class="DigNum (strict)"("DisabledEnum"=T1."Disabled and Grayed Out" ("Disabled")) -> ()  [unwired: 2 in, 2 out]
          }
          frame #2 {
            n872 = property on="X Go" class="Bool"("DisabledEnum"=T1."Disabled and Grayed Out" ("Disabled")) -> ()  [unwired: 2 in, 2 out]
          }
        }
      }
      event #17 {
        n873 = event-data() -> ()  [unwired: 1 in, 7 out]
        n874 = flat-sequence {
          tunnel: w1573 -> [w1583]
          tunnel: w1572 -> [w1582]
          tunnel: [w1579] -> w1570
          tunnel: [w1577] -> w1569
          tunnel: w1570 -> [w1596]
          tunnel: w1569 -> [w1595]
          tunnel: [w1596] -> w1567
          tunnel: [w1595] -> w1566
          tunnel: [w1598] -> w1571
          tunnel: [w1599] -> w1568
          tunnel: w1567 -> [w1599]
          tunnel: w1566 -> [w1598]
          frame #0 {
            # "VELOCITY"
            n875 = property on="Y Scan Velocity SP steps/sec" class="DigNum (strict)"() -> ("Value"=w1580:i32)  [unwired: 2 in, 2 out]
            n876 = Number To Decimal String(number=w1580) -> (decimal integer string=w1581:string)  [unwired: 1 in]
            n877 = call "mDrive Send Command.vi"("error in (no error)"=w1583, "Extra"=w1581, "Command"=T2."Max Velocity", "VISA resource name"=w1582) -> ("error out"=w1584:errorcluster, "VISA resource name out"=w1589:refnum<visa-resource-name>)  [unwired: 3 in, 1 out]
            n878 = call "Time Delay5"("error in (no error)"=w1584) -> ("error out"=w1587:errorcluster)  [unwired: 10 in]
            n879 = call "mDrive Send Command.vi"("error in (no error)"=w1587, "Extra"="VM", "Command"=T2."Print Parameter", "VISA resource name"=w1589) -> ("error out"=w1578:errorcluster, "read buffer"=w1585:string, "VISA resource name out"=w1579:refnum<visa-resource-name>)  [unwired: 3 in]
            n880 = Decimal String To Number(string=w1585, offset=0) -> (number=w1588:i32)  [unwired: 1 in, 1 out]
            n881 = property on="Y velocity PV step/sec" class="DigNum (strict)"("Val(Sgnl)"=w1588) -> ()  [unwired: 2 in, 2 out]
            n882 = call "Time Delay6"("error in (no error)"=w1578) -> ("error out"=w1577:errorcluster)  [unwired: 10 in]
          }
          frame #1 {
            n883 = property on="Y Scan" class="Bool (strict)"("Val(Sgnl)"=TRUE ("Slew Ready 2")) -> ()  [unwired: 2 in, 2 out]
            n884 = property on="Scan Go" class="Bool"("DisabledEnum"=T1."Enabled" ("Disabled")) -> ()  [unwired: 2 in, 2 out]
            n885 = property on="Scan Cancel" class="Bool"("DisabledEnum"=T1."Enabled" ("Disabled")) -> ()  [unwired: 2 in, 2 out]
            n886 = property on="Y Scan Length SP steps" class="DigNum (strict)"("DisabledEnum"=T1."Disabled and Grayed Out" ("Disabled")) -> ()  [unwired: 2 in, 2 out]
            n887 = property on="Y Scan Velocity SP steps/sec" class="DigNum (strict)"("DisabledEnum"=T1."Disabled and Grayed Out" ("Disabled")) -> ()  [unwired: 2 in, 2 out]
          }
          frame #2 {
            n888 = property on="Y Go" class="Bool"("DisabledEnum"=T1."Disabled and Grayed Out" ("Disabled")) -> ()  [unwired: 2 in, 2 out]
          }
        }
      }
      event #18 {
        n889 = event-data() -> ()  [unwired: 1 in, 7 out]
        n890 = flat-sequence {
          tunnel: [w1615] -> w1607
          tunnel: [w1613] -> w1606
          tunnel: w1603 -> [w1609]
          tunnel: w1602 -> [w1608]
          tunnel: w1607 -> [w1630]
          tunnel: w1606 -> [w1629]
          tunnel: [w1630] -> w1605
          tunnel: [w1629] -> w1604
          tunnel: [w1632] -> w1601
          tunnel: [w1633] -> w1600
          tunnel: w1605 -> [w1633]
          tunnel: w1604 -> [w1632]
          frame #0 {
            # "VELOCITY"
            n891 = property on="Z Scan Velocity SP steps/sec" class="DigNum (strict)"() -> ("Value"=w1616:i32)  [unwired: 2 in, 2 out]
            n892 = Number To Decimal String(number=w1616) -> (decimal integer string=w1617:string)  [unwired: 1 in]
            n893 = call "mDrive Send Command.vi"("error in (no error)"=w1608, "Extra"=w1617, "Command"=T2."Max Velocity", "VISA resource name"=w1609) -> ("error out"=w1618:errorcluster, "VISA resource name out"=w1623:refnum<visa-resource-name>)  [unwired: 3 in, 1 out]
            n894 = call "Time Delay24"("error in (no error)"=w1618) -> ("error out"=w1621:errorcluster)  [unwired: 10 in]
            n895 = call "mDrive Send Command.vi"("error in (no error)"=w1621, "Extra"="VM", "Command"=T2."Print Parameter", "VISA resource name"=w1623) -> ("error out"=w1614:errorcluster, "read buffer"=w1619:string, "VISA resource name out"=w1615:refnum<visa-resource-name>)  [unwired: 3 in]
            n896 = Decimal String To Number(string=w1619, offset=0) -> (number=w1622:i32)  [unwired: 1 in, 1 out]
            n897 = property on="Z  velocity PV step/sec" class="DigNum (strict)"("Val(Sgnl)"=w1622) -> ()  [unwired: 2 in, 2 out]
            n898 = call "Time Delay25"("error in (no error)"=w1614) -> ("error out"=w1613:errorcluster)  [unwired: 10 in]
          }
          frame #1 {
            n899 = property on="Z Scan" class="Bool (strict)"("Val(Sgnl)"=TRUE ("Slew Ready 2")) -> ()  [unwired: 2 in, 2 out]
            n900 = property on="Scan Go" class="Bool"("DisabledEnum"=T1."Enabled" ("Disabled")) -> ()  [unwired: 2 in, 2 out]
            n901 = property on="Scan Cancel" class="Bool"("DisabledEnum"=T1."Enabled" ("Disabled")) -> ()  [unwired: 2 in, 2 out]
            n902 = property on="Z Scan Length SP steps" class="DigNum (strict)"("DisabledEnum"=T1."Disabled and Grayed Out" ("Disabled")) -> ()  [unwired: 2 in, 2 out]
            n903 = property on="Z Scan Velocity SP steps/sec" class="DigNum (strict)"("DisabledEnum"=T1."Disabled and Grayed Out" ("Disabled")) -> ()  [unwired: 2 in, 2 out]
          }
          frame #2 {
            n904 = property on="Z Go" class="Bool"("DisabledEnum"=T1."Disabled and Grayed Out" ("Disabled")) -> ()  [unwired: 2 in, 2 out]
          }
        }
      }
      event #19 {
        n905 = event-data() -> ()  [unwired: 1 in, 7 out]
        n906 = flat-sequence {
          tunnel: [w1649] -> w1641
          tunnel: [w1647] -> w1640
          tunnel: w1637 -> [w1643]
          tunnel: w1636 -> [w1642]
          tunnel: w1641 -> [w1664]
          tunnel: w1640 -> [w1663]
          tunnel: [w1664] -> w1639
          tunnel: [w1663] -> w1638
          tunnel: [w1666] -> w1634
          tunnel: [w1667] -> w1635
          tunnel: w1639 -> [w1667]
          tunnel: w1638 -> [w1666]
          frame #0 {
            # "VELOCITY"
            n907 = property on="R Scan Velocity SP steps/sec" class="DigNum (strict)"() -> ("Value"=w1650:i32)  [unwired: 2 in, 2 out]
            n908 = Number To Decimal String(number=w1650) -> (decimal integer string=w1651:string)  [unwired: 1 in]
            n909 = call "mDrive Send Command.vi"("error in (no error)"=w1642, "Extra"=w1651, "Command"=T2."Max Velocity", "VISA resource name"=w1643) -> ("error out"=w1652:errorcluster, "VISA resource name out"=w1657:refnum<visa-resource-name>)  [unwired: 3 in, 1 out]
            n910 = call "Time Delay26"("error in (no error)"=w1652) -> ("error out"=w1655:errorcluster)  [unwired: 10 in]
            n911 = call "mDrive Send Command.vi"("error in (no error)"=w1655, "Extra"="VM", "Command"=T2."Print Parameter", "VISA resource name"=w1657) -> ("error out"=w1648:errorcluster, "read buffer"=w1653:string, "VISA resource name out"=w1649:refnum<visa-resource-name>)  [unwired: 3 in]
            n912 = Decimal String To Number(string=w1653, offset=0) -> (number=w1656:i32)  [unwired: 1 in, 1 out]
            n913 = property on="R velocity PV step/sec" class="DigNum (strict)"("Val(Sgnl)"=w1656) -> ()  [unwired: 2 in, 2 out]
            n914 = call "Time Delay27"("error in (no error)"=w1648) -> ("error out"=w1647:errorcluster)  [unwired: 10 in]
          }
          frame #1 {
            n915 = property on="R Scan" class="Bool (strict)"("Val(Sgnl)"=TRUE ("Slew Ready 2")) -> ()  [unwired: 2 in, 2 out]
            n916 = property on="Scan Go" class="Bool"("DisabledEnum"=T1."Enabled" ("Disabled")) -> ()  [unwired: 2 in, 2 out]
            n917 = property on="Scan Cancel" class="Bool"("DisabledEnum"=T1."Enabled" ("Disabled")) -> ()  [unwired: 2 in, 2 out]
            n918 = property on="R Scan Length SP steps" class="DigNum (strict)"("DisabledEnum"=T1."Disabled and Grayed Out" ("Disabled")) -> ()  [unwired: 2 in, 2 out]
            n919 = property on="R Scan Velocity SP steps/sec" class="DigNum (strict)"("DisabledEnum"=T1."Disabled and Grayed Out" ("Disabled")) -> ()  [unwired: 2 in, 2 out]
          }
          frame #2 {
            n920 = property on="R Go" class="Bool"("DisabledEnum"=T1."Disabled and Grayed Out" ("Disabled")) -> ()  [unwired: 2 in, 2 out]
          }
        }
      }
      event #20 {
        n921 = event-data() -> ()  [unwired: 1 in, 4 out]
        n922 = event-data() -> ()  [unwired: 3 in, 1 out]
      }
      event #21 {
        n923 = event-data() -> ()  [unwired: 1 in, 7 out]
        n924 = flat-sequence {
          tunnel: [w1700] -> w1682
          tunnel: [w1699] -> w1681
          tunnel: w1680 -> [w1698]
          tunnel: w1679 -> [w1697]
          frame #0 {
            n925 = call "mDrive Send Command.vi"("error in (no error)"=w1697, "Command"=T2."Stop", "VISA resource name"=w1698) -> ("error out"=w1699:errorcluster, "VISA resource name out"=w1700:refnum<visa-resource-name>)  [unwired: 4 in, 1 out]
          }
        }
        n926 = flat-sequence {
          tunnel: w1686 -> [w1706]
          tunnel: w1685 -> [w1705]
          tunnel: [w1704] -> w1684
          tunnel: [w1703] -> w1683
          frame #0 {
            n927 = call "mDrive Send Command.vi"("error in (no error)"=w1705, "Command"=T2."Stop", "VISA resource name"=w1706) -> ("error out"=w1703:errorcluster, "VISA resource name out"=w1704:refnum<visa-resource-name>)  [unwired: 4 in, 1 out]
          }
        }
        n928 = flat-sequence {
          tunnel: [w1695] -> w1676
          tunnel: [w1694] -> w1675
          tunnel: w1678 -> [w1693]
          tunnel: w1677 -> [w1692]
          frame #0 {
            n929 = call "mDrive Send Command.vi"("error in (no error)"=w1692, "Command"=T2."Stop", "VISA resource name"=w1693) -> ("error out"=w1694:errorcluster, "VISA resource name out"=w1695:refnum<visa-resource-name>)  [unwired: 4 in, 1 out]
          }
        }
        n930 = flat-sequence {
          tunnel: w1674 -> [w1691]
          tunnel: w1673 -> [w1690]
          tunnel: [w1689] -> w1672
          tunnel: [w1687] -> _
          tunnel: [w1687] -> w1671
          frame #0 {
            n931 = call "mDrive Send Command.vi"("error in (no error)"=w1690, "Command"=T2."Stop", "VISA resource name"=w1691) -> ("error out"=w1687:errorcluster, "VISA resource name out"=w1689:refnum<visa-resource-name>)  [unwired: 4 in, 1 out]
          }
        }
      }
      event #22 {
        n932 = event-data() -> ()  [unwired: 1 in, 7 out]
        n933 = flat-sequence {
          tunnel: w1722 -> [w1761]
          tunnel: w1721 -> [w1760]
          tunnel: [w1763] -> w1724
          tunnel: [w1762] -> w1723
          tunnel: [w1770] -> w1719
          tunnel: [w1771] -> w1720
          tunnel: w1724 -> [w1771]
          tunnel: w1723 -> [w1770]
          frame #0 {
            n934 = call "mDrive Send Command.vi"("error in (no error)"=w1760, "Command"=T2."Stop", "VISA resource name"=w1761) -> ("error out"=w1762:errorcluster, "VISA resource name out"=w1763:refnum<visa-resource-name>)  [unwired: 4 in, 1 out]
          }
          frame #1 {
            n935 = property on="X Scan" class="Bool (strict)"("Value"=FALSE ("Slew Ready")) -> ()  [unwired: 2 in, 2 out]
            n936 = property on="X Scan set" class="Bool"("DisabledEnum"=T1."Enabled" ("Disabled")) -> ()  [unwired: 2 in, 2 out]
            n937 = property on="X Scan Velocity SP steps/sec" class="DigNum (strict)"("DisabledEnum"=T1."Enabled" ("Disabled")) -> ()  [unwired: 2 in, 2 out]
            n938 = property on="X Scan Length SP steps" class="DigNum (strict)"("DisabledEnum"=T1."Enabled" ("Disabled")) -> ()  [unwired: 2 in, 2 out]
            n939 = property on="X Go" class="Bool"("DisabledEnum"=T1."Enabled" ("Disabled")) -> ()  [unwired: 2 in, 2 out]
            n940 = property on="X Scan OK" class="Bool"("DisabledEnum"=T1."Enabled" ("Disabled")) -> ()  [unwired: 2 in, 2 out]
          }
        }
        n941 = flat-sequence {
          tunnel: w1730 -> [w1774]
          tunnel: w1729 -> [w1773]
          tunnel: [w1776] -> w1726
          tunnel: [w1775] -> w1725
          tunnel: [w1783] -> w1731
          tunnel: [w1784] -> w1732
          tunnel: w1726 -> [w1784]
          tunnel: w1725 -> [w1783]
          frame #0 {
            n942 = call "mDrive Send Command.vi"("error in (no error)"=w1773, "Command"=T2."Stop", "VISA resource name"=w1774) -> ("error out"=w1775:errorcluster, "VISA resource name out"=w1776:refnum<visa-resource-name>)  [unwired: 4 in, 1 out]
          }
          frame #1 {
            n943 = property on="Y Scan" class="Bool (strict)"("Value"=FALSE ("Slew Ready")) -> ()  [unwired: 2 in, 2 out]
            n944 = property on="Y Scan Velocity SP steps/sec" class="DigNum (strict)"("DisabledEnum"=T1."Enabled" ("Disabled")) -> ()  [unwired: 2 in, 2 out]
            n945 = property on="Y Go" class="Bool"("DisabledEnum"=T1."Enabled" ("Disabled")) -> ()  [unwired: 2 in, 2 out]
            n946 = property on="Y Scan OK" class="Bool"("DisabledEnum"=T1."Enabled" ("Disabled")) -> ()  [unwired: 2 in, 2 out]
            n947 = property on="Y Scan Length SP steps" class="DigNum (strict)"("DisabledEnum"=T1."Enabled" ("Disabled")) -> ()  [unwired: 2 in, 2 out]
            n948 = property on="Y Scan set" class="Bool"("DisabledEnum"=T1."Enabled" ("Disabled")) -> ()  [unwired: 2 in, 2 out]
          }
        }
        n949 = flat-sequence {
          tunnel: [w1750] -> w1718
          tunnel: [w1749] -> w1717
          tunnel: w1716 -> [w1747]
          tunnel: w1715 -> [w1746]
          tunnel: [w1757] -> w1713
          tunnel: [w1758] -> w1714
          tunnel: w1718 -> [w1758]
          tunnel: w1717 -> [w1757]
          frame #0 {
            n950 = call "mDrive Send Command.vi"("error in (no error)"=w1746, "Command"=T2."Stop", "VISA resource name"=w1747) -> ("error out"=w1749:errorcluster, "VISA resource name out"=w1750:refnum<visa-resource-name>)  [unwired: 4 in, 1 out]
          }
          frame #1 {
            n951 = property on="Z Scan" class="Bool (strict)"("Value"=FALSE ("Slew Ready")) -> ()  [unwired: 2 in, 2 out]
            n952 = property on="Z Scan set" class="Bool"("DisabledEnum"=T1."Enabled" ("Disabled")) -> ()  [unwired: 2 in, 2 out]
            n953 = property on="Z Scan Velocity SP steps/sec" class="DigNum (strict)"("DisabledEnum"=T1."Enabled" ("Disabled")) -> ()  [unwired: 2 in, 2 out]
            n954 = property on="Z Scan Length SP steps" class="DigNum (strict)"("DisabledEnum"=T1."Enabled" ("Disabled")) -> ()  [unwired: 2 in, 2 out]
            n955 = property on="Z Go" class="Bool"("DisabledEnum"=T1."Enabled" ("Disabled")) -> ()  [unwired: 2 in, 2 out]
            n956 = property on="Z Scan OK" class="Bool"("DisabledEnum"=T1."Enabled" ("Disabled")) -> ()  [unwired: 2 in, 2 out]
          }
        }
        n957 = flat-sequence {
          tunnel: [w1737] -> w1712
          tunnel: [w1736] -> w1711
          tunnel: w1710 -> [w1734]
          tunnel: w1709 -> [w1733]
          tunnel: [w1744] -> w1707
          tunnel: [w1745] -> w1708
          tunnel: w1712 -> [w1745]
          tunnel: w1711 -> [w1744]
          frame #0 {
            n958 = call "mDrive Send Command.vi"("error in (no error)"=w1733, "Command"=T2."Stop", "VISA resource name"=w1734) -> ("error out"=w1736:errorcluster, "VISA resource name out"=w1737:refnum<visa-resource-name>)  [unwired: 4 in, 1 out]
          }
          frame #1 {
            n959 = property on="R Scan" class="Bool (strict)"("Value"=FALSE ("Slew Ready")) -> ()  [unwired: 2 in, 2 out]
            n960 = property on="R Scan OK" class="Bool"("DisabledEnum"=T1."Enabled" ("Disabled")) -> ()  [unwired: 2 in, 2 out]
            n961 = property on="R Scan Length SP steps" class="DigNum (strict)"("DisabledEnum"=T1."Enabled" ("Disabled")) -> ()  [unwired: 2 in, 2 out]
            n962 = property on="R Scan set" class="Bool"("DisabledEnum"=T1."Enabled" ("Disabled")) -> ()  [unwired: 2 in, 2 out]
            n963 = property on="R Scan Velocity SP steps/sec" class="DigNum (strict)"("DisabledEnum"=T1."Enabled" ("Disabled")) -> ()  [unwired: 2 in, 2 out]
            n964 = property on="R Go" class="Bool"("DisabledEnum"=T1."Enabled" ("Disabled")) -> ()  [unwired: 2 in, 2 out]
          }
        }
        n965 = property on="Scan Go" class="Bool"("DisabledEnum"=T1."Disabled and Grayed Out" ("Disabled")) -> ()  [unwired: 2 in, 2 out]
        n966 = property on="Scan Cancel" class="Bool"("DisabledEnum"=T1."Disabled and Grayed Out" ("Disabled")) -> ()  [unwired: 2 in, 2 out]
      }
      event #23 {
        n967 = event-data() -> ()  [unwired: 1 in, 7 out]
        n968 = flat-sequence {
          tunnel: [w1864] -> w1848
          tunnel: [w1862] -> w1841
          tunnel: [w1863] -> w1838
          tunnel: [w1857] -> w1837
          tunnel: [w1861] -> w1836
          tunnel: [w1860] -> w1835
          tunnel: [w1859] -> w1834
          tunnel: [w1858] -> w1833
          tunnel: w1812 -> [w1856]
          tunnel: [w1856] -> w1811
          tunnel: w1810 -> [w1855]
          tunnel: [w1855] -> w1809
          tunnel: w1808 -> [w1854]
          tunnel: [w1854] -> w1807
          tunnel: w1806 -> [w1853]
          tunnel: [w1853] -> w1805
          tunnel: w1804 -> [w1852]
          tunnel: [w1852] -> w1803
          tunnel: w1802 -> [w1851]
          tunnel: [w1851] -> w1801
          tunnel: [w1850] -> w1800
          tunnel: w1799 -> [w1850]
          tunnel: [w1849] -> w1798
          tunnel: w1797 -> [w1849]
          tunnel: [w1916] -> w1845
          tunnel: [w1915] -> w1843
          tunnel: w1848 -> [w1914]
          tunnel: w1841 -> [w1913]
          tunnel: [w1913] -> w1839
          tunnel: w1838 -> [w1912]
          tunnel: w1837 -> [w1901]
          tunnel: w1836 -> [w1911]
          tunnel: w1835 -> [w1907]
          tunnel: w1834 -> [w1904]
          tunnel: w1833 -> [w1910]
          tunnel: [w1909] -> w1831
          tunnel: [w1908] -> w1829
          tunnel: [w1907] -> w1826
          tunnel: [w1906] -> w1824
          tunnel: [w1905] -> w1822
          tunnel: [w1904] -> w1820
          tunnel: [w1903] -> w1818
          tunnel: [w1902] -> w1816
          tunnel: [w1901] -> w1815
          tunnel: w1811 -> [w1900]
          tunnel: w1809 -> [w1899]
          tunnel: w1807 -> [w1898]
          tunnel: w1805 -> [w1897]
          tunnel: w1803 -> [w1896]
          tunnel: w1801 -> [w1895]
          tunnel: w1800 -> [w1894]
          tunnel: w1798 -> [w1893]
          tunnel: w1845 -> [w1957]
          tunnel: [w1957] -> w1844
          tunnel: w1843 -> [w1956]
          tunnel: [w1956] -> w1842
          tunnel: [w1954] -> w1840
          tunnel: w1839 -> [w1954]
          tunnel: [w1953] -> w1832
          tunnel: w1831 -> [w1953]
          tunnel: [w1952] -> w1830
          tunnel: w1829 -> [w1952]
          tunnel: [w1951] -> w1828
          tunnel: [w1950] -> w1827
          tunnel: w1826 -> [w1950]
          tunnel: [w1949] -> w1825
          tunnel: w1824 -> [w1949]
          tunnel: [w1948] -> w1823
          tunnel: w1822 -> [w1948]
          tunnel: [w1947] -> w1821
          tunnel: w1820 -> [w1947]
          tunnel: [w1946] -> w1819
          tunnel: w1818 -> [w1946]
          tunnel: [w1945] -> w1817
          tunnel: w1816 -> [w1945]
          tunnel: w1815 -> [w1951]
          tunnel: w1844 -> [w1977]
          tunnel: [w1975] -> w1847
          tunnel: w1842 -> [w1976]
          tunnel: [w1974] -> w1846
          tunnel: w1840 -> [w1973]
          tunnel: w1832 -> [w1972]
          tunnel: w1830 -> [w1971]
          tunnel: w1828 -> [w1970]
          tunnel: w1827 -> [w1969]
          tunnel: w1825 -> [w1968]
          tunnel: w1823 -> [w1967]
          tunnel: w1821 -> [w1966]
          tunnel: w1819 -> [w1965]
          tunnel: w1817 -> [w1964]
          tunnel: [w1963] -> w1814
          tunnel: [w1962] -> w1813
          tunnel: [w1961] -> w1792
          tunnel: [w1960] -> w1789
          tunnel: [w1959] -> w1787
          tunnel: [w1958] -> w1785
          tunnel: w1847 -> [w2035]
          tunnel: w1846 -> [w2034]
          tunnel: [w2035] -> w1796
          tunnel: [w2034] -> w1795
          tunnel: [w2028] -> w1794
          tunnel: w1814 -> [w2028]
          tunnel: [w2027] -> w1793
          tunnel: w1813 -> [w2027]
          tunnel: w1792 -> [w2017]
          tunnel: [w2017] -> w1791
          tunnel: [w2016] -> w1790
          tunnel: w1789 -> [w2016]
          tunnel: [w2015] -> w1788
          tunnel: w1787 -> [w2015]
          tunnel: [w2014] -> w1786
          tunnel: w1785 -> [w2014]
          frame #0 {
            n969 = property on="X Scan" class="Bool (strict)"() -> ("Value"=w1857:bool)  [unwired: 2 in, 2 out]
            n970 = property on="Y Scan" class="Bool (strict)"() -> ("Value"=w1862:bool)  [unwired: 2 in, 2 out]
            n971 = property on="Z Scan" class="Bool (strict)"() -> ("Value"=w1859:bool)  [unwired: 2 in, 2 out]
            n972 = property on="R Scan" class="Bool (strict)"() -> ("Value"=w1860:bool)  [unwired: 2 in, 2 out]
            n973 = case shown="True" w1857 {
              tunnel: ["" w1880] -> w1863
              frame #0 {
              }
              frame #1 {
                n974 = property on="X Scan Length SP steps" class="DigNum (strict)"() -> ("Value"=w1885:i32)  [unwired: 2 in, 2 out]
                n975 = Number To Decimal String(number=w1885) -> (decimal integer string=w1882:string)  [unwired: 1 in]
                n976 = call <vilib>:"Space Constant.vi"() -> ("String"=w1883:string)
                n977 = Concatenate Strings("MR", w1883, w1882, "\r") -> (w1880:string)
              }
            }
            n978 = case shown="True" w1862 {
              tunnel: ["" w1887] -> w1864
              frame #0 {
              }
              frame #1 {
                n979 = property on="Y Scan Length SP steps" class="DigNum (strict)"() -> ("Value"=w1892:i32)  [unwired: 2 in, 2 out]
                n980 = Number To Decimal String(number=w1892) -> (decimal integer string=w1889:string)  [unwired: 1 in]
                n981 = call <vilib>:"Space Constant.vi"() -> ("String"=w1890:string)
                n982 = Concatenate Strings("MR", w1890, w1889, "\r") -> (w1887:string)
              }
            }
            n983 = case shown="True" w1859 {
              tunnel: ["" w1873] -> w1861
              frame #0 {
              }
              frame #1 {
                n984 = property on="Z Scan Length SP steps" class="DigNum (strict)"() -> ("Value"=w1878:i32)  [unwired: 2 in, 2 out]
                n985 = Number To Decimal String(number=w1878) -> (decimal integer string=w1875:string)  [unwired: 1 in]
                n986 = call <vilib>:"Space Constant.vi"() -> ("String"=w1876:string)
                n987 = Concatenate Strings("MR", w1876, w1875, "\r") -> (w1873:string)
              }
            }
            n988 = case shown="True" w1860 {
              tunnel: ["" w1866] -> w1858
              frame #0 {
              }
              frame #1 {
                n989 = property on="R Scan Length SP steps" class="DigNum (strict)"() -> ("Value"=w1871:i32)  [unwired: 2 in, 2 out]
                n990 = Number To Decimal String(number=w1871) -> (decimal integer string=w1868:string)  [unwired: 1 in]
                n991 = call <vilib>:"Space Constant.vi"() -> ("String"=w1869:string)
                n992 = Concatenate Strings("MR", w1869, w1868, "\r") -> (w1866:string)
              }
            }
          }
          frame #1 {
            n993 = case shown="False" w1901 {
              tunnel: [w1932 w1937] -> w1909
              tunnel: [w1931 w1936] -> w1908
              tunnel: w1912 -> [_ w1935]
              tunnel: w1900 -> [w1932 w1934]
              tunnel: w1899 -> [w1931 w1933]
              frame #0 {
              }
              frame #1 {
                n994 = VISA Write(VISA resource name=w1934, write buffer=w1935, error in (no error)=w1933) -> (VISA resource name out=w1937:refnum<visa-resource-name>, error out=w1936:errorcluster)  [unwired: 1 out]
              }
            }
            n995 = case shown="False" w1913 {
              tunnel: [w1939 w1944] -> w1916
              tunnel: [w1938 w1943] -> w1915
              tunnel: w1914 -> [_ w1942]
              tunnel: w1898 -> [w1939 w1941]
              tunnel: w1897 -> [w1938 w1940]
              frame #0 {
              }
              frame #1 {
                n996 = VISA Write(VISA resource name=w1941, write buffer=w1942, error in (no error)=w1940) -> (VISA resource name out=w1944:refnum<visa-resource-name>, error out=w1943:errorcluster)  [unwired: 1 out]
              }
            }
            n997 = case shown="False" w1904 {
              tunnel: [w1925 w1930] -> w1903
              tunnel: [w1924 w1929] -> w1902
              tunnel: w1911 -> [_ w1928]
              tunnel: w1896 -> [w1925 w1927]
              tunnel: w1895 -> [w1924 w1926]
              frame #0 {
              }
              frame #1 {
                n998 = VISA Write(VISA resource name=w1927, write buffer=w1928, error in (no error)=w1926) -> (VISA resource name out=w1930:refnum<visa-resource-name>, error out=w1929:errorcluster)  [unwired: 1 out]
              }
            }
            n999 = case shown="False" w1907 {
              tunnel: [w1918 w1923] -> w1906
              tunnel: [w1917 w1922] -> w1905
              tunnel: w1910 -> [_ w1921]
              tunnel: w1894 -> [w1918 w1920]
              tunnel: w1893 -> [w1917 w1919]
              frame #0 {
              }
              frame #1 {
                n1000 = VISA Write(VISA resource name=w1920, write buffer=w1921, error in (no error)=w1919) -> (VISA resource name out=w1923:refnum<visa-resource-name>, error out=w1922:errorcluster)  [unwired: 1 out]
              }
            }
          }
          frame #2 {
            n1001 = call "Time Delay7"("Delay Time (s)"=0.1) -> ()  [unwired: 10 in, 1 out]
          }
          frame #3 {
            n1002 = case shown="True" w1970 {
              tunnel: w1972 -> [w1997 w2001]
              tunnel: w1971 -> [w1996 w2000]
              tunnel: [w1997 w1999] -> w1959
              tunnel: [w1996 w1998] -> w1958
              frame #0 {
              }
              frame #1 {
                n1003 = property class="Instr"(reference=w2001, error in=w2000) -> (reference out=w2003:refnum<visa-resource-name>, error out=w2002:errorcluster, "Serial Settings:Number of Bytes at Serial Port"=w2004:u32)
                n1004 = VISA Read(VISA resource name=w2003, byte count=w2004, error in (no error)=w2002) -> (VISA resource name out=w1999:refnum<visa-resource-name>, error out=w1998:errorcluster)  [unwired: 2 out]
              }
            }
            n1005 = case shown="True" w1973 {
              tunnel: w1977 -> [w2006 w2010]
              tunnel: w1976 -> [w2005 w2009]
              tunnel: [w2006 w2008] -> w1975
              tunnel: [w2005 w2007] -> w1974
              frame #0 {
              }
              frame #1 {
                n1006 = property class="Instr"(reference=w2010, error in=w2009) -> (reference out=w2012:refnum<visa-resource-name>, error out=w2011:errorcluster, "Serial Settings:Number of Bytes at Serial Port"=w2013:u32)
                n1007 = VISA Read(VISA resource name=w2012, byte count=w2013, error in (no error)=w2011) -> (VISA resource name out=w2008:refnum<visa-resource-name>, error out=w2007:errorcluster)  [unwired: 2 out]
              }
            }
            n1008 = case shown="True" w1966 {
              tunnel: w1965 -> [w1979 w1983]
              tunnel: w1964 -> [w1978 w1982]
              tunnel: [w1979 w1981] -> w1963
              tunnel: [w1978 w1980] -> w1962
              frame #0 {
              }
              frame #1 {
                n1009 = property class="Instr"(reference=w1983, error in=w1982) -> (reference out=w1985:refnum<visa-resource-name>, error out=w1984:errorcluster, "Serial Settings:Number of Bytes at Serial Port"=w1986:u32)
                n1010 = VISA Read(VISA resource name=w1985, byte count=w1986, error in (no error)=w1984) -> (VISA resource name out=w1981:refnum<visa-resource-name>, error out=w1980:errorcluster)  [unwired: 2 out]
              }
            }
            n1011 = case shown="True" w1969 {
              tunnel: w1968 -> [w1988 w1992]
              tunnel: w1967 -> [w1987 w1991]
              tunnel: [w1988 w1990] -> w1961
              tunnel: [w1987 w1989] -> w1960
              frame #0 {
              }
              frame #1 {
                n1012 = property class="Instr"(reference=w1992, error in=w1991) -> (reference out=w1994:refnum<visa-resource-name>, error out=w1993:errorcluster, "Serial Settings:Number of Bytes at Serial Port"=w1995:u32)
                n1013 = VISA Read(VISA resource name=w1994, byte count=w1995, error in (no error)=w1993) -> (VISA resource name out=w1990:refnum<visa-resource-name>, error out=w1989:errorcluster)  [unwired: 2 out]
              }
            }
          }
          frame #4 {
            n1014 = property on="X Scan" class="Bool (strict)"("Val(Sgnl)"=FALSE ("Slew Ready 2")) -> ()  [unwired: 2 in, 2 out]
            n1015 = property on="R Scan" class="Bool (strict)"("Val(Sgnl)"=FALSE ("Slew Ready 2")) -> ()  [unwired: 2 in, 2 out]
            n1016 = property on="Y Scan" class="Bool (strict)"("Val(Sgnl)"=FALSE ("Slew Ready 2")) -> ()  [unwired: 2 in, 2 out]
            n1017 = property on="Z Scan" class="Bool (strict)"("Val(Sgnl)"=FALSE ("Slew Ready 2")) -> ()  [unwired: 2 in, 2 out]
            n1018 = property on="R Scan Length SP steps" class="DigNum (strict)"("DisabledEnum"=T1."Enabled" ("Disabled")) -> ()  [unwired: 2 in, 2 out]
            n1019 = property on="Z Scan Velocity SP steps/sec" class="DigNum (strict)"("DisabledEnum"=T1."Enabled" ("Disabled")) -> ()  [unwired: 2 in, 2 out]
            n1020 = property on="X Scan Length SP steps" class="DigNum (strict)"("DisabledEnum"=T1."Enabled" ("Disabled")) -> ()  [unwired: 2 in, 2 out]
            n1021 = property on="Y Scan Selocity SP steps/sec" class="DigNum (strict)"("DisabledEnum"=T1."Enabled" ("Disabled")) -> ()  [unwired: 2 in, 2 out]
            n1022 = property on="R Scan Velocity SP steps/sec" class="DigNum (strict)"("DisabledEnum"=T1."Enabled" ("Disabled")) -> ()  [unwired: 2 in, 2 out]
            n1023 = property on="Y Scan Length SP steps" class="DigNum (strict)"("DisabledEnum"=T1."Enabled" ("Disabled")) -> ()  [unwired: 2 in, 2 out]
            n1024 = property on="Z Scan Length SP steps" class="DigNum (strict)"("DisabledEnum"=T1."Enabled" ("Disabled")) -> ()  [unwired: 2 in, 2 out]
            n1025 = property on="X Scan Velocity SP steps/sec" class="DigNum (strict)"("DisabledEnum"=T1."Enabled" ("Disabled")) -> ()  [unwired: 2 in, 2 out]
            n1026 = property on="Scan Go" class="Bool"("DisabledEnum"=T1."Disabled and Grayed Out" ("Disabled")) -> ()  [unwired: 2 in, 2 out]
            n1027 = property on="Scan Cancel" class="Bool"("DisabledEnum"=T1."Disabled and Grayed Out" ("Disabled")) -> ()  [unwired: 2 in, 2 out]
          }
        }
      }
      event #24 {
        n1028 = event-data() -> ()  [unwired: 1 in, 7 out]
        n1029 = flat-sequence {
          tunnel: [w2066] -> w2045
          tunnel: w2046 -> [w2069]
          tunnel: [w2068] -> w2044
          tunnel: w2047 -> [w2067]
          frame #0 {
            n1030 = property on="Reset X Motor Steps" class="DigNum (strict)"() -> ("Value"=w2070:i32)  [unwired: 2 in, 2 out]
            n1031 = Number To Decimal String(number=w2070) -> (decimal integer string=w2071:string)  [unwired: 1 in]
            n1032 = call "mDrive Send Command.vi"("error in (no error)"=w2069, "Extra"=w2071, "Command"=T2."Set Current Position", "VISA resource name"=w2067) -> ("error out"=w2068:errorcluster, "VISA resource name out"=w2066:refnum<visa-resource-name>)  [unwired: 3 in, 1 out]
          }
        }
        n1033 = flat-sequence {
          tunnel: w2051 -> [w2076]
          tunnel: w2050 -> [w2075]
          tunnel: [w2074] -> w2049
          tunnel: [w2073] -> w2048
          frame #0 {
            n1034 = property on="Reset Y Motor Steps" class="DigNum (strict)"() -> ("Value"=w2077:i32)  [unwired: 2 in, 2 out]
            n1035 = Number To Decimal String(number=w2077) -> (decimal integer string=w2078:string)  [unwired: 1 in]
            n1036 = call "mDrive Send Command.vi"("error in (no error)"=w2075, "Extra"=w2078, "Command"=T2."Set Current Position", "VISA resource name"=w2076) -> ("error out"=w2073:errorcluster, "VISA resource name out"=w2074:refnum<visa-resource-name>)  [unwired: 3 in, 1 out]
          }
        }
        n1037 = flat-sequence {
          tunnel: [w2053] -> w2039
          tunnel: [w2055] -> w2038
          tunnel: w2041 -> [w2054]
          tunnel: w2040 -> [w2052]
          frame #0 {
            n1038 = property on="Reset R Motor Steps" class="DigNum (strict)"() -> ("Value"=w2056:i32)  [unwired: 2 in, 2 out]
            n1039 = Number To Decimal String(number=w2056) -> (decimal integer string=w2057:string)  [unwired: 1 in]
            n1040 = call "mDrive Send Command.vi"("error in (no error)"=w2052, "Extra"=w2057, "Command"=T2."Set Current Position", "VISA resource name"=w2054) -> ("error out"=w2055:errorcluster, "VISA resource name out"=w2053:refnum<visa-resource-name>)  [unwired: 3 in, 1 out]
          }
        }
        n1041 = flat-sequence {
          tunnel: [w2062] -> w2037
          tunnel: [w2061] -> w2036
          tunnel: w2043 -> [w2060]
          tunnel: w2042 -> [w2059]
          frame #0 {
            n1042 = property on="Reset Z Motor Steps" class="DigNum (strict)"() -> ("Value"=w2063:i32)  [unwired: 2 in, 2 out]
            n1043 = Number To Decimal String(number=w2063) -> (decimal integer string=w2064:string)  [unwired: 1 in]
            n1044 = call "mDrive Send Command.vi"("error in (no error)"=w2059, "Extra"=w2064, "Command"=T2."Set Current Position", "VISA resource name"=w2060) -> ("error out"=w2061:errorcluster, "VISA resource name out"=w2062:refnum<visa-resource-name>)  [unwired: 3 in, 1 out]
          }
        }
      }
    }
  }
  n1045 = flat-sequence {
    tunnel: w70 -> [w2084]
    tunnel: w69 -> [w2081]
    frame #0 {
      n1046 = call "mDrive Send Command.vi"("error in (no error)"=w2081, "Command"=T2."Stop", "VISA resource name"=w2084) -> ("error out"=w2082:errorcluster, "VISA resource name out"=w2083:refnum<visa-resource-name>)  [unwired: 4 in, 1 out]
      n1047 = VISA Close(VISA resource name=w2083, error in (no error)=w2082) -> ()  [unwired: 1 out]
    }
  }
  n1048 = flat-sequence {
    tunnel: w97 -> [w2089]
    tunnel: w96 -> [w2086]
    frame #0 {
      n1049 = call "mDrive Send Command.vi"("error in (no error)"=w2086, "Command"=T2."Stop", "VISA resource name"=w2089) -> ("error out"=w2087:errorcluster, "VISA resource name out"=w2088:refnum<visa-resource-name>)  [unwired: 4 in, 1 out]
      n1050 = VISA Close(VISA resource name=w2088, error in (no error)=w2087) -> ()  [unwired: 1 out]
    }
  }
  n1051 = flat-sequence {
    tunnel: w24 -> [w2094]
    tunnel: w23 -> [w2091]
    frame #0 {
      n1052 = call "mDrive Send Command.vi"("error in (no error)"=w2091, "Command"=T2."Stop", "VISA resource name"=w2094) -> ("error out"=w2092:errorcluster, "VISA resource name out"=w2093:refnum<visa-resource-name>)  [unwired: 4 in, 1 out]
      n1053 = VISA Close(VISA resource name=w2093, error in (no error)=w2092) -> ()  [unwired: 1 out]
    }
  }
  n1054 = flat-sequence {
    tunnel: w20 -> [w2099]
    tunnel: w19 -> [w2096]
    frame #0 {
      n1055 = call "mDrive Send Command.vi"("error in (no error)"=w2096, "Command"=T2."Stop", "VISA resource name"=w2099) -> ("error out"=w2097:errorcluster, "VISA resource name out"=w2098:refnum<visa-resource-name>)  [unwired: 4 in, 1 out]
      n1056 = VISA Close(VISA resource name=w2098, error in (no error)=w2097) -> ()  [unwired: 1 out]
    }
  }
  "Y COM PORT" <- w100
  "X COM PORT" <- w75
  "Z COM PORT" <- w62
  "R COM PORT" <- w29
